vi "Main.vi"() -> ()   [LabVIEW 2018]
uses:
  Status.ctl
  Command.ctl
  SECM tip/Control 1.ctl
  SR865/SR865.ctl
  RBD9103/RBD9103.ctl
  GenericDataEvent/GenericEvent.ctl
  Zaber library/Zaber.ctl
  Zaber library/ZaberVariables.ctl
  Exec Action.ctl
  Actions.ctl
  Program Info.ctl
  Zaber library/Stage joystick buttons.ctl
  <vilib>/Analysis/baseanly.llb/Matrix Type of Inverse Matrix.ctl
  SR865/DataChannel.ctl
  <vilib>/Platform/TimedLoop/XDataNode/timing_clust.ctl
  <vilib>/Platform/TimedLoop/XDataNode/nitl_modes.ctl
  <vilib>/Platform/TimedLoop/XDataNode/wakeup.ctl
  <vilib>/DAQmx/write.llb/DAQmx Write (Digital Bool 1Line 1Point).vi
  <vilib>/Analysis/7linalg.llb/Solve Linear Equations (single right hand).vi
  <vilib>/Analysis/baseanly.llb/Solve Linear Equations By Cholesky.vi
  <vilib>/Analysis/baseanly.llb/Real Matrix to Compact Array.vi
  <vilib>/Analysis/baseanly.llb/Real Compact Tri-Matrix Linear Eqs.vi
  <vilib>/DAQmx/create/channels.llb/DAQmx Create Channel (DO-Digital Output).vi
  <vilib>/DAQmx/miscellaneous.llb/DAQmx Fill In Error Info.vi
  <vilib>/Analysis/7linalg.llb/Solve Linear Eqs (General).vi
  <vilib>/Analysis/7linalg.llb/Solve Linear Eqs (Gen, single right hand).vi
  <vilib>/Utility/file.llb/Write Delimited Spreadsheet (DBL).vi
  <vilib>/measure/maresamp.llb/Resample N Pairs of Arrays (single shot).vi
  <vilib>/Platform/TimedLoop/XDataNode/XDataNode.xnode
  <vilib>/Analysis/NI_AALBase.lvlib
  <vilib>/Analysis/NI_AALPro.lvlib
  <vilib>/Platform/TimedLoop/XDataNode/XDNodeRunTimeDep.lvlib
  <vilib>/measure/NI_MAPro.lvlib
panel:
  in  "Pre-scan time, s":dbl
  in  "Landing dwell, s":dbl
  out "MS dwell":bool
  in  "BtnSaveSegLineRecords":bool
  out "relative main end":dbl
  out "relative main start":dbl
  out "segLines":dbl[][](array[numeric])
  out "Current step idx":i32
  out "CC stop":bool
  out "CC start":bool
  out "Strip motion \nposition":dbl
  out "Main motion\nstart position":dbl
  out "Main motion \nend position":dbl
  in  "sample DLADS prediction":string="C:\\Users\\Lab Admin\\Desktop"
  out "Latest step idx":i32
  out "Wait to iterate ?":bool
  out "Iterate ?":bool
  in  "BtnDLADS":bool
  in  "BtnSaveScanConfig":bool
  in  "Com error":bool
  out "Z Zaber":T1={"Serial port handle"="", "Axis"="", "Controller #"=0, "Min position"=0.0, "Max position"=0.0, "Min velocity"=0.0, "Max velocity"=0.0, "Firmware"="", "Device ID"=0, "Variable event"=refnum, "Variable ref"=refnum, "Resolution, usteps/step"=0, "Serial port semaphore"=refnum, "Joystick buttons"={"MinDir"=1, "MaxDir"=2, "MedSpeed"=5, "HighSpeed"=6}} {"Joystick buttons"."HighSpeed" min=1 max=25 step=1; "Joystick buttons"."MedSpeed" min=1 max=25 step=1; "Joystick buttons"."MaxDir" min=1 max=25 step=1; "Joystick buttons"."MinDir" min=1 max=25 step=1}
  out "Loop time":u32
  out "BtnLoopWasLate":bool caption="Loop was late"
  out "MS ever Trig?":bool=TRUE
  out "MS start":u32=518275974
  out "LineMotion":bool=TRUE caption="Line motion"
  out "LineNumber":u32=2
  out "dt":dbl
  out "t0":dbl
  out "MotionStartTime":u32 caption="Line start time"
  out "Keyence":T4={"Serial port sem"=refnum, "Serial port handle"="", "Baud rate"=9600}
  in  "Keyence COM port":refnum<visa-resource-name>="COM4"
  out "SICM tip":refnum<vi>
  out "Stop tune SICM":refnum<user-event>
  out "RBD9103":T5
  in  "RBD9103 COM":refnum<visa-resource-name>="COM4"
  in  "SR865":refnum<visa-resource-name>="USB0::0xB506::0x2000::003539::INSTR"
  out "SR865":T6
  in  "TabMethods":T7(tab)=enum."Shear force sensor"
  in  "TabPlanes":enum32{"Simple plane", "3 point plane"}(tab)
  in  "SPZEndPosition":dbl=5.0 caption="Z end" min=0.0 max=25.0 format="%#.4f"
  out "PlaneZ3":dbl caption="Z3" min=0.0 max=25.0 format="%#.4f"
  out "PlaneY3":dbl caption="Y3" min=0.0 max=25.0 format="%#.4f"
  out "PlaneX3":dbl=20.0000235 caption="X3" min=0.0 max=25.0 format="%#.4f"
  out "PlaneZ2":dbl caption="Z2" min=0.0 max=25.0 format="%#.4f"
  out "PlaneY2":dbl=10.00001175 caption="Y2" min=0.0 max=25.0 format="%#.4f"
  out "PlaneX2":dbl caption="X2" min=0.0 max=25.0 format="%#.4f"
  out "PlaneZ1":dbl caption="Z1" min=0.0 max=25.0 format="%#.4f"
  out "PlaneY1":dbl caption="Y1" min=0.0 max=25.0 format="%#.4f"
  out "PlaneX1":dbl caption="X1" min=0.0 max=25.0 format="%#.4f"
  in  "BtnPlaneSetPoint3":bool caption="Set Z out position"
  in  "BtnPlaneSetPoint1":bool
  in  "BtnPlaneSetPoint2":bool caption="Set Z out position"
  out "PlaneZx":dbl caption="Zx" min=0.0 max=25.0 format="%#.4f"
  out "PlaneZy":dbl caption="Zy" min=0.0 max=25.0 format="%#.4f"
  in  "BtnPZStepType":bool caption="Z step type"
  out "PZJumps":u32=600 caption="Z jumps" min=1
  out "PZJump":u32 caption="Z jump"
  out "PZRealStep":dbl=0.0049999802083333334 caption="Z real step" format="%#.4f"
  out "PZStepTimeRb":dbl=0.03399378902730266 caption="Z step time, s" format="%#.1f"
  out "Distance":dbl=2257.881405072176 caption="Distance, um" format="%#.1f"
  out "StartDistance":dbl caption="Start distance, um" format="%#.1f"
  out "MoveDistance":dbl caption="Move distance, um" format="%#.1f"
  out "RealMoveDistance":dbl caption="Real move distance, um" format="%#.1f"
  in  "ZFactor":dbl=20.0 caption="Sensor/Z motion factor" min=0.0 max=25.0 format="%#.4f"
  in  "ZMinToMoveDistanceancy":dbl=5.0 caption="Min to move distance, um" min=0.0 format="%#.4f"
  in  "ZMaxToMoveDistance":dbl=50.0 caption="Max to move distance, um" min=0.0 format="%#.4f"
  in  "BtnShearForceTune":bool
  out "SFMWorkingLevel":dbl=7.0 caption="Working level, V" min=0.0 max=25.0 step=0.01 format="%#.4f"
  in  "SFMShiftFromAirLevel":dbl=-0.5 caption="Shift from Air level, V" min=0.0 max=25.0 step=0.01 format="%#.4f"
  in  "SFMSlope":dbl=-0.007 caption="Slope, mm/V" min=0.0 max=25.0 step=0.01 format="%#.4f"
  in  "SFMAirErrorLevel":dbl=0.05 caption="Air error level, V" min=0.0 max=25.0 step=0.01 format="%#.4f"
  out "SFMAirError":bool caption="Air level changed"
  in  "SFMLoopTime":i32=10 caption="Loop time, ms"
  out "CurrentAirLevel":dbl=7.198980893447915 caption="Current air level, V" format="%0.2f"
  in  "SFMStayRange":dbl=0.01 caption="Stay range, V"
  out "ShF loop time":u32
  out "Amp dead time":u32
  out "Read position":u32
  in  "SIMStayRange":dbl=0.01 caption="Stay range, V"
  out "BtnSIMLoopWasLate":bool caption="Loop was late"
  out "SIMCurrentLevel":dbl=7.198980893447915 caption="Current air level, V" format="%0.4g"
  in  "SIMLoopTime":i32=10 caption="Loop time, ms" format="%.4g"
  out "SIMAirError":bool caption="Air error"
  in  "SIMAirErrorLevel":dbl=0.05 caption="Air error level, V" min=0.0 max=25.0 step=0.01 format="%#.4g"
  in  "SIMAirLevelSp":dbl=7.22 caption="Air level, V" min=0.0 max=25.0 step=0.01 format="%#.4g"
  in  "SIMWorkingLevel":dbl=7.0 caption="Working level,V" min=0.0 max=25.0 step=0.01 format="%#.4g"
  out "Position, mm":dbl
  out "PositionRb":dbl caption="Position, mm"
  out "Calculated position":dbl
  out "Value, nA":dbl
  out "LineTimeInSec":dbl=20.396273416381593 caption="Line time, s" format="%#.4f"
  out "LineError":dbl=396.27341638159305 caption="Line error, um" format="%#.1f"
  out "LineTimeError":dbl=0.3962734163815931 caption="Line time error, s"
  out "LineStraightTime":dbl=20.0 caption="Line straight time, s"
  in  "ZStep":dbl=0.005 caption="Z step, mm" min=1e-07 max=25.0 step=0.01 format="%#.4f"
  out "RunRef":refnum<vi>
  out "Dialog3StagesRef":refnum<vi>
  in  "Call type":enum16{"Dynamic", "Static"}(ring)=enum."Static"
  out "Stop tune ShFrc":refnum<user-event>
  out "Tune ShFrc":refnum<vi>
  in  "Baud rate (9600 or 115200)":u32=9600
  in  "Z stage":refnum<visa-resource-name>="COM7"
  in  "X&Y stages":T8="COM6"
  in  "BtnSaveZToFile":bool=TRUE
  in  "BtnZ+":bool
  in  "BtnZ-":bool
  out "ProfilePlot":dbl[][](graph) caption="Profile"
  out "ZPositionPlot":cluster{cluster{dbl, dbl}[]}[](graph) caption="Z position"
  in  "LineZData":cluster{cluster{dbl, dbl}[]}[](array[cluster])=[{[]}, {[]}, {[]}]
  out "Profile array":cluster{dbl[], dbl[]}[](array[cluster])
  in  "Method":T9(ring)=enum."3 point plane"
  in  "BtnMeasurementPause":bool
  in  "BtnSave":bool
  in  "Command":T10=enum."None"
  in  "Status":T11
  out "StripStepRb":dbl caption="Strip step" format="%#.4f"
  out "StripLineRb":u32 caption="Strip line"
  in  "StripLines":u32=2 caption="Strip lines" min=1
  out "YStageType":enum16{"Main motion", "Strip motion"}(ring)=enum."Strip motion" caption="Type motion"
  in  "XStageType":enum16{"Main motion", "Strip motion"}(ring) caption="Type"
  out "ZOutPosition":dbl=9.67997175 caption="Z out" format="%#.4f"
  in  "BtnSetZOutPosition":bool caption="Set Z out position"
  out "ZStartPosition":dbl=9.67997175 caption="Z start" min=0.0 max=25.0 format="%#.4f"
  in  "BtnMeasurement":bool
  in  "BtnSetZStartPosition":bool
  in  "BtnExit":bool
  out "LineTimeInMin":dbl=0.33993789027302657 caption="Line time, min" format="%#.3f"
  in  "MSDwellTimeInSec":dbl=15.0 caption="QTOF ready, s" format="%#.1f"
  in  "YEndPosition":dbl=7.0 caption="End  position, mm" min=0.0 max=25.40003175 format="%#.4f"
  in  "YStartPosition":dbl=5.0 caption="Start position, mm" min=0.0 max=25.40003175 format="%#.4f"
  in  "Velocity":dbl=0.020091796874999998 caption="Velocity, mm/s" min=0.000446484375 max=3.5 format="%#.4g"
  in  "XEndPosition":dbl=20.0 caption="End position, mm" min=0.0 max=50.800015875 format="%#.4f"
  in  "XStartPosition":dbl=15.0 caption="Start position, mm" min=0.0 max=50.800015875 format="%#.4f"
  out "Current Time":timestamp format="%<%I:%M:%S %p>T"
  # "X stage"
  # "Z stage"
  # "Y stage"
  # "Main motion"
  # "Strip motion"
  # "Timing"
  # "Keyence reading time 50 ms ; 115200 bod"
  # "doesn't work in Line"
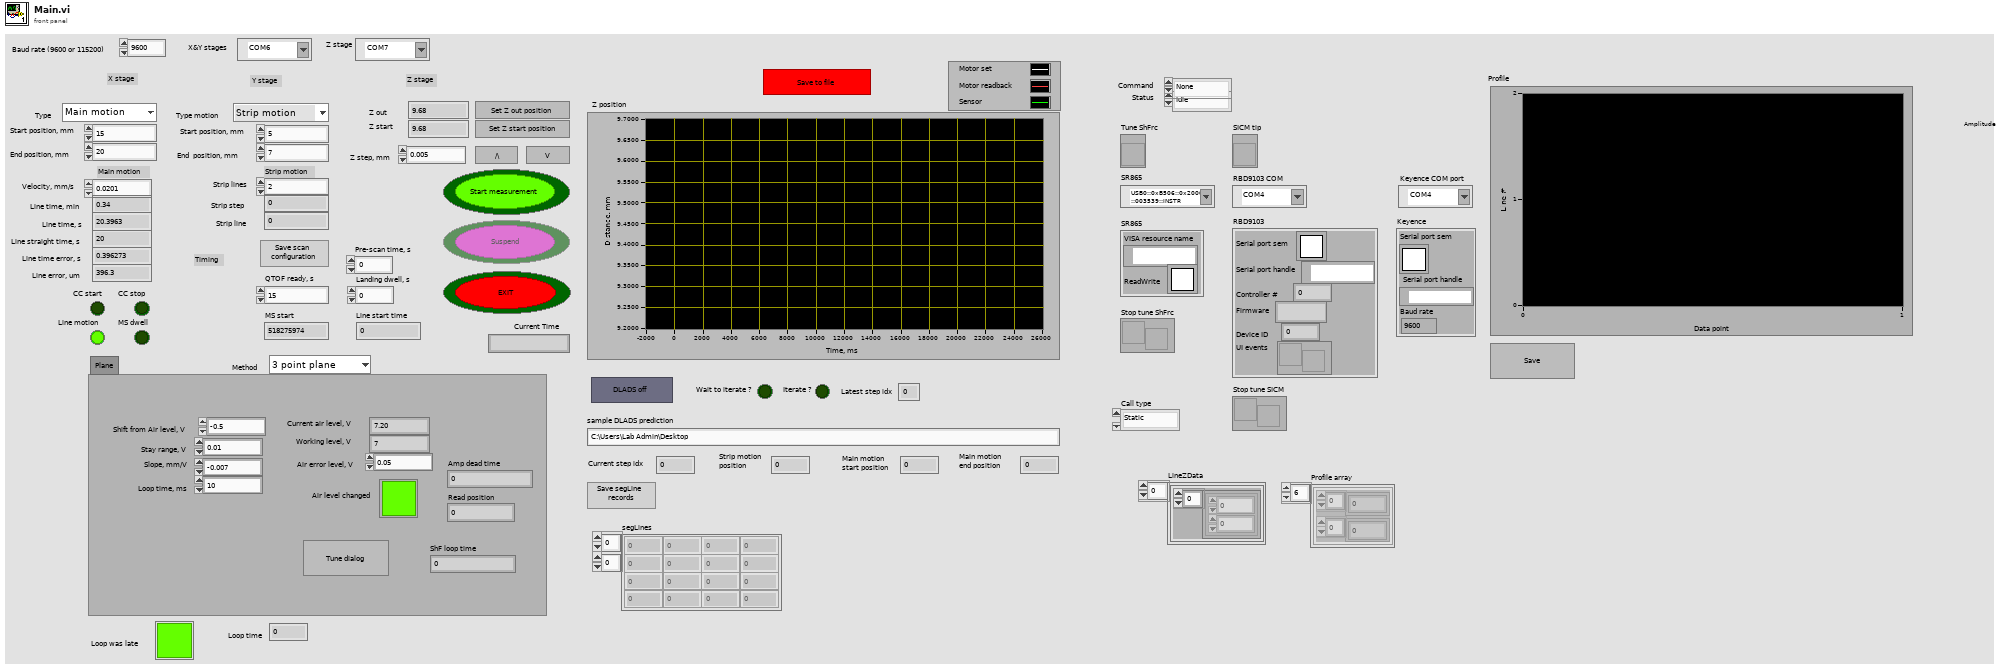
[diagram p1: front panel]
types:
  T1 = typedef "Zaber.ctl" = cluster{"Serial port handle":refnum<visa-resource-name>, "Axis":string, "Controller #":u8, "Min position":dbl, "Max position":dbl, "Min velocity":dbl, "Max velocity":dbl, "Firmware":string, "Device ID":i32, "Variable event":T2, "Variable ref":refnum<data-value>, "Resolution, usteps/step":i32, "Serial port semaphore":T3, "Joystick buttons":cluster{"MinDir":i32, "MaxDir":i32, "MedSpeed":i32, "HighSpeed":i32}}
  T2 = typedef "GenericEvent.ctl" = refnum<user-event>
  T3 = typedef "Semaphore RefNum" = refnum<k1>
  T4 = cluster{"Serial port sem":T3, "Serial port handle":refnum<visa-resource-name>, "Baud rate":u32}
  T5 = typedef "RBD9103.ctl" = cluster{"Serial port sem":T3, "Serial port handle":refnum<visa-resource-name>, "Controller #":u8, "Firmware":string, "Device ID":i32, "UI events":T2}
  T6 = typedef "SR865.ctl" = cluster{"VISA resource name":refnum<visa-resource-name>, "ReadWrite":T3}
  T7 = enum32{"Plane", "Keyence sensor", "Shear force sensor", "SICM sensor"}
  T8 = typedef "Control 1.ctl" = refnum<visa-resource-name>
  T9 = enum16{"Simple plane", "3 point plane", "Keyence sensor", "Shear force sensor", "SICM sensor", "Surface image by Keyence"}
  T10 = typedef "Command.ctl" = enum16{"Start", "Suspend", "Resume", "Stop", "Finish", "None"}
  T11 = typedef "Status.ctl" = enum16{"Idle", "Working", "Pause", "Stopping"}
  T12 = typedef "Program Info.ctl" = cluster{"Placeholder":bool}
  T13 = typedef "Exec Action.ctl" = cluster{"Action":T14, "1":bool, "2":bool, "3":bool}
  T14 = typedef "Actions.ctl" = enum16{"SW Init", "HW Init - Zaber", "HW Init - DO", "Init Asynch Vis", "Set Motion Params", "Set Zout Pos", "Set Zstart Pos", "Step Z", "Method close - Shear force", "Method close - SICM", "Method close - Keyence", "Method UI and HW init", "Tune Shear Force", "Plane Set Point 1", "Plane Set Point 2", "Plane Set Point 3", "Calculate Plane", "Scan UI", "Scan Ctrl", "Handle DLADS", "XY and Sensor Init", "Z Init", "MS Trig", "Line Motion", "Z Exit Ctrl", "MS Complete", "Pause Check Ctrl", "Shift Data", "Plot Profile", "Save Scan Config", "Save Profile Text File", "Wait (ms)", "Get Time", "HW Close - Zaber", "HW Close - DO", "Error", "Exit", "Shutdown Ctrl"}
  T15 = enum8{"Enabled", "Disabled", "Disabled and Grayed Out"}
  T16 = enum32{"Invalid", "Standard", "Closed", "Hidden", "Minimized", "Maximized"}
  T17 = typedef "NI_AALBase.lvlib/Matrix Type of Inverse Matrix.ctl" = enum32{"General", "Positive Definite", "Lower Triangular", "Upper Triangular"}
  T18 = typedef "XDNodeRunTimeDep.lvlib/timing_clust.ctl" = cluster{"Expected End [f-1]":u64, "Actual End [f-1]":u64, "Finished Late? [f-1]":bool, "Expected End [i-1]":u64, "Actual End [i-1]":u64, "Finished Late? [i-1]":bool, "Expected Start [i]":u64, "Actual Start [i]":u64, "Expected Start [f]":u64, "Actual Start [f]":u64, "Source Name":string, "Structure Name":string, "Period":i64, "Deadline":i64, "Offset":i64, "Start":i64, "Priority":i32, "Timeout":i32, "Mode":T19, "Wakeup Reason":T20, "Error":errorcluster, "Source Type":string, "Secondary Source Type":string, "Global End Time":u64, "Global Start Time":u64, "Frame Duration":u64, "Iteration Duration":u64, "Assigned CPU":i32, "I/O Scan Engine Mode":u32}
  T19 = typedef "XDNodeRunTimeDep.lvlib/nitl_modes.ctl" = enum32{"No Change", "Process missed periods, maintain original phase", "Discard missed periods, maintain original phase", "Process missed periods, ignore original phase", "Discard missed periods, ignore original phase"}
  T20 = typedef "XDNodeRunTimeDep.lvlib/wakeup.ctl" = enum32{"Normal", "Aborted", "Asynchronous wakeup", "Timing source error", "Timed loop error", "Timeout"}
  T21 = enum16{"open", "replace", "create", "open or create", "replace or create", "replace or create with confirmation"}
  T22 = typedef "Stage joystick buttons.ctl" = cluster{"MinDir":i32, "MaxDir":i32, "MedSpeed":i32, "HighSpeed":i32}
  T23 = typedef "Joystick event.ctl" = refnum<user-event>
  T24 = typedef "DataChannel.ctl" = u16
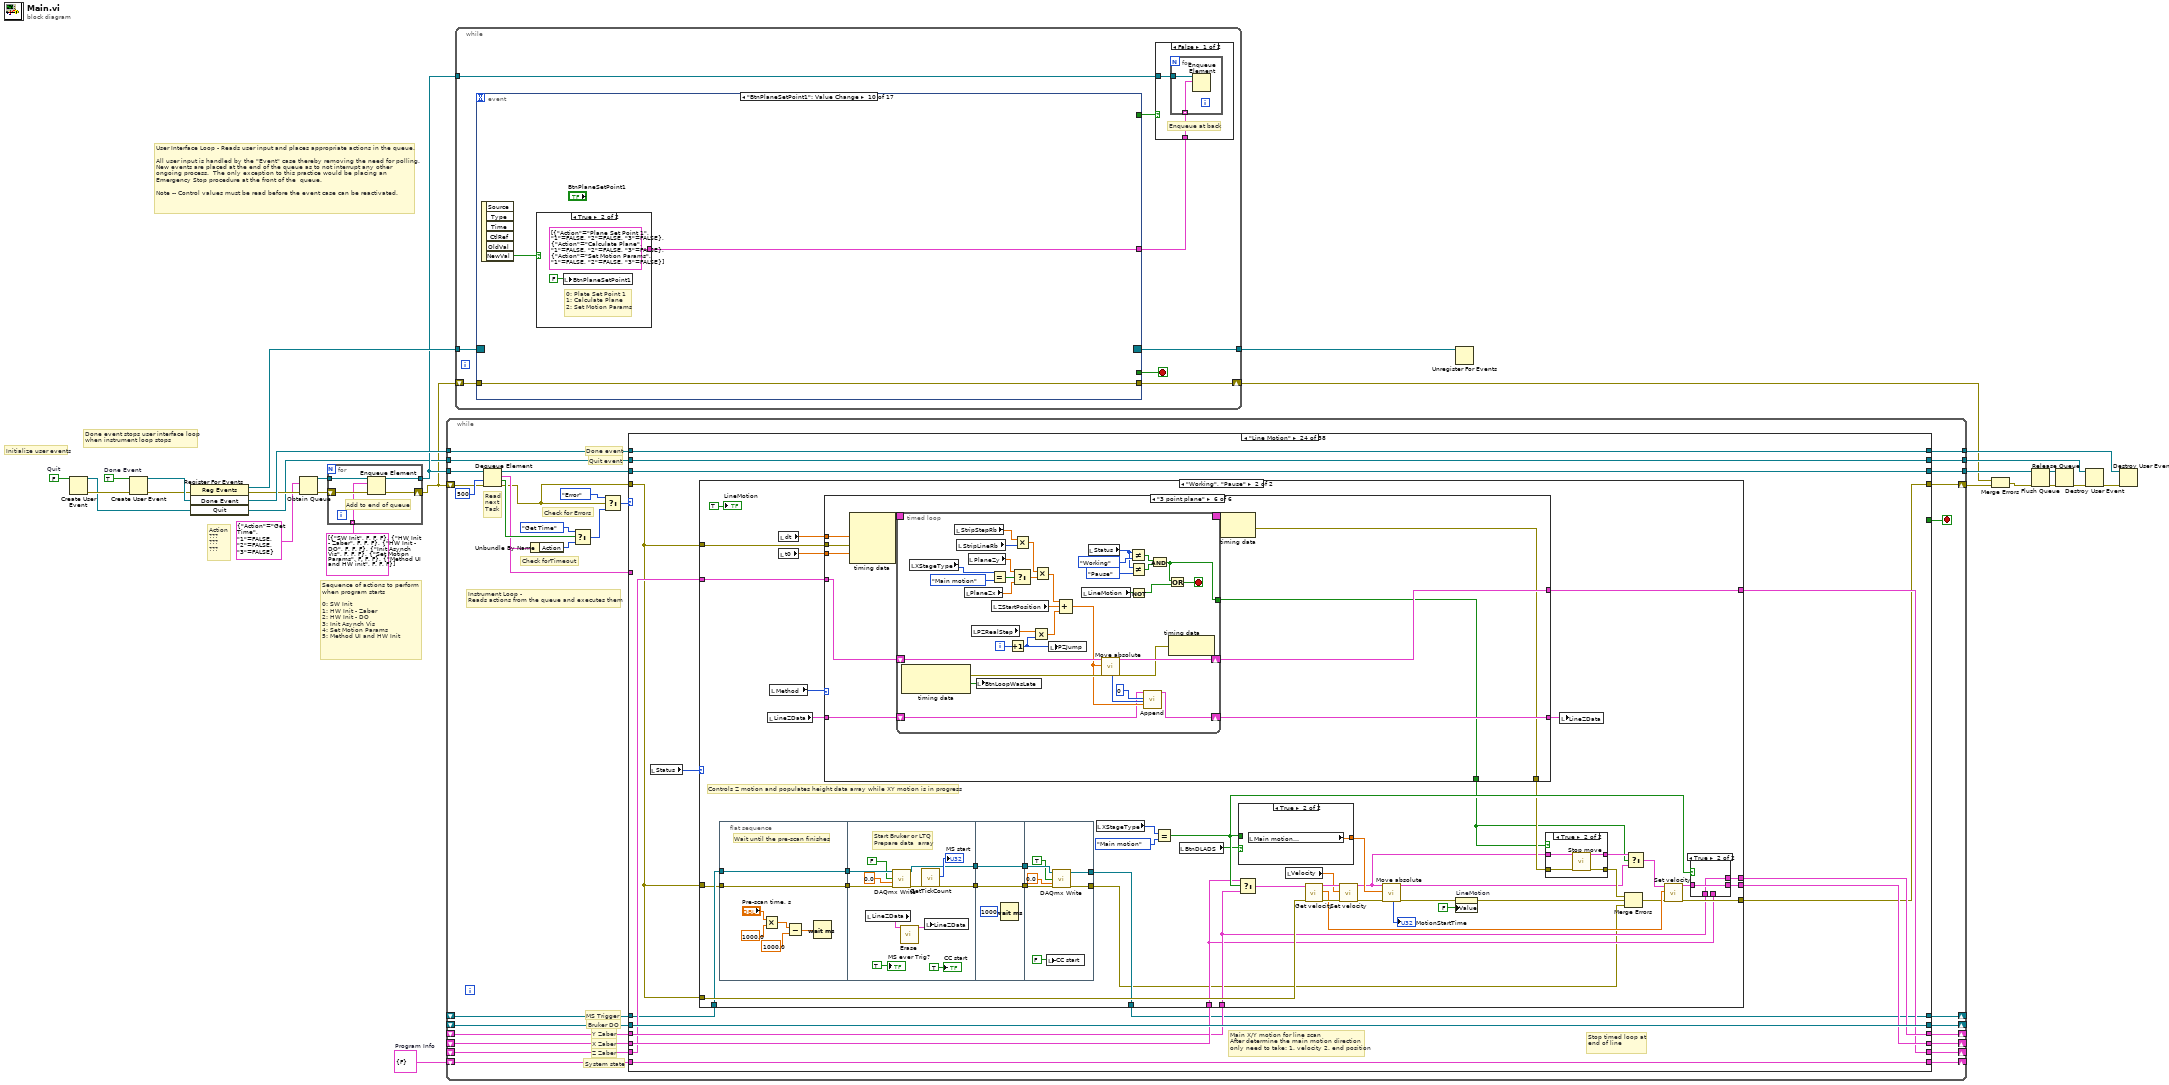
[diagram p0: block diagram]
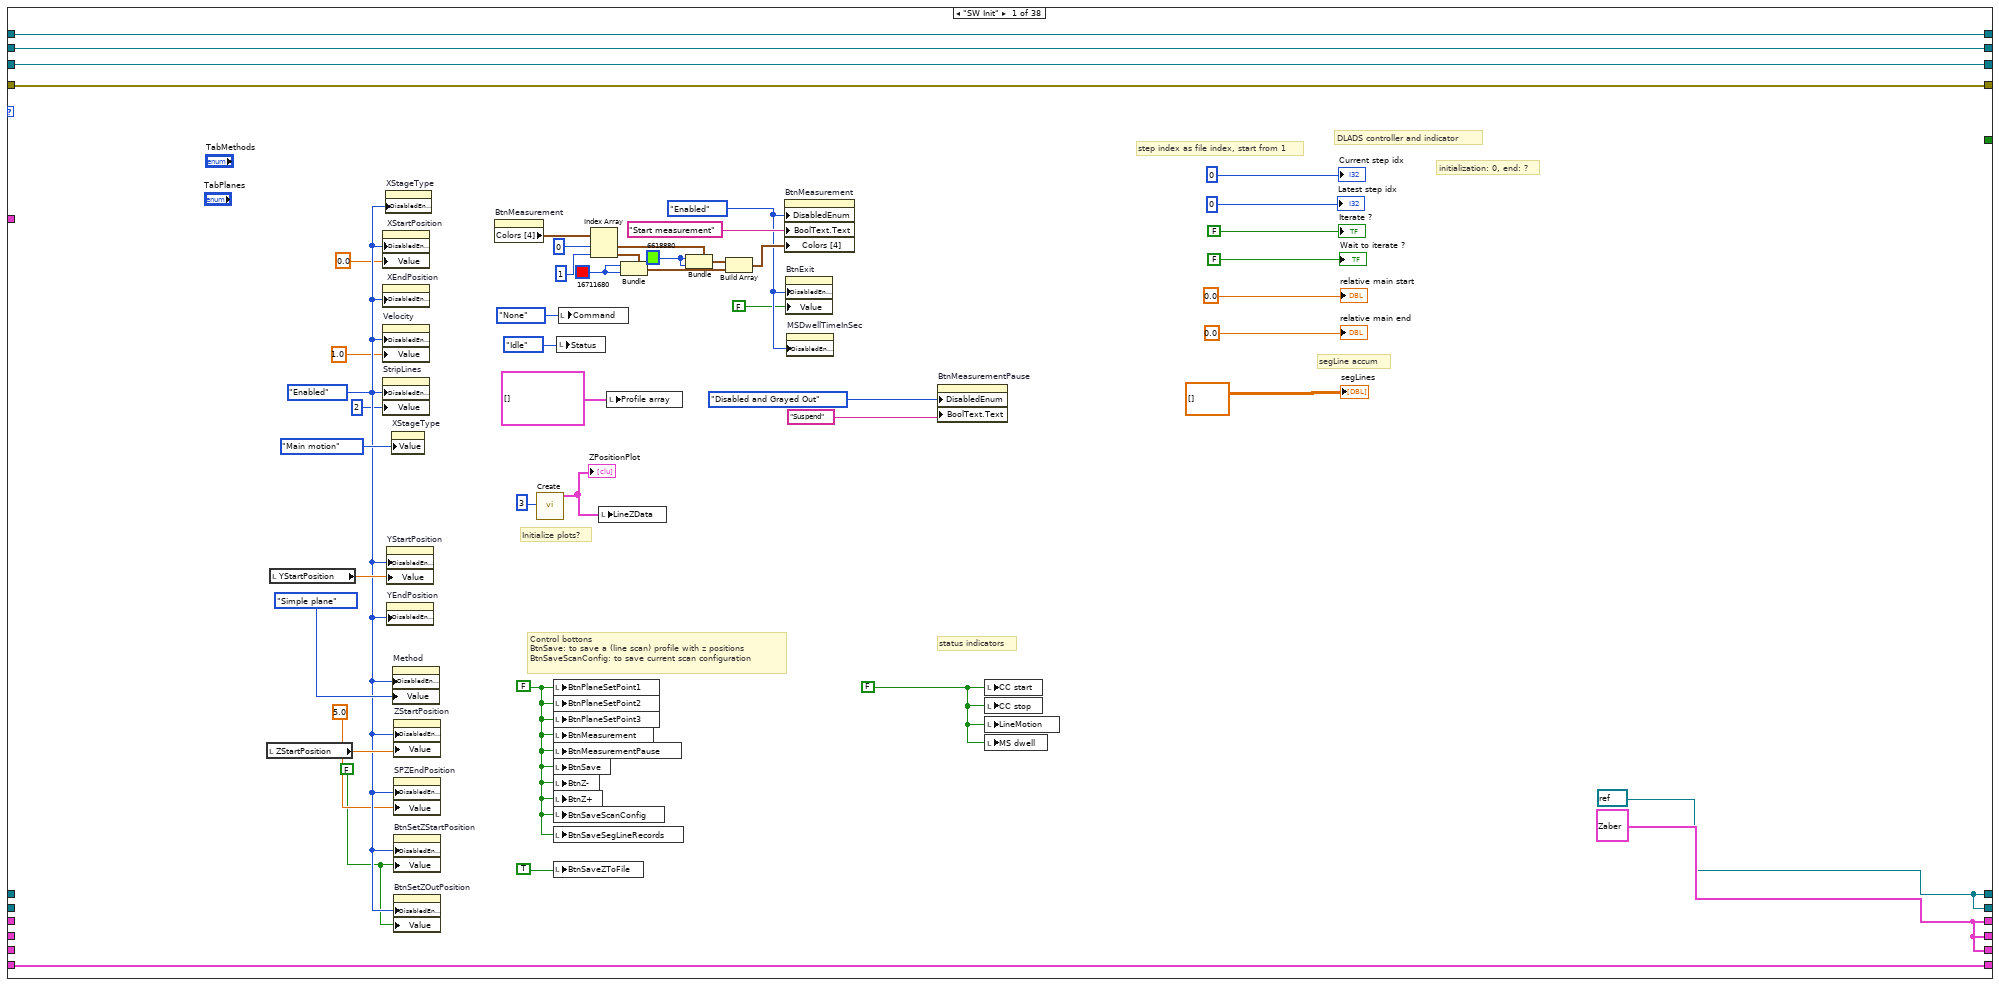
[diagram p2: hidden frame]
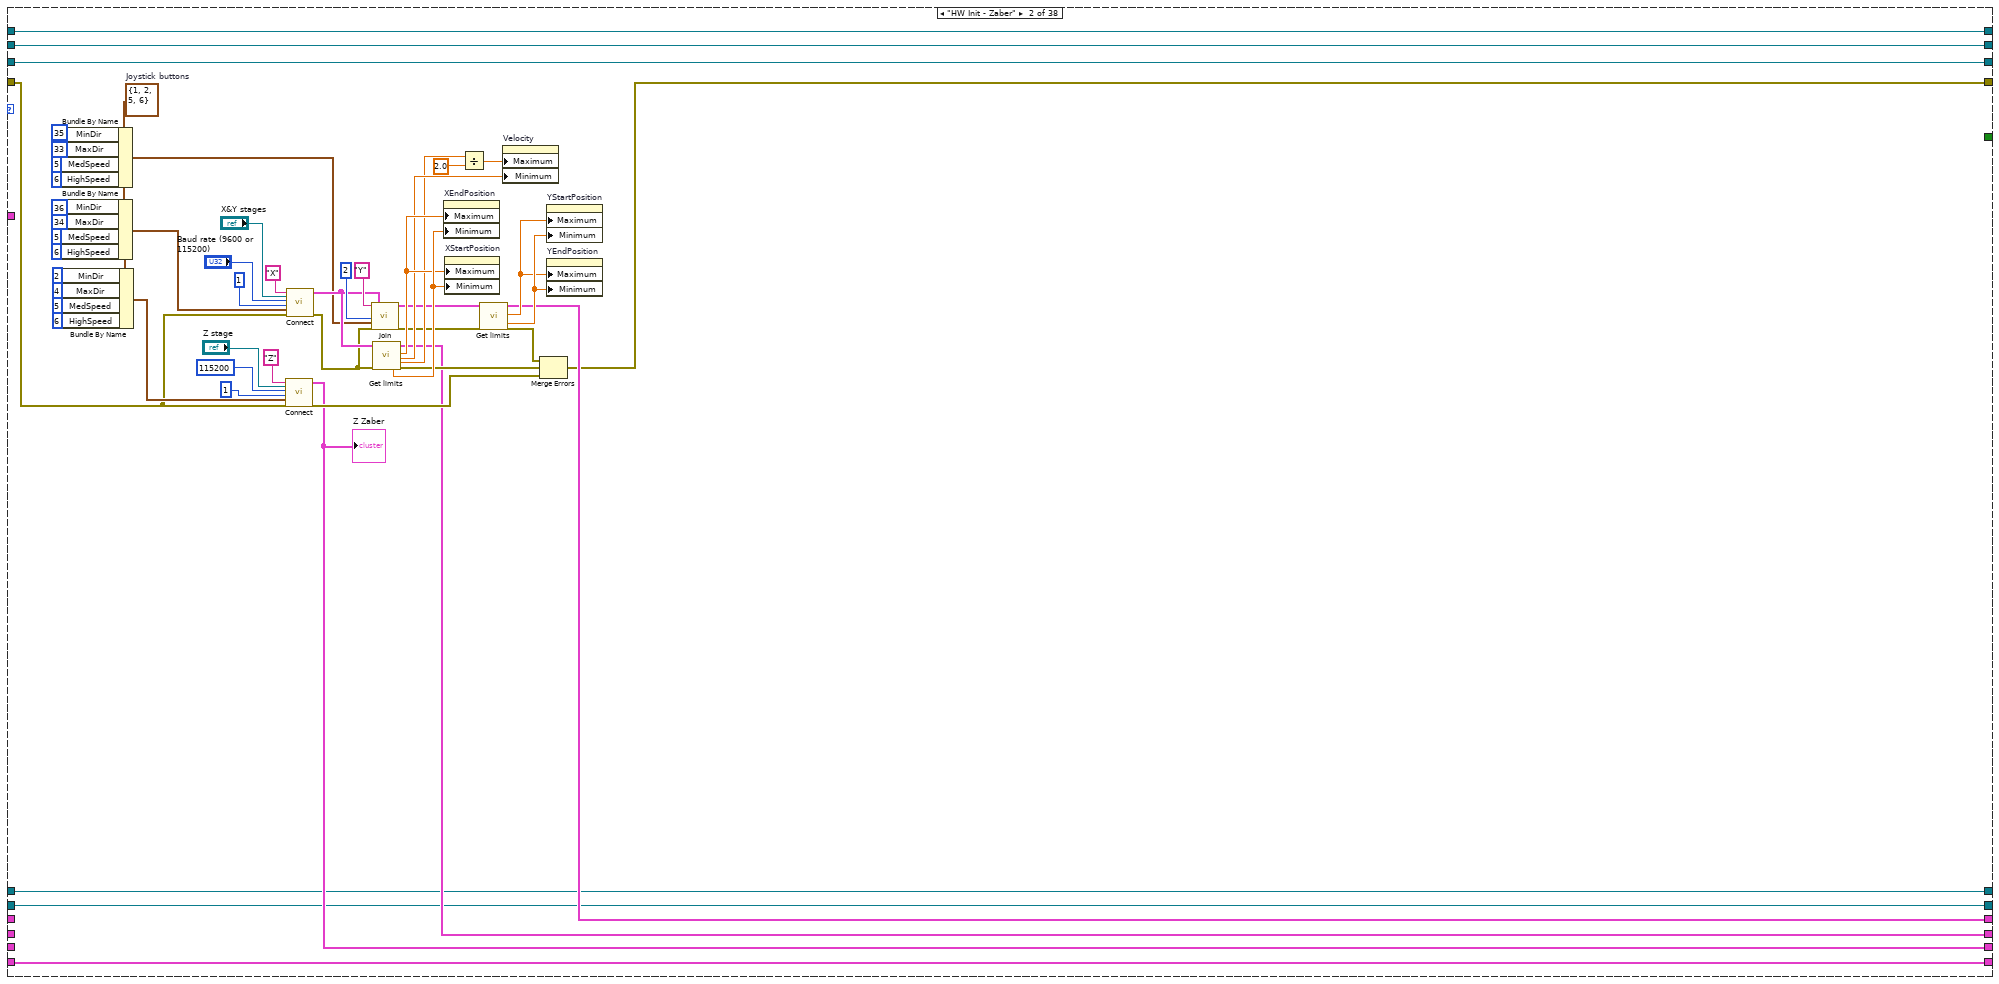
[diagram p3: hidden frame]
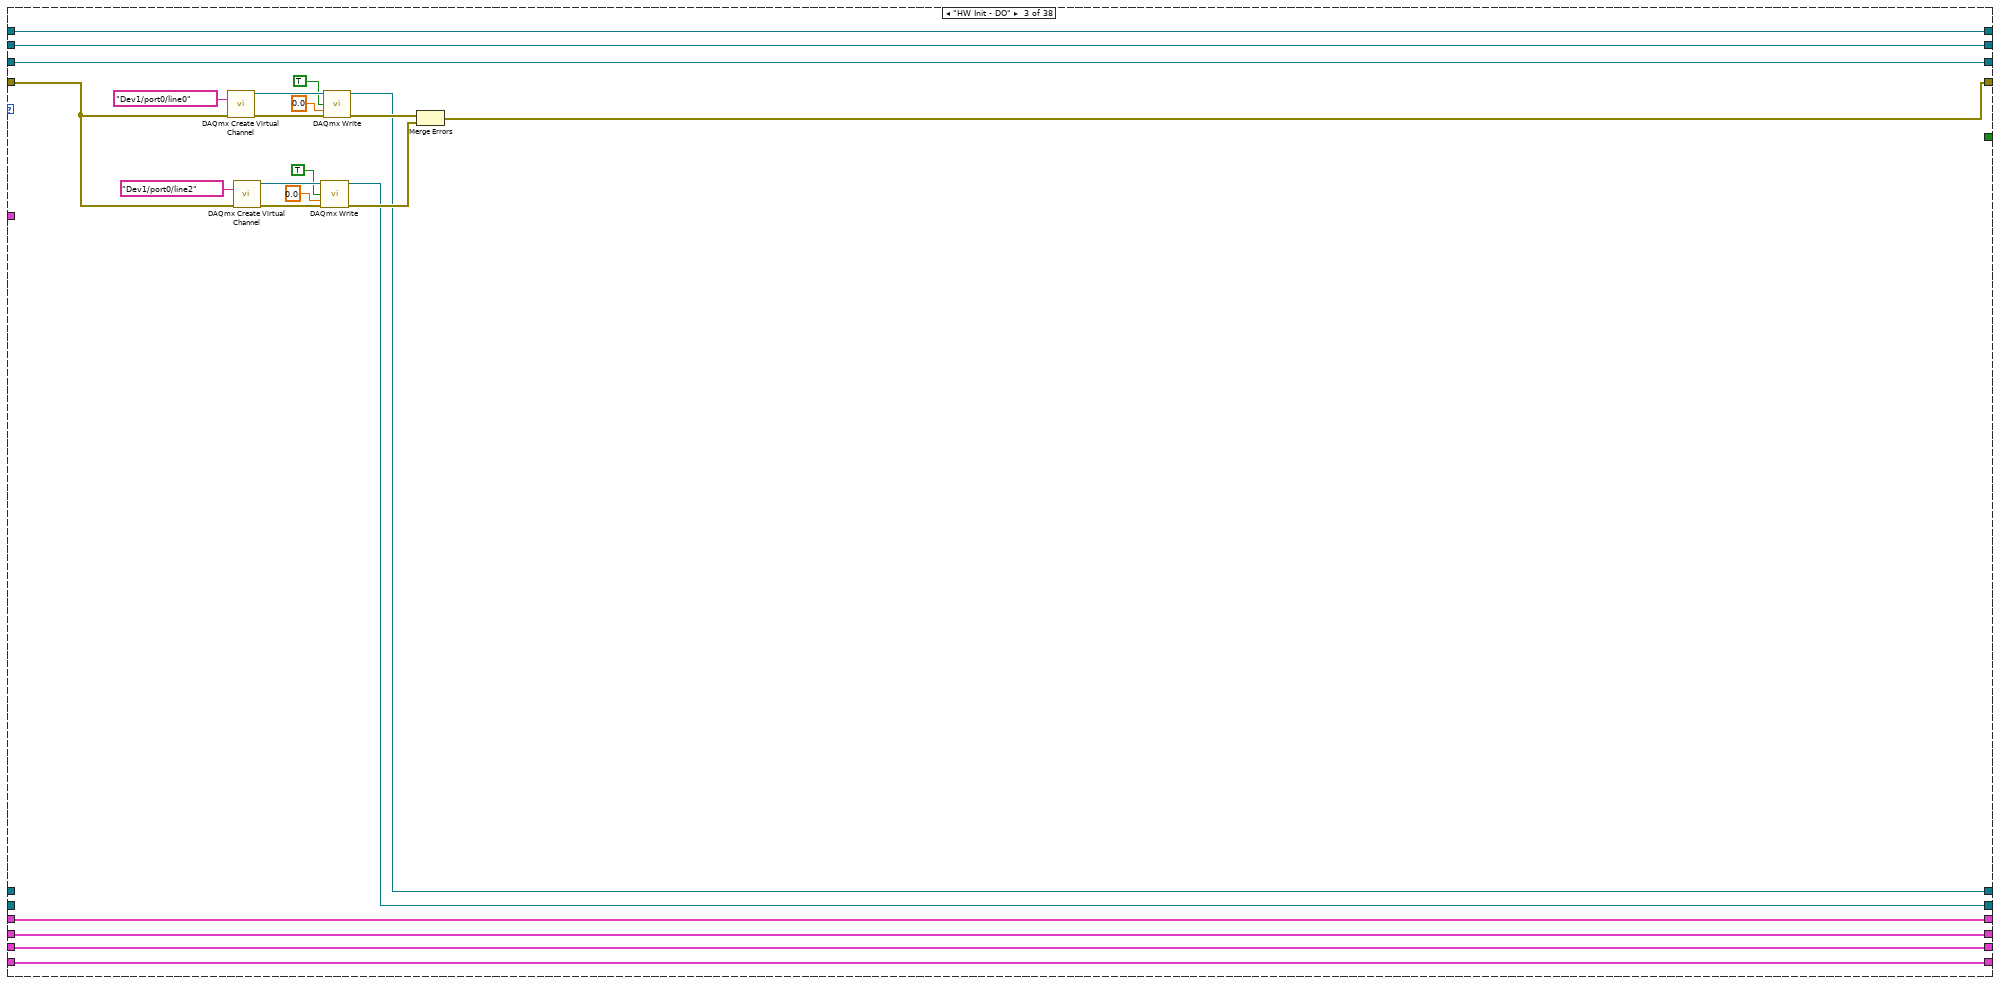
[diagram p4: hidden frame]
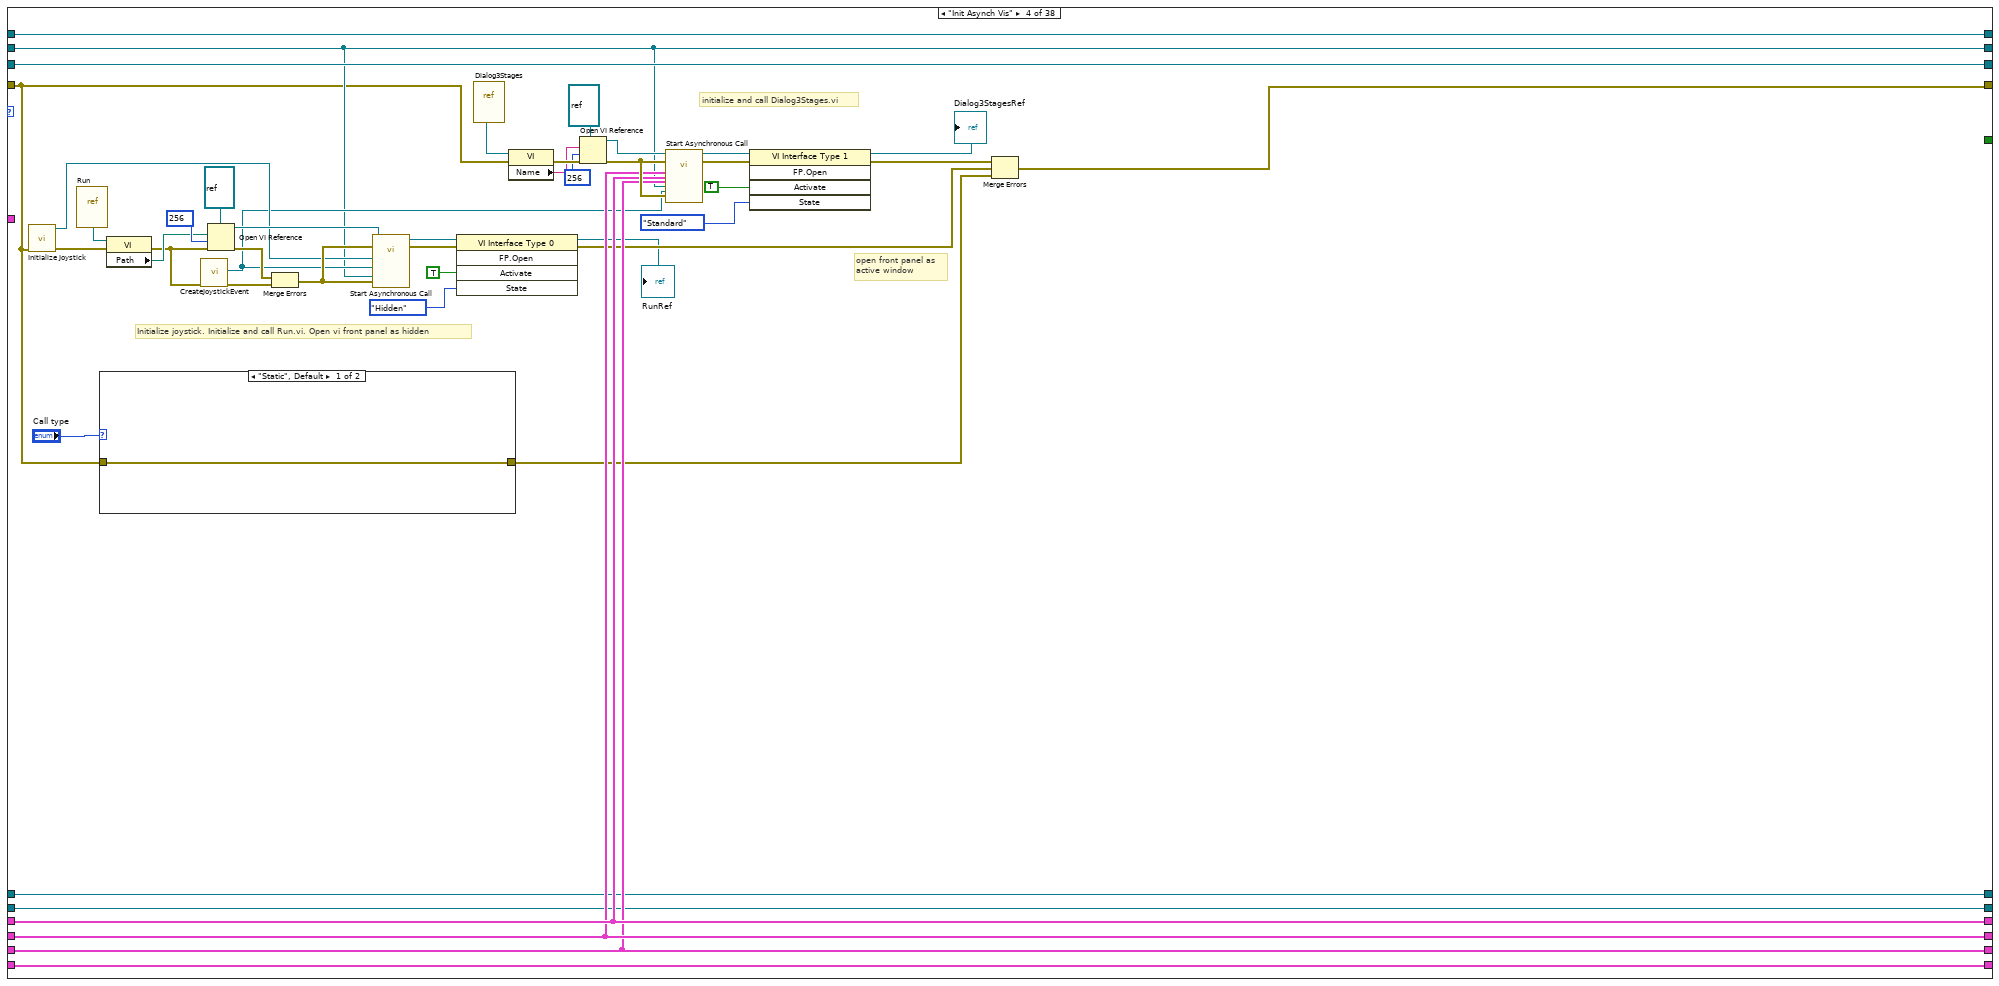
[diagram p5: hidden frame]
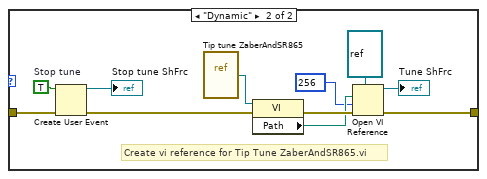
[diagram p6: hidden frame]
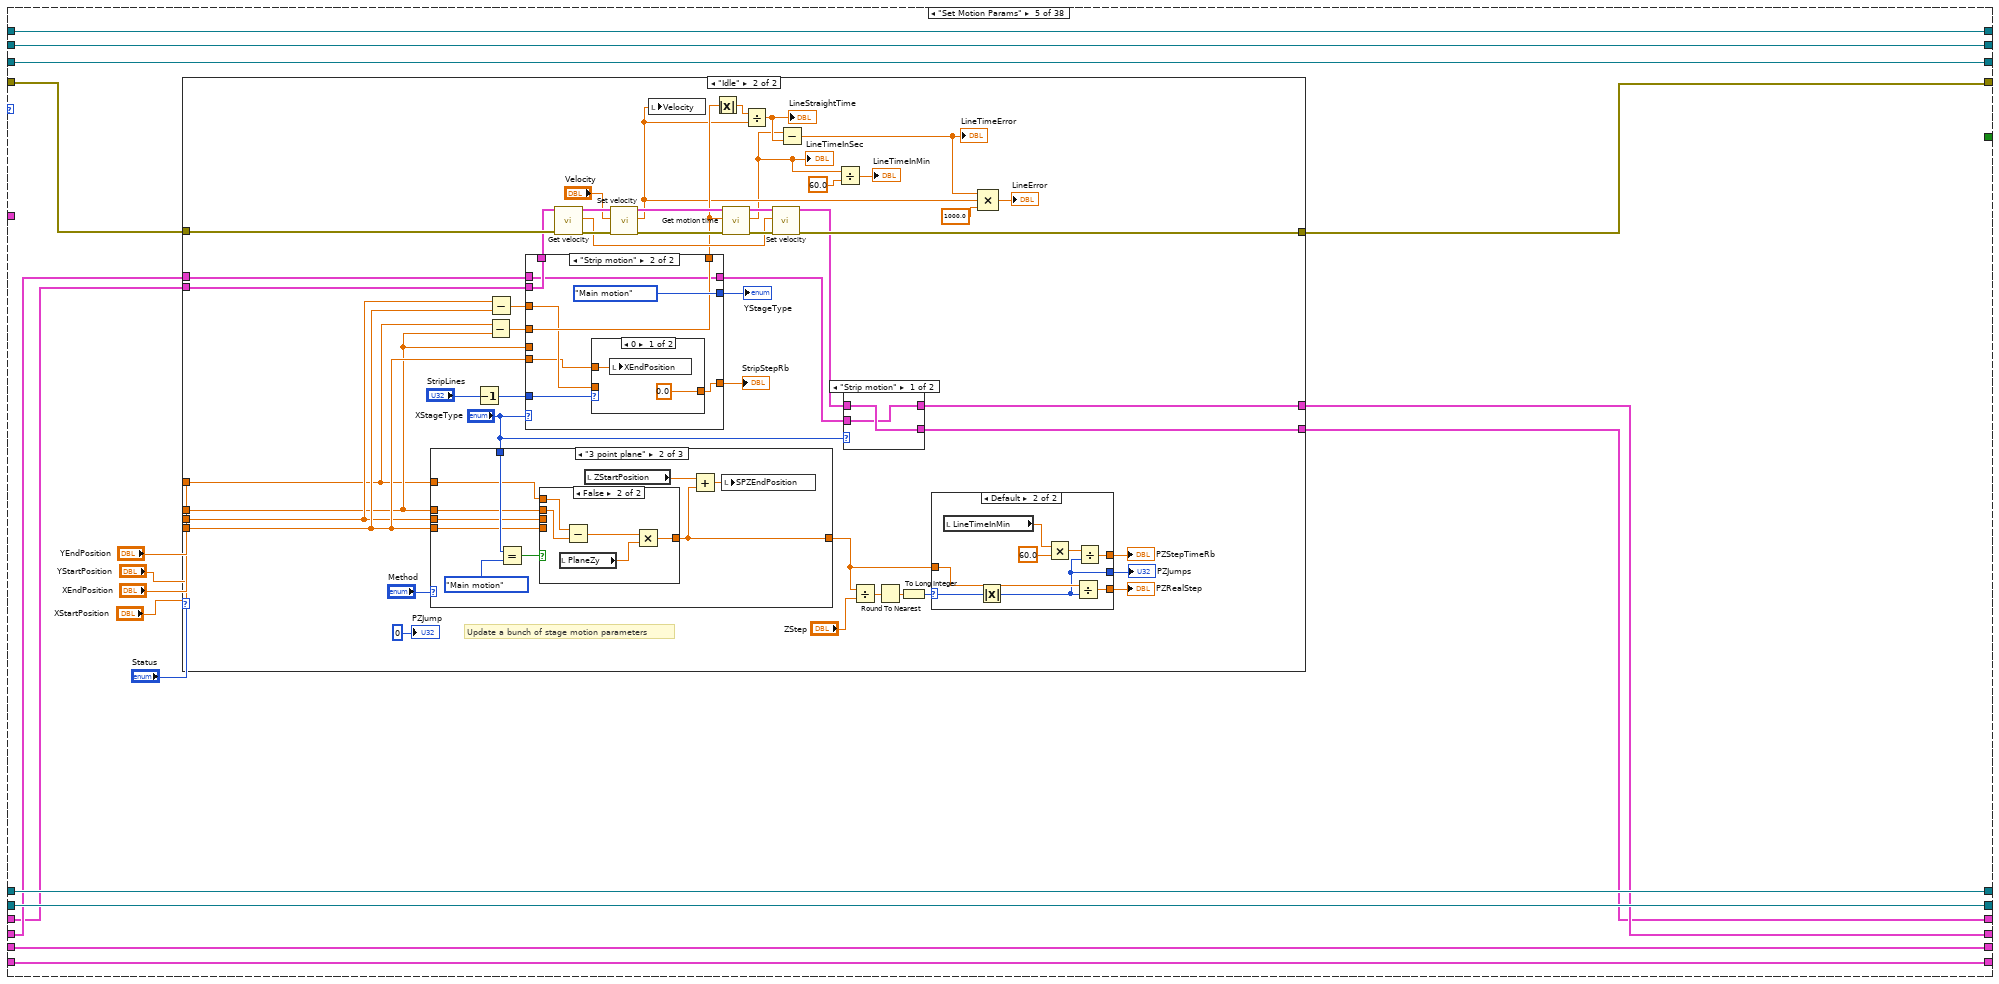
[diagram p7: hidden frame]
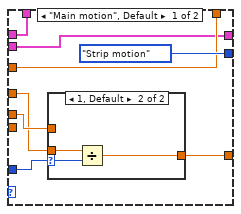
[diagram p10: hidden frame]
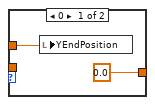
[diagram p11: hidden frame]
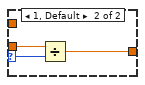
[diagram p12: hidden frame]
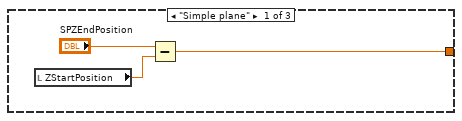
[diagram p13: hidden frame]
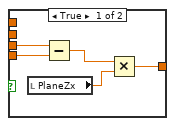
[diagram p14: hidden frame]
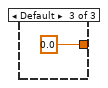
[diagram p15: hidden frame]
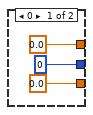
[diagram p16: hidden frame]
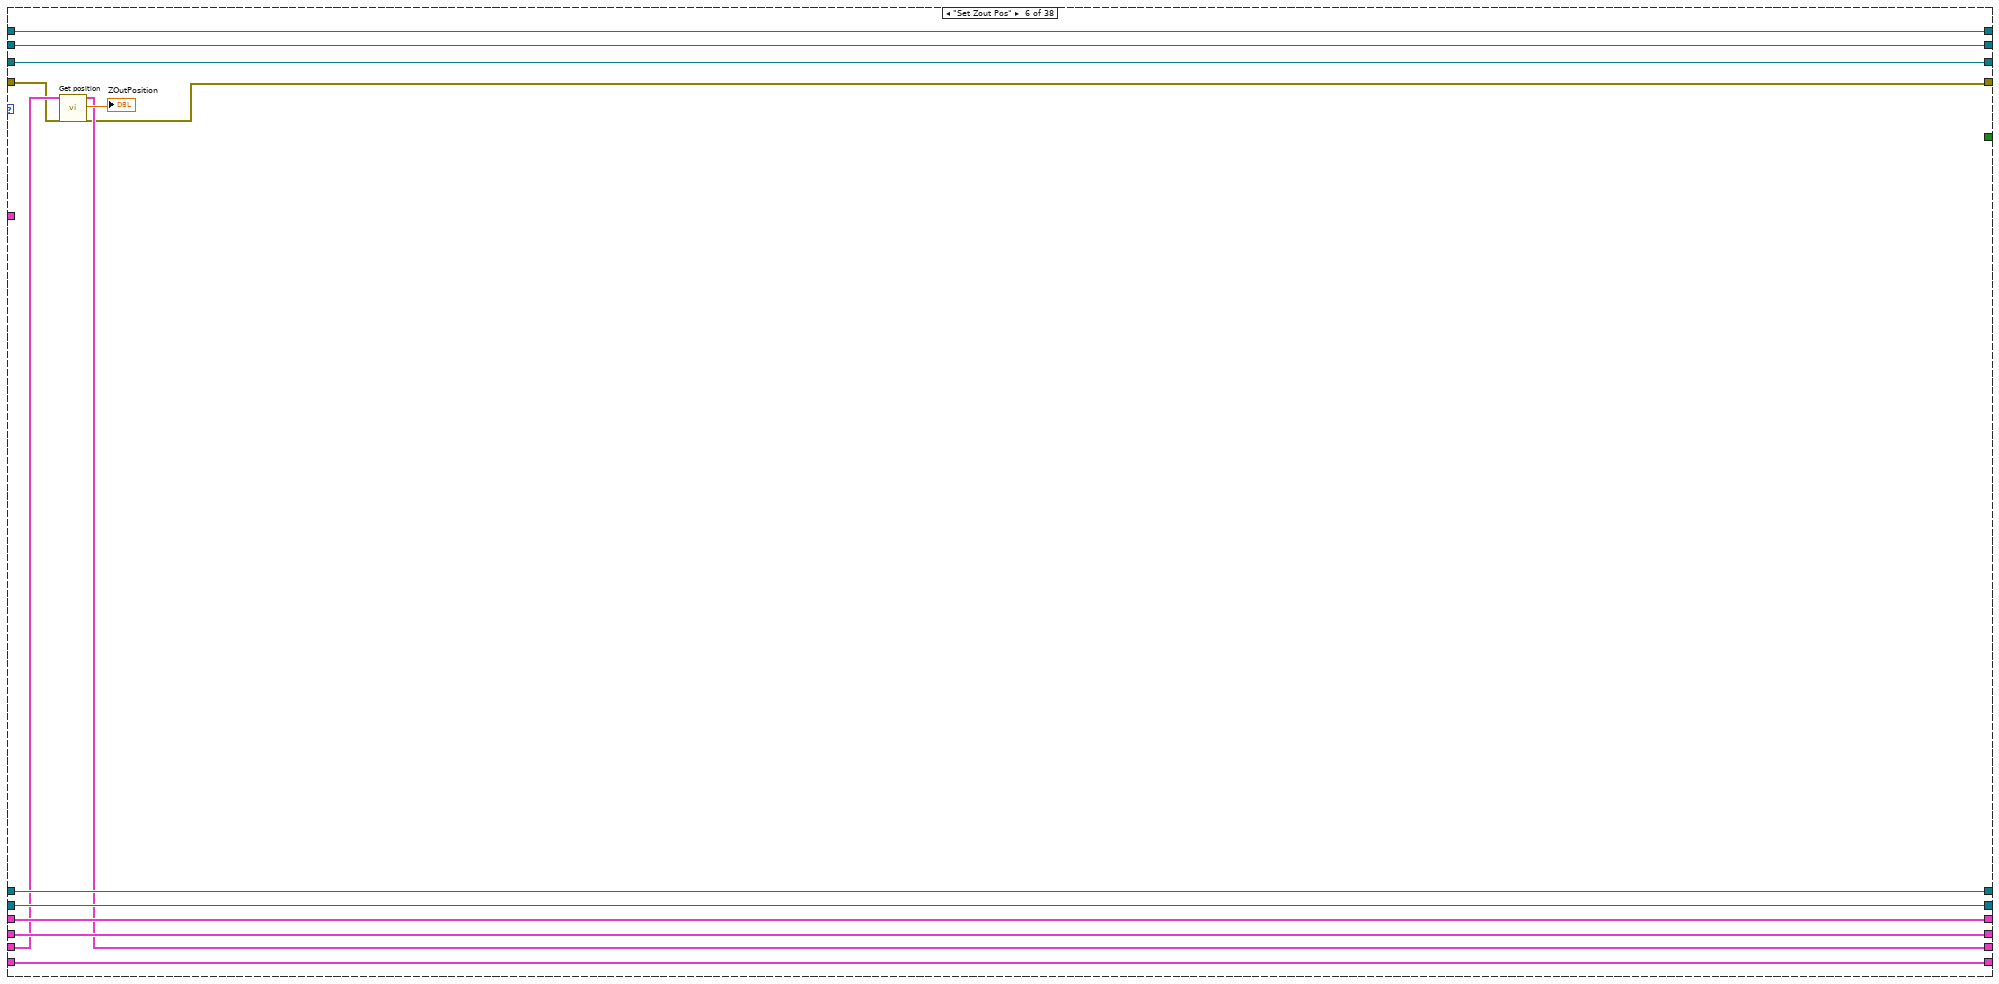
[diagram p17: hidden frame]
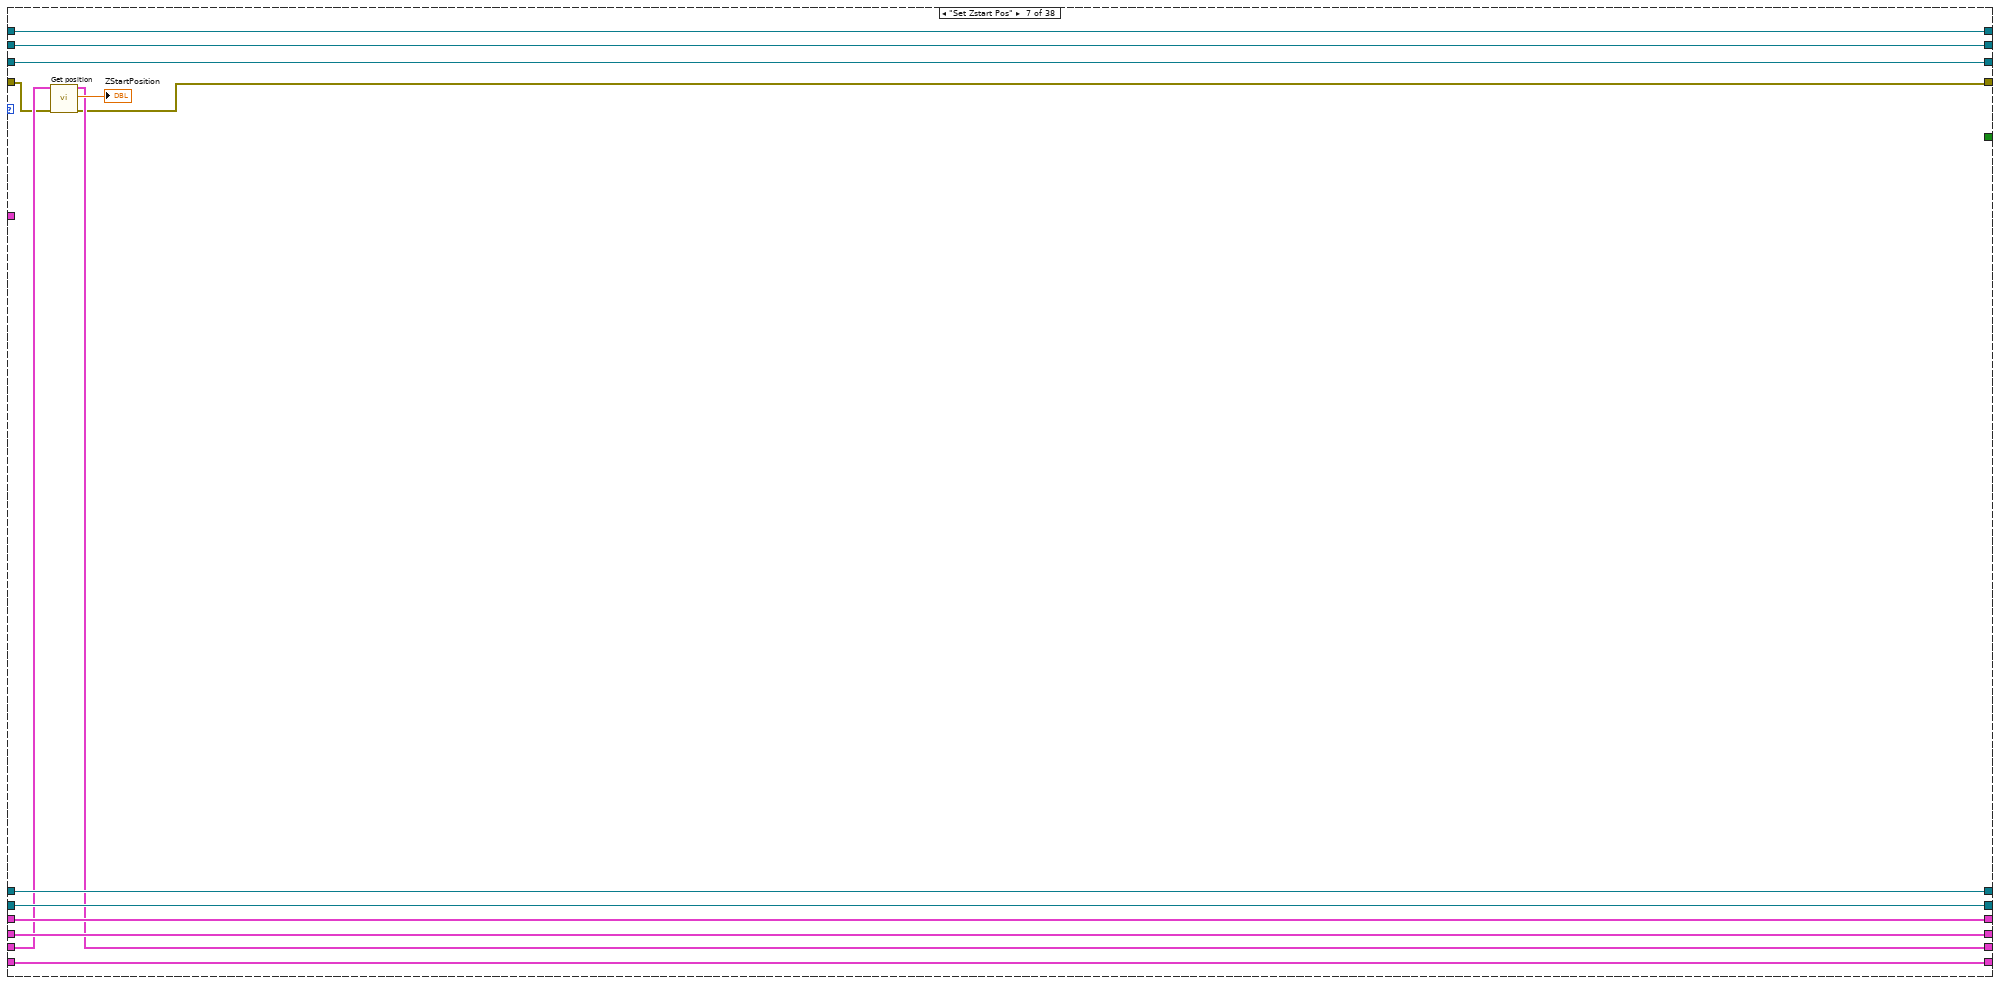
[diagram p18: hidden frame]
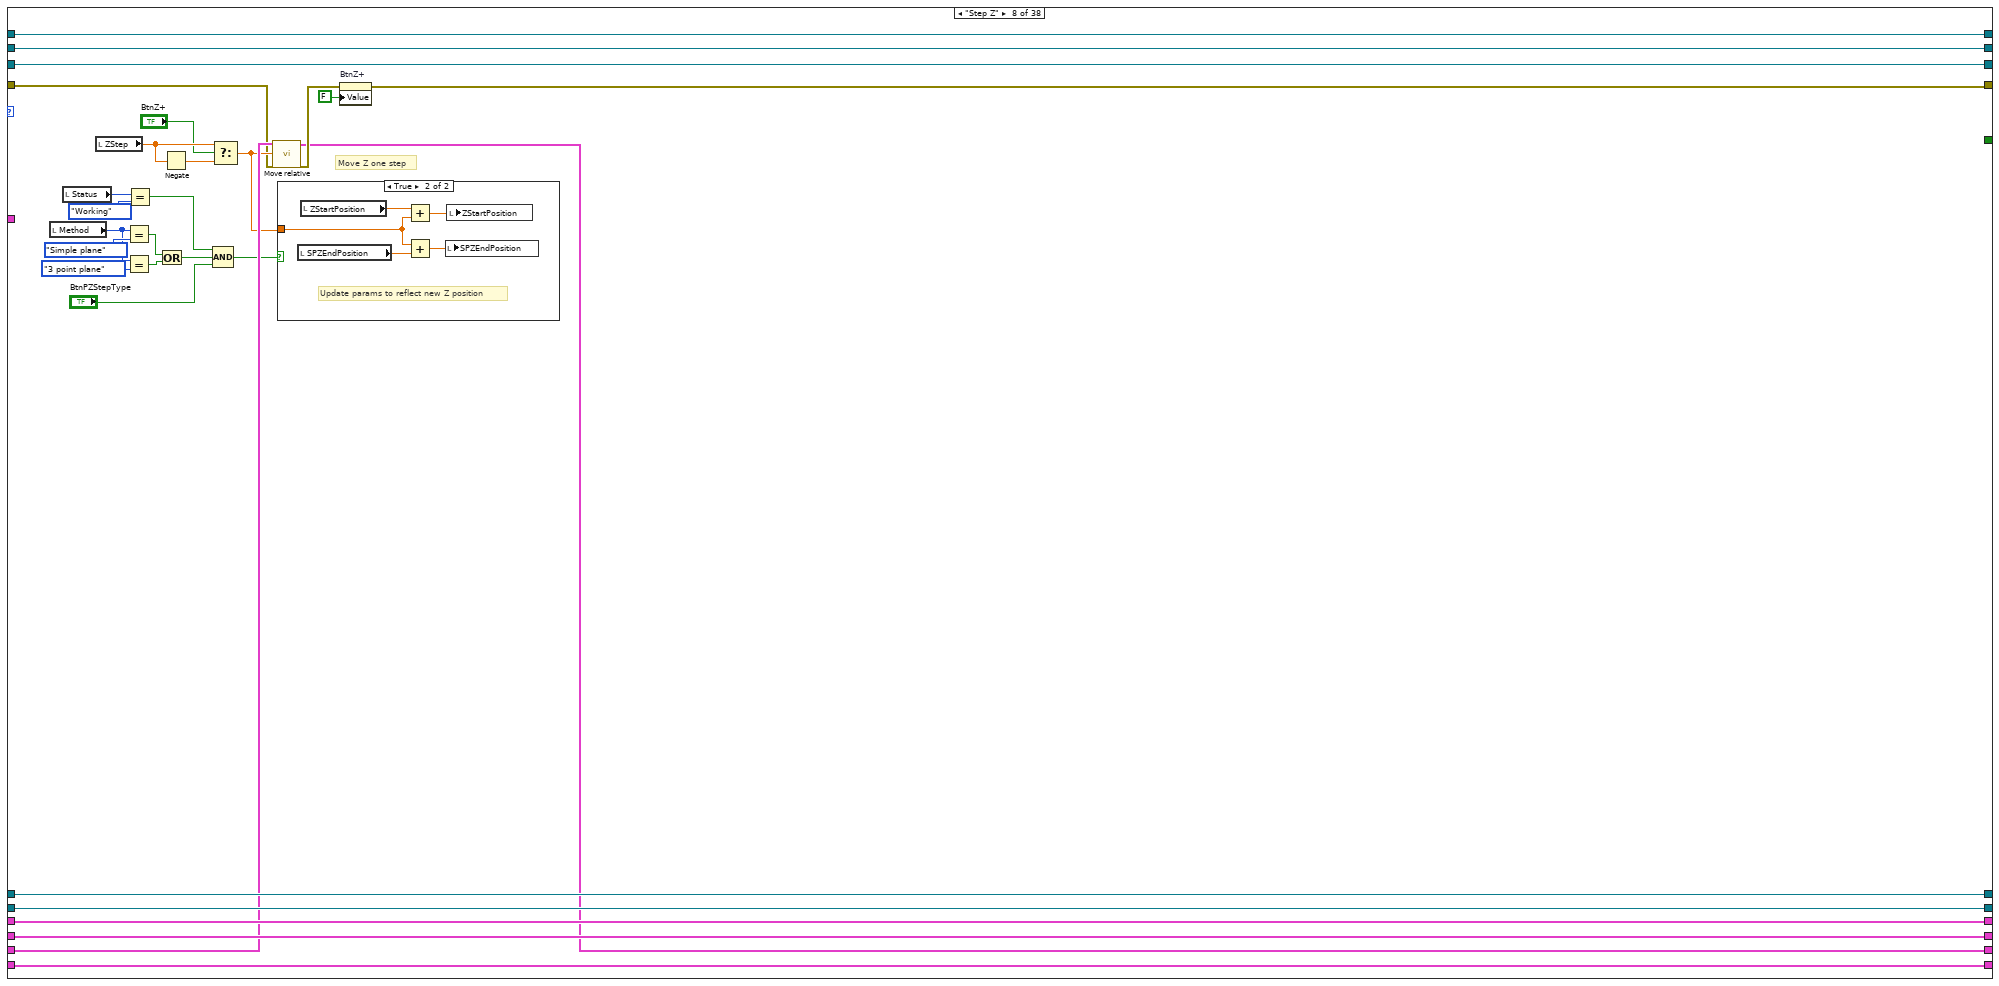
[diagram p19: hidden frame]
diagram:
  w13 = FALSE  # Quit
  w17 = T12 {"Placeholder"=FALSE}  # Program Info
  w23 = TRUE  # Done Event
  # "Initialize user events"
  # "User Interface Loop - Reads user input and places appropriate actions in the queue.\n\nAll user input is handled by the \"Event\" case thereby removing the need for polling.  \nNew events are placed at the end of the queue as to not interrupt any other \nongoing process.  The only exception to this practice would be placing an \nEmergency Stop procedure at the front of the  queue.\n\nNote -- Control values must be read before the event case can be reactivated."
  # "Done event stops user interface loop\nwhen instrument loop stops"
  # "Action\n???\n???\n???"
  # "Sequence of actions to perform \nwhen program starts\n\n0: SW Init\n1: HW Init - Zaber\n2: HW Init - DO\n3: Init Asynch Vis\n4: Set Motion Params\n5: Method UI and HW Init"
  n1 = Create User Event(user event datatype=w13) -> (user event=w7:refnum<user-event>, error out=w9:errorcluster)  [unwired: 1 in]
  n2 = Create User Event(user event datatype=w23, error in=w9) -> (user event=w22:refnum<user-event>, error out=w6:errorcluster)
  n3 = register-events(error in=w6, w22, w7) -> (reference out=w21:refnum<event-registration>, error out=w12:errorcluster)  [unwired: 1 in]
  n4 = Obtain Queue(element data type=T13 {"Action"=enum."Get Time", "1"=FALSE, "2"=FALSE, "3"=FALSE} ("Exec State"), error in (no error)=w12) -> (queue out=w26:refnum<queue>, error out=w25:errorcluster)  [unwired: 3 in, 1 out]
  n5 = for {
    tunnel: w26 -> [w31]
    tunnel: [w28] -> w18
    tunnel: T13[] [{"Action"=enum."SW Init", "1"=FALSE, "2"=FALSE, "3"=FALSE}, {"Action"=enum."HW Init - Zaber", "1"=FALSE, "2"=FALSE, "3"=FALSE}, {"Action"=enum."HW Init - DO", "1"=FALSE, "2"=FALSE, "3"=FALSE}, {"Action"=enum."Init Asynch Vis", "1"=FALSE, "2"=FALSE, "3"=FALSE}, {"Action"=enum."Set Motion Params", "1"=FALSE, "2"=FALSE, "3"=FALSE}, {"Action"=enum."Method UI and HW init", "1"=FALSE, "2"=FALSE, "3"=FALSE}] -> [w27] mode=indexing
    shift-right: [w29] -> w4
    shift-left: w25 -> [w30]
    # "Add to end of queue"
    n6 = Enqueue Element(queue=w31, element=w27, error in (no error)=w30) -> (queue out=w28:refnum<queue>, error out=w29:errorcluster)  [unwired: 1 in, 1 out]
  }
  n7 = while {
    tunnel: w22 -> [w56]
    tunnel: [w55] -> w20
    tunnel: w18 -> [w54]
    shift-right: [w49] -> _
    shift-left: w17 -> [w50]
    tunnel: w7 -> [w47]
    tunnel: [w46] -> w10
    shift-right: [w45] -> _
    shift-left: _ -> [w40]
    shift-right: [w44] -> _
    shift-left: _ -> [w41]
    shift-right: [w43] -> _
    shift-left: _ -> [w42]
    shift-right: [w39] -> _
    shift-left: _ -> [w37]
    shift-right: [w38] -> _
    shift-left: _ -> [w36]
    shift-right: [w33] -> w3
    shift-left: w4 -> [w34]
    tunnel: [w32] -> w14
    stop <- w48 stop-if-true
    # "Bruker DO"
    # "MS Trigger"
    # "Quit event"
    # "Done event"
    # "Y Zaber"
    # "X Zaber"
    # "Z Zaber"
    # "System state"
    # "Instrument Loop -\nReads actions from the queue and executes them"
    # "Check forTimeout"
    # "Check for Errors"
    # "Read\nnext\nTask"
    n8 = Dequeue Element(queue=w54, timeout in ms (-1)=500, error in (no error)=w34) -> (queue out=w53:refnum<queue>, element=w51:T13, timed out?=w59:bool, error out=w35:errorcluster)
    n9 = Unbundle By Name(w51) -> ("Action"=w57:T14)
    n10 = Select(t=Actions."Get Time", s=w59, f=w57) -> (s? t:f=w60:T14)
    n11 = Select(t=Actions."Error", s=w35, f=w60) -> (s? t:f=w52:T14)
    n12 = case shown="\"Line Motion\"" w52 {
      tunnel: w56 -> [w109 w113 w165 w187 w258 w387 w391 w403 w448 w483 w495 w526 w599 w618 w637 w640 w694 w735 w836 w886 w996 w1089 w1242 w1258 w1715 w1759 w1805 w1850 w1854 w1968 w2056 w2136 w2149 w2173 w2209 w2233 w2245 w2271]
      tunnel: [w109 w113 w165 w187 w258 w387 w391 w403 w448 w483 w495 w526 w599 w618 w637 w640 w694 w735 w836 w886 w996 w1089 w1242 w1258 w1715 w1759 w1805 w1850 w1854 w1968 w2056 w2136 w2149 w2173 w2209 w2223 w2245 w2271] -> w55
      tunnel: w53 -> [w108 w160 w183 w227 w256 w385 w399 w428 w446 w481 w493 w524 w597 w616 w635 w655 w692 w697 w822 w872 w1006 w1097 w1240 w1256 w1707 w1757 w1795 w1848 w1865 w1966 w2069 w2144 w2159 w2171 w2178 w2232 w2238 w2278]
      tunnel: w51 -> [_ _ _ _ _ _ _ _ _ _ _ _ _ _ _ _ _ _ _ _ _ _ _ _ _ _ _ _ _ _ _ _ _ _ _ _ _ _]
      tunnel: w50 -> [w107 w161 w184 w228 w257 w386 w400 w429 w447 w482 w494 w525 w598 w617 w636 w656 w693 w734 w835 w885 w993 w1098 w1241 w1257 w1714 w1758 w1804 w1849 w1866 w1967 w2070 w2143 w2160 w2172 w2210 w2230 w2246 w2279]
      tunnel: [w107 w161 w184 w228 w257 w386 w400 w429 w447 w482 w494 w525 w598 w617 w636 w656 w693 w734 w835 w885 w993 w1098 w1241 w1257 w1714 w1758 w1804 w1849 w1866 w1967 w2070 w2143 w2160 w2172 w2210 w2230 w2246 w2279] -> w49
      tunnel: [w108 w160 w183 w227 w256 w385 w399 w428 w446 w481 w493 w524 w597 w616 w635 w655 w692 w697 w819 w876 w1006 w1097 w1240 w1256 w1705 w1757 w1794 w1848 w1865 w1966 w2069 w2144 w2159 w2171 w2176 w2232 w2244 w2278] -> w32
      tunnel: [_ _ _ _ _ _ _ _ _ _ _ _ _ _ _ _ _ _ _ _ _ _ _ _ _ _ _ _ _ _ _ _ _ _ _ w2231 _ _] -> w48
      tunnel: w47 -> [w75 w112 w164 w196 w255 w377 w390 w427 w437 w480 w492 w498 w591 w615 w621 w654 w691 w733 w834 w884 w1005 w1088 w1235 w1247 w1713 w1749 w1803 w1847 w1864 w1965 w2068 w2142 w2148 w2163 w2184 w2224 w2237 w2270]
      tunnel: [w75 w112 w164 w196 w255 w377 w390 w427 w437 w480 w492 w498 w591 w615 w621 w654 w691 w733 w834 w884 w1005 w1088 w1235 w1247 w1713 w1749 w1803 w1847 w1864 w1965 w2068 w2142 w2148 w2163 w2183 w2224 w2237 w2270] -> w46
      tunnel: [w78 w118 w182 w213 w254 w378 w392 w404 w445 w479 w491 w499 w592 w602 w622 w641 w690 w699 w818 w883 w1004 w1090 w1239 w1248 w1700 w1756 w1802 w1846 w1863 w1964 w2067 w2139 w2150 w2170 w2206 w2227 w2241 w2274] -> w43
      tunnel: [w78 w117 w181 w214 w244 w384 w398 w426 w444 w478 w490 w523 w596 w603 w623 w642 w689 w700 w833 w882 w997 w1096 w1238 w1250 w1712 w1755 w1801 w1845 w1862 w1963 w2066 w2140 w2150 w2169 w2207 w2228 w2242 w2275] -> w44
      tunnel: [w78 w116 w180 w215 w243 w383 w397 w425 w443 w477 w489 w522 w595 w604 w624 w643 w688 w701 w832 w881 w998 w1095 w1237 w1251 w1711 w1754 w1800 w1844 w1861 w1962 w2065 w2141 w2150 w2168 w2208 w2229 w2243 w2276] -> w45
      tunnel: w42 -> [_ _ w182 w213 w254 w380 w394 w419 w445 w479 w491 w499 w592 w610 w628 w647 w690 w702 w823 w883 w1004 w1092 w1239 w1249 w1701 w1756 w1802 w1846 w1863 w1964 w2067 w2139 w2154 w2170 w2206 w2227 w2241 w2274]
      tunnel: w41 -> [_ _ w181 w214 w246 w384 w398 w426 w444 w478 w490 w523 w596 w611 w629 w648 w689 w703 w833 w882 w999 w1096 w1238 w1253 w1712 w1755 w1801 w1845 w1862 w1963 w2066 w2140 w2156 w2169 w2207 w2228 w2242 w2275]
      tunnel: w40 -> [_ _ w180 w215 w245 w383 w397 w425 w443 w477 w489 w522 w595 w612 w630 w649 w688 w704 w832 w881 w1000 w1095 w1237 w1252 w1711 w1754 w1800 w1844 w1861 w1962 w2065 w2141 w2155 w2168 w2208 w2229 w2243 w2276]
      tunnel: [w77 w114 w167 w188 w253 w382 w396 w424 w442 w476 w488 w521 w594 w614 w634 w653 w687 w732 w831 w880 w1003 w1094 w1236 w1255 w1710 w1750 w1799 w1843 w1860 w1961 w2064 w2137 w2158 w2164 w2204 w2225 w2239 w2272] -> w39
      tunnel: [w77 w115 w166 w189 w252 w381 w395 w423 w441 w475 w487 w520 w593 w613 w633 w652 w686 w731 w830 w879 w1002 w1093 w1233 w1244 w1709 w1753 w1798 w1842 w1859 w1960 w2063 w2138 w2157 w2164 w2205 w2226 w2240 w2273] -> w38
      tunnel: w37 -> [_ w114 _ w188 w253 w382 w396 w424 w442 w476 w488 w521 w594 w614 w634 w653 w687 w732 w831 w880 w1003 w1094 w1236 w1255 w1710 w1751 w1799 w1843 w1860 w1961 w2064 w2137 w2158 w2165 w2204 w2225 w2239 w2272]
      tunnel: w36 -> [_ w115 _ w189 w252 w381 w395 w423 w441 w475 w487 w520 w593 w613 w633 w652 w686 w731 w830 w879 w1002 w1093 w1233 w1245 w1709 w1753 w1798 w1842 w1859 w1960 w2063 w2138 w2157 w2166 w2205 w2226 w2240 w2273]
      tunnel: w35 -> [w74 w110 w162 w186 w242 w376 w389 w402 w436 w461 w485 w497 w590 w601 w620 w639 w657 w696 w816 w878 w995 w1087 w1234 w1243 w1699 w1748 w1788 w1838 w1853 w1958 w2055 w2135 w2147 w2162 w2177 w2222 w2235 w2269]
      tunnel: [w74 w111 w163 w185 w241 w375 w388 w401 w435 w460 w484 w496 w590 w600 w619 w638 w657 w695 w815 w875 w994 w1086 w1234 w1246 w1703 w1747 w1787 w1838 w1852 w1955 w2054 w2135 w2146 w2161 w2174 w2221 w2236 w2269] -> w33
      frame "SW Init" {
        w63 = FALSE ("CC start")
        w77 = refnum<k21> refnum ("task out")
        w78 = T1 {"Serial port handle"="", "Axis"="", "Controller #"=0, "Min position"=0.0, "Max position"=0.0, "Min velocity"=0.0, "Max velocity"=0.0, "Firmware"="", "Device ID"=0, "Variable event"=refnum, "Variable ref"=refnum, "Resolution, usteps/step"=0, "Serial port semaphore"=refnum, "Joystick buttons"={"MinDir"=1, "MaxDir"=2, "MedSpeed"=5, "HighSpeed"=6}} ("Zaber out")
        w82 = FALSE ("BtnSetZStartPosition")
        w64 = FALSE ("BtnPlaneSetPoint1")
        w81 = T15."Enabled" ("Disabled")
        w97 = u32 6618880
        w96 = u32 16711680
        w102 = T15."Enabled" ("Disabled")
        # "segLine accum"
        # "step index as file index, start from 1"
        # "status indicators"
        # "initialization: 0, end: ?"
        # "DLADS controller and indicator"
        # "Control bottons \nBtnSave: to save a (line scan) profile with z positions\nBtnSaveScanConfig: to save current scan configuration"
        # "Initialize plots?"
        n13 = local read "ZStartPosition"() -> (w103:dbl)
        n14 = local read "YStartPosition"() -> (w105:dbl)
        n15 = property on="XStartPosition" class="DigNum (strict)"("DisabledEnum"=w102, "Value"=0.0 ("Value (Signaling)")) -> ()  [unwired: 2 in, 2 out]
        n16 = property on="XEndPosition" class="DigNum (strict)"("DisabledEnum"=w102) -> ()  [unwired: 2 in, 2 out]
        n17 = property on="Velocity" class="DigNum (strict)"("DisabledEnum"=w102, "Value"=1.0 ("Velocity")) -> ()  [unwired: 2 in, 2 out]
        n18 = property on="StripLines" class="DigNum (strict)"("DisabledEnum"=w102, "Value"=u32 2 ("StripLines")) -> ()  [unwired: 2 in, 2 out]
        n19 = property on="XStageType" class="Enum (strict)"("DisabledEnum"=w102) -> ()  [unwired: 2 in, 2 out]
        n20 = property on="YStartPosition" class="DigNum (strict)"("DisabledEnum"=w102, "Value"=w105) -> ()  [unwired: 2 in, 2 out]
        n21 = property on="YEndPosition" class="DigNum (strict)"("DisabledEnum"=w102) -> ()  [unwired: 2 in, 2 out]
        n22 = property on="XStageType" class="Enum (strict)"("Value"=enum16{"Main motion", "Strip motion"}."Main motion" ("XMotionType")) -> ()  [unwired: 2 in, 2 out]
        n23 = property on="Method" class="Enum (strict)"("DisabledEnum"=w102, "Value"=T9."Simple plane" ("Value (Signaling)")) -> ()  [unwired: 2 in, 2 out]
        n24 = property on="ZStartPosition" class="DigNum (strict)"("DisabledEnum"=w102, "Value"=w103) -> ()  [unwired: 2 in, 2 out]
        n25 = property on="SPZEndPosition" class="DigNum (strict)"("DisabledEnum"=w102, "Value"=5.0 ("SPZEndPosition")) -> ()  [unwired: 2 in, 2 out]
        n26 = property on="BtnSetZStartPosition" class="Bool (strict)"("DisabledEnum"=w102, "Value"=w82) -> ()  [unwired: 2 in, 2 out]
        n27 = property on="BtnSetZOutPosition" class="Bool (strict)"("DisabledEnum"=w102, "Value"=w82) -> ()  [unwired: 2 in, 2 out]
        n28 = property on="BtnMeasurement" class="Bool (strict)"() -> ("Colors [4]"=w92:cluster{u32, u32}[])  [unwired: 2 in, 2 out]
        n29 = call "Create.vi"("Plots"=3) -> ("Data"=w83:cluster{cluster{dbl, dbl}[]}[])  [unwired: 18 in]
        "ZPositionPlot" <- w83
        n30 = local write "BtnPlaneSetPoint1"(w64) -> ()
        n31 = local write "BtnPlaneSetPoint2"(w64) -> ()
        n32 = local write "BtnPlaneSetPoint3"(w64) -> ()
        n33 = local write "BtnMeasurement"(w64) -> ()
        n34 = local write "BtnMeasurementPause"(w64) -> ()
        n35 = local write "BtnSave"(w64) -> ()
        n36 = local write "BtnZ-"(w64) -> ()
        n37 = local write "BtnZ+"(w64) -> ()
        n38 = local write "BtnSaveScanConfig"(w64) -> ()
        n39 = local write "BtnSaveSegLineRecords"(w64) -> ()
        n40 = local write "BtnSaveZToFile"(TRUE ("BtnSaveZToFile")) -> ()
        n41 = local write "Status"(Status."Idle" ("Status")) -> ()
        n42 = local write "Command"(Command."None" ("Command")) -> ()
        n43 = Index Array(array=w92, index #1=0 ("index"), index #2=1 ("index")) -> (element #1=w100:cluster{u32, u32}, element #2=w93:cluster{u32, u32})
        n44 = local write "LineZData"(w83) -> ()
        n45 = local write "Profile array"(cluster{dbl[], dbl[]}[] [] ("Profile array")) -> ()
        n46 = Bundle(cluster=w93, w96, w96) -> (w95:cluster{u32, u32})
        n47 = Bundle(cluster=w100, w97, w97) -> (w99:cluster{u32, u32})
        n48 = Build Array(w99, w95) -> (w91:cluster{u32, u32}[])
        n49 = property on="BtnMeasurement" class="Bool (strict)"("DisabledEnum"=w81, "BoolText.Text"="Start measurement" ("Boolean Text.Text"), "Colors [4]"=w91) -> ()  [unwired: 2 in, 2 out]
        n50 = property on="BtnExit" class="Bool (strict)"("DisabledEnum"=w81, "Value"=FALSE ("BtnExit")) -> ()  [unwired: 2 in, 2 out]
        n51 = property on="MSDwellTimeInSec" class="DigNum (strict)"("DisabledEnum"=w81) -> ()  [unwired: 2 in, 2 out]
        n52 = property on="BtnMeasurementPause" class="Bool (strict)"("DisabledEnum"=T15."Disabled and Grayed Out" ("Disabled"), "BoolText.Text"="Suspend" ("Boolean Text.Text")) -> ()  [unwired: 2 in, 2 out]
        n53 = local write "CC start"(w63) -> ()
        n54 = local write "CC stop"(w63) -> ()
        n55 = local write "LineMotion"(w63) -> ()
        n56 = local write "MS dwell"(w63) -> ()
        "Latest step idx" <- 0
        "Iterate ?" <- FALSE ("Iterate ?")
        "Wait to iterate ?" <- FALSE ("Wait to iterate ?")
        "Current step idx" <- 0
        "segLines" <- dbl[][] [] ("array")
        "relative main start" <- 0.0 ("relative main start")
        "relative main end" <- 0.0 ("relative main end")
      }
      frame "HW Init - Zaber" {
        w127 = T22 {"MinDir"=1, "MaxDir"=2, "MedSpeed"=5, "HighSpeed"=6}  # Joystick buttons
        n57 = Bundle By Name(cluster=w127, "MinDir"=35 ("MinDire"), "MaxDir"=33, "MedSpeed"=5, "HighSpeed"=6) -> (w128:T22)
        n58 = Bundle By Name(cluster=w127, "MinDir"=36 ("MinDire"), "MaxDir"=34, "MedSpeed"=5, "HighSpeed"=6) -> (w129:T22)
        n59 = Bundle By Name(cluster=w127, "MinDir"=2 ("MinDire"), "MaxDir"=4, "MedSpeed"=5, "HighSpeed"=6) -> (w122:T22)
        n60 = call "Connect.vi"("Axis"="Z", "VISA resource name"="Z stage", "baud rate (9600)"=u32 115200, "Controller #"=u8 1, "Joystick buttons"=w122, "error in"=w110) -> ("Zaber"=w118:T1, "error out"=w119:errorcluster)  [unwired: 12 in]
        "Z Zaber" <- w118
        n61 = call "Connect.vi"("Axis"="X", "VISA resource name"="X&Y stages", "baud rate (9600)"="Baud rate (9600 or 115200)", "Controller #"=u8 1, "Joystick buttons"=w129, "error in"=w110) -> ("Zaber"=w143:T1, "error out"=w126:errorcluster)  [unwired: 12 in]
        n62 = call "Join.vi"("Axis"="Y", "Controller #"=u8 2, "Joystick buttons"=w128, "error in"=w126, "Primary Zaber"=w143) -> ("Zaber"=w142:T1, "error out"=w125:errorcluster)  [unwired: 13 in]
        n63 = call "Get limits.vi"("Zaber"=w143, "error in"=w126) -> ("MIN position, mm"=w155:dbl, "Zaber out"=w117:T1, "MAX position, mm"=w154:dbl, "MIN velociry, mm/s"=w153:dbl, "MAX velocity, mm/s"=w145:dbl, "error out"=w120:errorcluster)  [unwired: 11 in, 1 out]
        n64 = property on="XEndPosition" class="DigNum (strict)"("Maximum"=w154, "Minimum"=w155) -> ()  [unwired: 2 in, 2 out]
        n65 = property on="XStartPosition" class="DigNum (strict)"("Maximum"=w154, "Minimum"=w155) -> ()  [unwired: 2 in, 2 out]
        n66 = Divide(x=w145, y=2.0) -> (x/y=w144:dbl)
        n67 = call "Get limits.vi"("Zaber"=w142, "error in"=w125) -> ("MIN position, mm"=w157:dbl, "Zaber out"=w116:T1, "MAX position, mm"=w156:dbl, "error out"=w121:errorcluster)  [unwired: 11 in, 3 out]
        n68 = property on="Velocity" class="DigNum (strict)"("Maximum"=w144, "Minimum"=w153) -> ()  [unwired: 2 in, 2 out]
        n69 = Merge Errors(w121, w120, w119) -> (w111:errorcluster)
        n70 = property on="YStartPosition" class="DigNum (strict)"("Maximum"=w156, "Minimum"=w157) -> ()  [unwired: 2 in, 2 out]
        n71 = property on="YEndPosition" class="DigNum (strict)"("Maximum"=w156, "Minimum"=w157) -> ()  [unwired: 2 in, 2 out]
      }
      frame "HW Init - DO" {
        n72 = call-poly <vilib>:"DAQmx Create Virtual Channel.vi"("lines"=tag "Dev1/port0/line0", "error in"=w162) -> ("task out"=w179:refnum<k21>, "error out"=w176:errorcluster)  [unwired: 3 in, 9 out]
        n73 = call-poly <vilib>:"DAQmx Create Virtual Channel.vi"("lines"=tag "Dev1/port0/line2", "error in"=w162) -> ("task out"=w174:refnum<k21>, "error out"=w171:errorcluster)  [unwired: 3 in, 9 out]
        n74 = call-poly <vilib>:"DAQmx Write.vi"("task/channels in"=w174, "data"=TRUE, "timeout"=0.0, "error in"=w171) -> ("task out"=w167:refnum<k21>, "error out"=w168:errorcluster)  [unwired: 1 in, 9 out]
        n75 = call-poly <vilib>:"DAQmx Write.vi"("task/channels in"=w179, "data"=TRUE, "timeout"=0.0, "error in"=w176) -> ("task out"=w166:refnum<k21>, "error out"=w169:errorcluster)  [unwired: 1 in, 9 out]
        n76 = Merge Errors(w169, w168) -> (w163:errorcluster)
      }
      frame "Init Asynch Vis" {
        # "Initialize joystick. Initialize and call Run.vi. Open vi front panel as hidden"
        # "open front panel as\nactive window"
        # "initialize and call Dialog3Stages.vi"
        n77 = call <vilib>:"Initialize Joystick.vi"("error in (no error)"=w186) -> ("error out"=w200:errorcluster, "device ID"=w198:refnum<k1>)  [unwired: 9 in]
        n78 = vi-ref "Run.vi"() -> (w202:refnum<vi>)
        n79 = case shown="\"Static\", Default" "Call type" {
          tunnel: [w229 w231] -> w192
          tunnel: w186 -> [w229 w230]
          frame "Static", Default {
          }
          frame "Dynamic" {
            w233 = TRUE  # Stop tune
            # "Create vi reference for Tip Tune ZaberAndSR865.vi"
            n80 = Create User Event(user event datatype=w233, error in=w230) -> (user event=→"Stop tune ShFrc":refnum<user-event>, error out=w240:errorcluster)
            n81 = vi-ref "Tip tune ZaberAndSR865.vi"() -> (w238:refnum<vi>)
            n82 = property class="VI"(reference=w238, error in=w240) -> (error out=w239:errorcluster, "Path"=w237:path)  [unwired: 1 out]
            n83 = Open VI Reference(type specifier VI Refnum (for type only)=refnum<vi> refnum, vi path=w237, options=256, error in (no error)=w239) -> (vi reference=→"Tune ShFrc":refnum<vi>, error out=w231:errorcluster)  [unwired: 2 in]
          }
        }
        n84 = property class="VI"(reference=w202, error in=w200) -> (error out=w199:errorcluster, "Path"=w201:path)  [unwired: 1 out]
        n85 = call "CreateJoystickEvent.vi"("error in"=w199) -> ("Joystick event"=w197:T23, "error out"=w206:errorcluster)  [unwired: 17 in]
        n86 = Open VI Reference(type specifier VI Refnum (for type only)=refnum<vi> refnum, vi path=w201, options=256, error in (no error)=w199) -> (vi reference=w210:refnum<vi>, error out=w205:errorcluster)  [unwired: 2 in]
        n87 = Merge Errors(w205, w206) -> (w204:errorcluster)
        n88 = call-by-ref "Start Asynchronous Call"(reference=w210, error in=w204, "Joystick ID"=w198, "Joystick event"=w197, "Stop event"=w196, "error in"=w204) -> (reference out=w208:refnum<vi>, error out=w207:errorcluster)  [unwired: 14 in, 2 out]
        n89 = invoke class="VI Interface Type 0" method="FP.Open"(reference=w208, error in=w207, "Activate"=TRUE ("Activate?"), "State"=T16."Hidden") -> (reference out=→"RunRef":refnum<vi>, error out=w193:errorcluster)  [unwired: 1 in, 3 out]
        n90 = vi-ref "Dialog3Stages.vi"() -> (w216:refnum<vi>)
        n91 = property class="VI"(reference=w216, error in=w186) -> (error out=w226:errorcluster, "Name"=w218:string)  [unwired: 1 out]
        n92 = Open VI Reference(type specifier VI Refnum (for type only)=refnum<vi> refnum, vi path=w218, options=256, error in (no error)=w226) -> (vi reference=w219:refnum<vi>, error out=w221:errorcluster)  [unwired: 2 in]
        n93 = call-by-ref "Start Asynchronous Call"(reference=w219, error in=w221, "X axis"=w214, "Y axis"=w215, "Z axis"=w213, "Stop event"=w196, "Joystick event"=w197, "error in"=w221) -> (reference out=w222:refnum<vi>, error out=w223:errorcluster)  [unwired: 13 in, 1 out]
        n94 = invoke class="VI Interface Type 1" method="FP.Open"(reference=w222, error in=w223, "Activate"=TRUE ("Activate?"), "State"=T16."Standard") -> (reference out=→"Dialog3StagesRef":refnum<vi>, error out=w194:errorcluster)  [unwired: 1 in, 3 out]
        n95 = Merge Errors(w194, w193, w192) -> (w185:errorcluster)
      }
      frame "Set Motion Params" {
        n96 = case shown="\"Idle\"" "Status" {
          tunnel: "XEndPosition" -> [_ w264]
          tunnel: "XStartPosition" -> [_ w265]
          tunnel: "YEndPosition" -> [_ w262]
          tunnel: "YStartPosition" -> [_ w263]
          tunnel: w246 -> [w259 w293]
          tunnel: w245 -> [w260 w292]
          tunnel: w242 -> [w261 w283]
          tunnel: [w261 w271] -> w241
          tunnel: [w259 w268] -> w244
          tunnel: [w260 w267] -> w243
          frame "Working", Default {
          }
          frame "Idle" {
            # "Update a bunch of stage motion parameters"
            n97 = case shown="\"3 point plane\"" "Method" {
              tunnel: [w341 w349 0.0] -> w309
              tunnel: "XStageType" -> [_ w347 _]
              tunnel: w264 -> [_ w346 _]
              tunnel: w265 -> [_ w345 _]
              tunnel: w262 -> [_ w344 _]
              tunnel: w263 -> [_ w343 _]
              frame "Simple plane" {
                n98 = local read "ZStartPosition"() -> (w342:dbl)
                n99 = Subtract(x="SPZEndPosition", y=w342) -> (x-y=w341:dbl)
              }
              frame "3 point plane" {
                n100 = Equal?(x=w347, y=enum16{"Main motion", "Strip motion"}."Main motion") -> (x = y?=w351:bool)
                n101 = case shown="False" w351 {
                  tunnel: [w355 w360] -> w349
                  tunnel: w346 -> [w354 _]
                  tunnel: w345 -> [w353 _]
                  tunnel: w344 -> [_ w358]
                  tunnel: w343 -> [_ w359]
                  frame True {
                    n102 = local read "PlaneZx"() -> (w356:dbl)
                    n103 = Subtract(x=w354, y=w353) -> (x-y=w357:dbl)
                    n104 = Multiply(x=w357, y=w356) -> (x*y=w355:dbl)
                  }
                  frame False {
                    n105 = local read "PlaneZy"() -> (w361:dbl)
                    n106 = Subtract(x=w358, y=w359) -> (x-y=w362:dbl)
                    n107 = Multiply(x=w362, y=w361) -> (x*y=w360:dbl)
                  }
                }
                n108 = local read "ZStartPosition"() -> (w350:dbl)
                n109 = Add(x=w350, y=w349) -> (x+y=w348:dbl)
                n110 = local write "SPZEndPosition"(w348) -> ()
              }
              frame Default {
              }
            }
            n111 = Decrement(x="StripLines") -> (x-1=w296:u32)
            n112 = Subtract(x=w262, y=w263) -> (x-y=w298:dbl)
            n113 = Subtract(x=w264, y=w265) -> (x-y=w297:dbl)
            n114 = case shown="\"Strip motion\"" "XStageType" {
              tunnel: [enum16{"Main motion", "Strip motion"}."Strip motion" ("Value (Signaling)") enum16{"Main motion", "Strip motion"}."Main motion" ("Value (Signaling)")] -> w294
              tunnel: w297 -> [w320 w331]
              tunnel: w298 -> [w317 w332]
              tunnel: [w320 w332] -> w281
              tunnel: w296 -> [w319 w333]
              tunnel: w263 -> [w318 _]
              tunnel: w265 -> [_ w330]
              tunnel: [w316 w329] -> w299
              tunnel: w293 -> [w315 w327]
              tunnel: w292 -> [w314 w328]
              tunnel: [w315 w328] -> w282
              tunnel: [w314 w327] -> w266
              frame "Main motion", Default {
                n115 = case shown="1, Default" w319 {
                  selector: w319 -> [_ w325]
                  tunnel: w318 -> [w322 _]
                  tunnel: w317 -> [_ w326]
                  tunnel: [0.0 w324] -> w316
                  frame 0 {
                    n116 = local write "YEndPosition"(w322) -> ()
                  }
                  frame 1, Default {
                    n117 = Divide(x=w326, y=w325) -> (x/y=w324:dbl)
                  }
                }
              }
              frame "Strip motion" {
                n118 = case shown="0" w333 {
                  selector: w333 -> [_ w338]
                  tunnel: w331 -> [_ w339]
                  tunnel: [0.0 w337] -> w329
                  tunnel: w330 -> [w335 _]
                  frame 0 {
                    n119 = local write "XEndPosition"(w335) -> ()
                  }
                  frame 1, Default {
                    n120 = Divide(x=w339, y=w338) -> (x/y=w337:dbl)
                  }
                }
              }
            }
            "YStageType" <- w294
            "StripStepRb" <- w299
            n121 = call "Get velocity.vi"("Zaber"=w282, "error in"=w283) -> ("Zaber out"=w291:T1, "Velocity, mm/s"=w284:dbl, "error out"=w290:errorcluster)  [unwired: 14 in, 1 out]
            n122 = call "Set velocity.vi"("Zaber in"=w291, "Velocity, mm/s"="Velocity", "error in"=w290) -> ("Zaber out"=w288:T1, "Velocity, mm/s"=w277:dbl, "error out"=w287:errorcluster)  [unwired: 14 in]
            n123 = local write "Velocity"(w277) -> ()
            n124 = Absolute Value(x=w281) -> (abs(x)=w280:dbl)
            n125 = call "Get motion time.vi"("Zaber"=w288, "Distance, mm"=w281, "error in"=w287) -> ("Zaber out"=w286:T1, "Motion time, s"=w274:dbl, "error out"=w285:errorcluster)  [unwired: 14 in]
            "LineTimeInSec" <- w274
            n126 = Divide(x=w280, y=w277) -> (x/y=w279:dbl)
            "LineStraightTime" <- w279
            n127 = call "Set velocity.vi"("Zaber in"=w286, "Velocity, mm/s"=w284, "error in"=w285) -> ("Zaber out"=w270:T1, "error out"=w271:errorcluster)  [unwired: 14 in, 1 out]
            n128 = Subtract(x=w274, y=w279) -> (x-y=w278:dbl)
            "LineTimeError" <- w278
            n129 = Divide(x=w274, y=60.0) -> (x/y=→"LineTimeInMin":dbl)
            n130 = case shown="\"Strip motion\"" "XStageType" {
              tunnel: w270 -> [w311 w313]
              tunnel: [w310 w313] -> w268
              tunnel: [w311 w312] -> w267
              tunnel: w266 -> [w310 w312]
              frame "Strip motion" {
              }
              frame "Main motion", Default {
              }
            }
            n131 = Divide(x=w309, y="ZStep") -> (x/y=w308:dbl)
            n132 = Round To Nearest(number=w308) -> (nearest integer value=w307:dbl)
            n133 = To Long Integer(number=w307) -> (32bit integer=w306:i32)
            n134 = case shown="Default" w306 {
              selector: w306 -> [_ w368]
              tunnel: [0.0 w374] -> w300
              tunnel: [0.0 w373] -> w302
              tunnel: [u32 0 w367] -> w301
              tunnel: w309 -> [_ w370]
              frame 0 {
              }
              frame Default {
                n135 = local read "LineTimeInMin"() -> (w369:dbl)
                n136 = Absolute Value(x=w368) -> (abs(x)=w367:i32)
                n137 = Multiply(x=w369, y=60.0) -> (x*y=w371:dbl)
                n138 = Divide(x=w370, y=w367) -> (x/y=w374:dbl)
                n139 = Divide(x=w371, y=w367) -> (x/y=w373:dbl)
              }
            }
            "PZStepTimeRb" <- w302
            "PZJumps" <- w301
            "PZRealStep" <- w300
            n140 = Compound Arithmetic op=MULTIPLY(w278, w277, 1000.0 ("value")) -> (→"LineError":dbl)
            "PZJump" <- u32 0 ("ZUpRb")
          }
        }
      }
      frame "Set Zout Pos" {
        n141 = call "Get position.vi"("Zaber"=w380, "error in"=w376) -> ("Zaber out"=w378:T1, "PositionRb"=→"ZOutPosition":dbl, "error out"=w375:errorcluster)  [unwired: 13 in, 2 out]
      }
      frame "Set Zstart Pos" {
        n142 = call "Get position.vi"("Zaber"=w394, "error in"=w389) -> ("Zaber out"=w392:T1, "PositionRb"=→"ZStartPosition":dbl, "error out"=w388:errorcluster)  [unwired: 13 in, 2 out]
      }
      frame "Step Z" {
        # "Move Z one step"
        n143 = local read "Method"() -> (w415:T9)
        n144 = local read "Status"() -> (w418:T11)
        n145 = local read "ZStep"() -> (w421:dbl)
        n146 = Equal?(x=w415, y=T9."Simple plane") -> (x = y?=w413:bool)
        n147 = Equal?(x=w415, y=T9."3 point plane") -> (x = y?=w412:bool)
        n148 = Equal?(x=w418, y=Status."Working") -> (x = y?=w411:bool)
        n149 = Or(x=w413, y=w412) -> (x .or. y?=w410:bool)
        n150 = Negate(x=w421) -> (-x=w422:dbl)
        n151 = Select(t=w421, s="BtnZ+", f=w422) -> (s? t:f=w407:dbl)
        n152 = Compound Arithmetic op=AND(w411, w410, "BtnPZStepType") -> (w408:bool)
        n153 = call "Move relative.vi"("Zaber"=w419, "Distance, mm"=w407, "error in"=w402) -> ("Zaber out"=w404:T1, "error out"=w406:errorcluster)  [unwired: 13 in, 2 out]
        n154 = case shown="True" w408 {
          tunnel: w407 -> [_ w433]
          frame False {
          }
          frame True {
            # "Update params to reflect new Z position"
            n155 = local read "SPZEndPosition"() -> (w432:dbl)
            n156 = local read "ZStartPosition"() -> (w434:dbl)
            n157 = Add(x=w434, y=w433) -> (x+y=w431:dbl)
            n158 = Add(x=w433, y=w432) -> (x+y=w430:dbl)
            n159 = local write "SPZEndPosition"(w430) -> ()
            n160 = local write "ZStartPosition"(w431) -> ()
          }
        }
        n161 = property on="BtnZ+" class="Bool (strict)"(error in=w406, "Value"=FALSE ("BtnZ+")) -> (error out=w401:errorcluster)  [unwired: 1 in, 1 out]
      }
      frame "Method close - Shear force" {
        # "Close SW and HW associated wth shear force method"
        n162 = local read "Call type"() -> (w440:enum16{"Dynamic", "Static"})
        n163 = case shown="\"Dynamic\"" w440 {
          tunnel: w436 -> [w449 w457]
          tunnel: [w449 w450] -> w438
          frame "Static", Default {
          }
          frame "Dynamic" {
            n164 = local read "Stop tune ShFrc"() -> (w459:refnum<user-event>)
            n165 = Generate User Event(user event=w459, event data cluster=TRUE ("event data"), error in=w457) -> (error out=w456:errorcluster)  [unwired: 1 in, 1 out]
            n166 = local read "Tune ShFrc"() -> (w455:refnum<vi>)
            n167 = call-by-ref "Wait On Asynchronous Call"(reference=w455, error in=w456) -> (reference out=w453:refnum<vi>, error out=w452:errorcluster, 19:"error out"=w451:errorcluster)  [unwired: 19 in]
            n168 = Merge Errors(w452, w451) -> (w454:errorcluster)
            n169 = invoke class="VI Interface Type 2" method="FP.Close"(reference=w453, error in=w454) -> (error out=w450:errorcluster)  [unwired: 1 in, 2 out]
          }
        }
        n170 = local read "SR865"() -> (w439:T6)
        n171 = call "Uninit.vi"("SR865 in"=w439, "error in"=w438) -> ("error out"=w435:errorcluster)  [unwired: 17 in]
      }
      frame "Method close - SICM" {
        # "Close SW and HW associated with SICM method"
        n172 = local read "Stop tune SICM"() -> (w465:refnum<user-event>)
        n173 = Generate User Event(user event=w465, event data cluster=TRUE ("event data"), error in=w461) -> (error out=w471:errorcluster)  [unwired: 1 in, 1 out]
        n174 = local read "SICM tip"() -> (w464:refnum<vi>)
        n175 = call-by-ref "Wait On Asynchronous Call"(reference=w464, error in=w471) -> (reference out=w469:refnum<vi>, error out=w473:errorcluster, 19:"error out"=w472:errorcluster)  [unwired: 19 in]
        n176 = Merge Errors(w473, w472) -> (w466:errorcluster)
        n177 = invoke class="VI Interface Type 3" method="FP.Close"(reference=w469, error in=w466) -> (reference out=w467:refnum<vi>, error out=w468:errorcluster)  [unwired: 1 in, 1 out]
        n178 = Close Reference(reference=w467, error in (no error)=w468) -> (error out=w470:errorcluster)
        n179 = Destroy User Event(user event=w465, error in=w470) -> (error out=w463:errorcluster)
        n180 = local read "RBD9103"() -> (w462:T5)
        n181 = call "DisconnectR.vi"("RBD9103"=w462, "error in"=w463) -> ("error out"=w460:errorcluster)  [unwired: 17 in]
      }
      frame "Method close - Keyence" {
        # "Close Keyence HW"
        n182 = local read "Keyence"() -> (w486:T4)
        n183 = call "DisconnectK.vi"("Keyence"=w486, "error in"=w485) -> ("error out"=w484:errorcluster)  [unwired: 17 in]
      }
      frame "Method UI and HW init" {
        # "Init hardware and software associated with new method type"
        # "Update UI tab visibility"
        n184 = property on="TabPlanes" class="TabCtl (strict)"(error in=w497) -> (error out=w517:errorcluster, "Pages"=w516:refnum<vi>[])  [unwired: 1 in, 1 out]
        n185 = local read "Method"() -> (w501:T9)
        n186 = property on="TabMethods" class="TabCtl (strict)"(error in=w497) -> (error out=w519:errorcluster, "Pages"=w518:refnum<vi>[])  [unwired: 1 in, 1 out]
        n187 = To Long Integer(number=w501) -> (32bit integer=w513:i32)
        n188 = Index Array(array=w516, index #1=0 ("index"), index #2=1 ("index")) -> (element #1=w509:refnum<vi>, element #2=w508:refnum<vi>)
        n189 = Decrement(x=w513) -> (x-1=w514:i32)
        n190 = Greater Or Equal To 0?(x=w514) -> (x >= 0?=w515:bool)
        n191 = case shown="Default" w501 {
          tunnel: w509 -> [_ w571 w583]
          tunnel: w508 -> [_ w570 w581]
          tunnel: w517 -> [w569 w574 w579]
          tunnel: [w569 w572 w578] -> w507
          frame Default {
          }
          frame "Simple plane" {
            n192 = property class="Page"(reference=w571, error in=w574, "PageVis"=TRUE ("Page Visible")) -> (error out=w576:errorcluster)  [unwired: 1 out]
            n193 = property class="Page"(reference=w570, error in=w576, "PageVis"=FALSE ("Page Visible")) -> (error out=w572:errorcluster)  [unwired: 1 out]
          }
          frame "3 point plane" {
            n194 = property class="Page"(reference=w581, error in=w579, "PageVis"=TRUE ("Page Visible")) -> (error out=w582:errorcluster)  [unwired: 1 out]
            n195 = property class="Page"(reference=w583, error in=w582, "PageVis"=FALSE ("Page Visible")) -> (error out=w578:errorcluster)  [unwired: 1 out]
          }
        }
        n196 = Select(t=w514, s=w515, f=0) -> (s? t:f=w512:i32)
        n197 = Index Array(array=w518, index=w512) -> (element=w511:refnum<vi>)
        n198 = property class="Page"(reference=w511, error in=w519, "PageVis"=TRUE ("Page Visible")) -> (error out=w510:errorcluster)  [unwired: 1 out]
        n199 = for {
          tunnel: w518 -> [w589] mode=indexing
          shift-right: [w587] -> w506
          shift-left: w510 -> [w588]
          tunnel: w512 -> [w586]
          i -> [w585]
          n200 = Equal?(x=w586, y=w585) -> (x = y?=w584:bool)
          n201 = property class="Page"(reference=w589, error in=w588, "PageVis"=w584) -> (error out=w587:errorcluster)  [unwired: 1 out]
        }
        n202 = Merge Errors(w506, w507) -> (w500:errorcluster)
        n203 = case shown="\"Shear force sensor\"" w501 {
          tunnel: w500 -> [w543 w545 w546 w555]
          tunnel: w499 -> [w534 _ _ w552]
          tunnel: [w529 w545 w547 w551] -> w496
          frame "SICM sensor" {
            w542 = TRUE  # Stop tune
            n204 = call "ConnectR.vi"("VISA resource name"="RBD9103 COM", "error in"=w543) -> ("RBD9103"=w533:T5, "error out"=w541:errorcluster)  [unwired: 16 in]
            "RBD9103" <- w533
            n205 = Create User Event(user event datatype=w542, error in=w541) -> (user event=w532:refnum<user-event>, error out=w540:errorcluster)
            "Stop tune SICM" <- w532
            n206 = Open VI Reference(type specifier VI Refnum (for type only)=refnum<vi> refnum, vi path=".\\SICM tip\\Tune SICM method_2.vi", options=256, error in (no error)=w540) -> (vi reference=w535:refnum<vi>, error out=w536:errorcluster)  [unwired: 2 in]
            "SICM tip" <- w535
            n207 = call-by-ref "Start Asynchronous Call"(reference=w535, error in=w536, "Z axis"=w534, "RBD9103"=w533, "Stop event"=w532, "error in"=w536) -> (reference out=w531:refnum<vi>, error out=w530:errorcluster)  [unwired: 15 in, 1 out]
            n208 = invoke class="VI Interface Type 3" method="FP.Open"(reference=w531, error in=w530, "Activate"=TRUE ("Activate?"), "State"=T16."Standard") -> (error out=w529:errorcluster)  [unwired: 1 in, 4 out]
          }
          frame Default {
          }
          frame "Keyence sensor" {
            n209 = call "ConnectK.vi"("VISA resource name"="Keyence COM port", "Baud rate"=u32 115200, "error in"=w546) -> ("Keyence"=→"Keyence":T4, "error out"=w547:errorcluster)  [unwired: 15 in]
          }
          frame "Shear force sensor" {
            n210 = local read "Call type"() -> (w557:enum16{"Dynamic", "Static"})
            n211 = call "Init.vi"("VISA resource name"="SR865", "error in"=w555) -> ("SR865"=w553:T6, "error out"=w554:errorcluster)  [unwired: 16 in]
            "SR865" <- w553
            n212 = case shown="\"Static\", Default" w557 {
              tunnel: w554 -> [w558 w568]
              tunnel: w553 -> [_ w566]
              tunnel: w552 -> [_ w565]
              tunnel: [w558 w560] -> w551
              frame "Static", Default {
              }
              frame "Dynamic" {
                n213 = local read "Tune ShFrc"() -> (w567:refnum<vi>)
                n214 = local read "Stop tune ShFrc"() -> (w564:refnum<user-event>)
                n215 = call-by-ref "Start Asynchronous Call"(reference=w567, error in=w568, "Z axis"=w565, "SR865"=w566, "Stop event"=w564, "error in"=w568) -> (reference out=w563:refnum<vi>, error out=w562:errorcluster)  [unwired: 15 in, 1 out]
                n216 = invoke class="VI Interface Type 2" method="FP.Open"(reference=w563, error in=w562, "Activate"=TRUE ("Activate?"), "State"=T16."Standard") -> (error out=w560:errorcluster)  [unwired: 1 in, 4 out]
              }
            }
          }
        }
      }
      frame "Tune Shear Force" {
      }
      frame "Plane Set Point 1" {
        n217 = call "Get position.vi"("Zaber"=w612, "error in"=w601) -> ("Zaber out"=w604:T1, "PositionRb"=→"PlaneY1":dbl, "error out"=w609:errorcluster)  [unwired: 13 in, 2 out]
        n218 = call "Get position.vi"("Zaber"=w611, "error in"=w609) -> ("Zaber out"=w603:T1, "PositionRb"=→"PlaneX1":dbl, "error out"=w608:errorcluster)  [unwired: 13 in, 2 out]
        n219 = call "Get position.vi"("Zaber"=w610, "error in"=w608) -> ("Zaber out"=w602:T1, "PositionRb"=→"PlaneZ1":dbl, "error out"=w600:errorcluster)  [unwired: 13 in, 2 out]
      }
      frame "Plane Set Point 2" {
        n220 = call "Get position.vi"("Zaber"=w630, "error in"=w620) -> ("Zaber out"=w624:T1, "PositionRb"=→"PlaneY2":dbl, "error out"=w632:errorcluster)  [unwired: 13 in, 2 out]
        n221 = call "Get position.vi"("Zaber"=w629, "error in"=w632) -> ("Zaber out"=w623:T1, "PositionRb"=→"PlaneX2":dbl, "error out"=w631:errorcluster)  [unwired: 13 in, 2 out]
        n222 = call "Get position.vi"("Zaber"=w628, "error in"=w631) -> ("Zaber out"=w622:T1, "PositionRb"=→"PlaneZ2":dbl, "error out"=w619:errorcluster)  [unwired: 13 in, 2 out]
      }
      frame "Plane Set Point 3" {
        n223 = call "Get position.vi"("Zaber"=w649, "error in"=w639) -> ("Zaber out"=w643:T1, "PositionRb"=→"PlaneY3":dbl, "error out"=w651:errorcluster)  [unwired: 13 in, 2 out]
        n224 = call "Get position.vi"("Zaber"=w648, "error in"=w651) -> ("Zaber out"=w642:T1, "PositionRb"=→"PlaneX3":dbl, "error out"=w650:errorcluster)  [unwired: 13 in, 2 out]
        n225 = call "Get position.vi"("Zaber"=w647, "error in"=w650) -> ("Zaber out"=w641:T1, "PositionRb"=→"PlaneZ3":dbl, "error out"=w638:errorcluster)  [unwired: 13 in, 2 out]
      }
      frame "Calculate Plane" {
        # "Calculate imaging plane"
        n226 = local read "PlaneX2"() -> (w671:dbl)
        n227 = local read "PlaneX1"() -> (w670:dbl)
        n228 = local read "PlaneX3"() -> (w669:dbl)
        n229 = local read "PlaneX1"() -> (w668:dbl)
        n230 = local read "PlaneY2"() -> (w667:dbl)
        n231 = local read "PlaneY1"() -> (w666:dbl)
        n232 = local read "PlaneY3"() -> (w665:dbl)
        n233 = local read "PlaneY1"() -> (w664:dbl)
        n234 = local read "PlaneZ2"() -> (w663:dbl)
        n235 = local read "PlaneZ1"() -> (w662:dbl)
        n236 = local read "PlaneZ3"() -> (w661:dbl)
        n237 = local read "PlaneZ1"() -> (w660:dbl)
        n238 = Subtract(x=w661, y=w660) -> (x-y=w684:dbl)
        n239 = Subtract(x=w671, y=w670) -> (x-y=w681:dbl)
        n240 = Subtract(x=w663, y=w662) -> (x-y=w685:dbl)
        n241 = Subtract(x=w669, y=w668) -> (x-y=w672:dbl)
        n242 = Subtract(x=w667, y=w666) -> (x-y=w673:dbl)
        n243 = Subtract(x=w665, y=w664) -> (x-y=w680:dbl)
        n244 = Build Array(w685, w684) -> (w683:dbl[])
        n245 = Build Array(w681, w673) -> (w679:dbl[])
        n246 = Build Array(w672, w680) -> (w678:dbl[])
        n247 = Build Array(w679, w678) -> (w677:dbl[][])
        n248 = call-poly <vilib>:"Solve Linear Equations.vi"("matrix type"=Matrix_Type_of_Inverse_Matrix."General", "Known Vector"=w683, "Input Matrix"=w677) -> ("Solution Vector"=w676:dbl[])  [unwired: 1 out]
        n249 = Index Array(array=w676, index #1=0 ("index"), index #2=1 ("index")) -> (element #1=→"PlaneZx":dbl, element #2=→"PlaneZy":dbl)
      }
      frame "Scan UI" {
        # "Update UI based on scan status"
        n250 = property on="BtnMeasurement" class="Bool (strict)"() -> ("Colors [4]"=w706:cluster{u32, u32}[])  [unwired: 2 in, 2 out]
        n251 = case shown="\"Start\"" "Command" {
          tunnel: [T15."Disabled and Grayed Out" ("Disabled") w772 w796 w800 w809] -> w721
          tunnel: w696 -> [w745 w759 w782 w805 w814]
          tunnel: [w745 w756 w779 w805 w814] -> w720
          tunnel: [w744 w772 w796 w800 w808] -> w711
          tunnel: [w744 w772 T15."Disabled and Grayed Out" ("Disabled") w800 w808] -> w710
          tunnel: ["Stop measurement" ("Caption.Text") "Stopping measurement" ("Boolean Text.Text") "Start measurement" ("Caption.Text") "Stop measurement" ("Caption.Text") "Stop measurement" ("Caption.Text")] -> w709
          tunnel: ["Suspend" ("Caption.Text") "Suspend" ("Caption.Text") "Suspend" ("Caption.Text") "Suspending" ("Caption.Text") "Suspend" ("Caption.Text")] -> w708
          tunnel: [T15."Disabled and Grayed Out" ("Disabled") T15."Enabled" ("Disabled") w796 w800 w809] -> w707
          tunnel: w706 -> [w740 w763 w785 w804 w813]
          tunnel: [w740 w760 w783 w804 w813] -> w705
          tunnel: w704 -> [w739 w755 w778 w803 w812]
          tunnel: w703 -> [w738 w754 w776 w802 w811]
          tunnel: w702 -> [w737 w753 w774 w801 w810]
          tunnel: [w739 w752 w777 w803 w812] -> w701
          tunnel: [w738 w751 w775 w802 w811] -> w700
          tunnel: [w737 w750 w773 w801 w810] -> w699
          frame "Start" {
            w744 = T15."Enabled" ("Disabled")
            w748 = u32 0 ("StripLineRb")
            # "Start imaging"
            n252 = local write "PZJump"(w748) -> ()
            "Profile array" <- cluster{dbl[], dbl[]}[] []
            "StripLineRb" <- w748
            "LineNumber" <- u32 0 ("StripLines")
          }
          frame "Stop" {
            w770 = u32 16711916
            w766 = u32 16711916
            w772 = T15."Disabled and Grayed Out" ("Disabled")
            # "Stop imaging"
            n253 = call "Stop move.vi"("Zaber"=w755, "error in"=w759) -> ("Zaber out"=w752:T1, "error out"=w758:errorcluster)  [unwired: 16 in]
            n254 = call "Stop move.vi"("Zaber"=w754, "error in"=w758) -> ("Zaber out"=w751:T1, "error out"=w757:errorcluster)  [unwired: 16 in]
            n255 = call "Stop move.vi"("Zaber"=w753, "error in"=w757) -> ("Zaber out"=w750:T1, "error out"=w756:errorcluster)  [unwired: 16 in]
            n256 = Index Array(array=w763, index #1=0 ("index"), index #2=1 ("index")) -> (element #1=w767:cluster{u32, u32}, element #2=w764:cluster{u32, u32})
            n257 = Bundle(cluster=w764, w766, w766) -> (w771:cluster{u32, u32})
            n258 = Bundle(cluster=w767, w770, w770) -> (w768:cluster{u32, u32})
            n259 = Build Array(w768, w771) -> (w760:cluster{u32, u32}[])
          }
          frame "Finish", Default {
            w789 = u32 6618880
            w784 = u32 16711680
            w796 = T15."Enabled" ("Disabled")
            # "Imaging finished"
            n260 = call "Stop move.vi"("Zaber"=w778, "error in"=w782) -> ("Zaber out"=w777:T1, "error out"=w781:errorcluster)  [unwired: 16 in]
            n261 = call "Stop move.vi"("Zaber"=w776, "error in"=w781) -> ("Zaber out"=w775:T1, "error out"=w780:errorcluster)  [unwired: 16 in]
            n262 = call "Stop move.vi"("Zaber"=w774, "error in"=w780) -> ("Zaber out"=w773:T1, "error out"=w779:errorcluster)  [unwired: 16 in]
            n263 = Index Array(array=w785, index #1=0 ("index"), index #2=1 ("index")) -> (element #1=w792:cluster{u32, u32}, element #2=w786:cluster{u32, u32})
            n264 = Bundle(cluster=w786, w784, w784) -> (w788:cluster{u32, u32})
            n265 = local write "BtnMeasurement"(FALSE ("BtnMeasurement")) -> ()
            n266 = Bundle(cluster=w792, w789, w789) -> (w791:cluster{u32, u32})
            n267 = Build Array(w791, w788) -> (w783:cluster{u32, u32}[])
          }
          frame "Suspend" {
            w800 = T15."Disabled and Grayed Out" ("Disabled")
            # "Suspend imaging"
          }
          frame "Resume" {
            w808 = T15."Enabled" ("Disabled")
            w809 = T15."Disabled and Grayed Out" ("Disabled")
            # "Resume imaging"
          }
        }
        n268 = property on="XStageType" class="Enum (strict)"(error in=w720, "DisabledEnum"=w721) -> (error out=w730:errorcluster)  [unwired: 1 in, 1 out]
        n269 = property on="Velocity" class="DigNum (strict)"(error in=w720, "DisabledEnum"=w721) -> (error out=w726:errorcluster)  [unwired: 1 in, 1 out]
        n270 = property on="BtnMeasurement" class="Bool (strict)"(error in=w720, "Colors [4]"=w705, "DisabledEnum"=w711, "BoolText.Text"=w709) -> (error out=w719:errorcluster)  [unwired: 1 in, 1 out]
        n271 = property on="Method" class="Enum (strict)"(error in=w720, "DisabledEnum"=w721) -> (error out=w723:errorcluster)  [unwired: 1 in, 1 out]
        n272 = property on="XStartPosition" class="DigNum (strict)"(error in=w730, "DisabledEnum"=w721) -> (error out=w729:errorcluster)  [unwired: 1 in, 1 out]
        n273 = property on="StripLines" class="DigNum (strict)"(error in=w726, "DisabledEnum"=w721) -> (error out=w725:errorcluster)  [unwired: 1 in, 1 out]
        n274 = property on="SPZEndPosition" class="DigNum (strict)"(error in=w723, "DisabledEnum"=w721) -> (error out=w722:errorcluster)  [unwired: 1 in, 1 out]
        n275 = property on="BtnMeasurementPause" class="Bool (strict)"(error in=w719, "DisabledEnum"=w710, "BoolText.Text"=w708) -> (error out=w718:errorcluster)  [unwired: 1 in, 1 out]
        n276 = property on="BtnSetZOutPosition" class="Bool (strict)"(error in=w725, "DisabledEnum"=w721) -> (error out=w724:errorcluster)  [unwired: 1 in, 1 out]
        n277 = property on="XEndPosition" class="DigNum (strict)"(error in=w729, "DisabledEnum"=w721) -> (error out=w728:errorcluster)  [unwired: 1 in, 1 out]
        n278 = property on="MSDwellTimeInSec" class="DigNum (strict)"(error in=w722, "DisabledEnum"=w721) -> (error out=w715:errorcluster)  [unwired: 1 in, 1 out]
        n279 = property on="YStartPosition" class="DigNum (strict)"(error in=w728, "DisabledEnum"=w721) -> (error out=w727:errorcluster)  [unwired: 1 in, 1 out]
        n280 = property on="BtnExit" class="Bool (strict)"(error in=w718, "DisabledEnum"=w707) -> (error out=w714:errorcluster)  [unwired: 1 in, 1 out]
        n281 = property on="BtnSetZStartPosition" class="Bool (strict)"(error in=w724, "DisabledEnum"=w721) -> (error out=w716:errorcluster)  [unwired: 1 in, 1 out]
        n282 = property on="YEndPosition" class="DigNum (strict)"(error in=w727, "DisabledEnum"=w721) -> (error out=w717:errorcluster)  [unwired: 1 in, 1 out]
        n283 = Merge Errors(w717, w716, w715, w714) -> (w713:errorcluster)
        n284 = property on="Command" class="Enum (strict)"(error in=w713, "Value"=Command."None" ("Command")) -> (error out=w695:errorcluster)  [unwired: 1 in, 1 out]
      }
      frame "Scan Ctrl" {
        # "determine :  ideal\n                     or \n                      working     determine:  normal mode\n                                                              or \n                                                              DLADS mode"
        n285 = local read "Command"() -> (w824:T10)
        n286 = local read "Status"() -> (w817:T11)
        n287 = Not Equal?(x=w824, y=Command."Finish") -> (x != y?=w829:bool)
        n288 = Equal?(x=Status."Working" ("y"), y=w817) -> (x = y?=w828:bool)
        n289 = And(x=w829, y=w828) -> (x .and. y?=w825:bool)
        n290 = case shown="True" w825 {
          tunnel: w823 -> [w837 w847]
          tunnel: w816 -> [w839 w846]
          tunnel: [w839 w840] -> w821
          tunnel: [T13[] [{"Action"=enum."Wait (ms)", "1"=FALSE, "2"=FALSE, "3"=FALSE}] w845] -> w820
          tunnel: [w837 w844] -> w818
          tunnel: w817 -> [_ w843]
          frame False {
            # "0: Wait"
          }
          frame True {
            w850 = 1000.0 ("y")
            # "Calculate dt and t0 for simple\nplane and 3 point plane methods"
            n291 = case shown="\"Working\", \"Pause\"" w843 {
              tunnel: w847 -> [w866 w870]
              tunnel: [w866 w869] -> w851
              tunnel: w846 -> [w865 w868]
              tunnel: [w865 w867] -> w852
              frame "Idle", Default {
              }
              frame "Working", "Pause" {
                n292 = local read "ZOutPosition"() -> (w871:dbl)
                n293 = call "Move absolute.vi"("Zaber"=w870, "Position, mm"=w871, "error in"=w868) -> ("Zaber out"=w869:T1, "error out"=w867:errorcluster)  [unwired: 13 in, 2 out]
              }
            }
            n294 = local read "PZRealStep"() -> (w853:dbl)
            n295 = call "Get motion time.vi"("Zaber"=w851, "Distance, mm"=w853, "error in"=w852) -> ("Zaber out"=w844:T1, "Motion time, s"=w859:dbl, "error out"=w841:errorcluster)  [unwired: 14 in]
            n296 = local read "PZStepTimeRb"() -> (w858:dbl)
            n297 = Multiply(x=w858, y=w850) -> (x*y=w857:dbl)
            "dt" <- w857
            n298 = Multiply(x=w850, y=w859) -> (x*y=w856:dbl)
            n299 = Subtract(x=w857, y=w856) -> (x-y=w855:dbl)
            n300 = Divide(x=w855, y=2.0) -> (x/y=w854:dbl)
            n301 = Absolute Value(x=w854) -> (abs(x)=→"t0":dbl)
            n302 = case shown="True" "BtnDLADS" {
              tunnel: [T13[] [{"Action"=enum."XY and Sensor Init", "1"=FALSE, "2"=FALSE, "3"=FALSE}, {"Action"=enum."Z Init", "1"=FALSE, "2"=FALSE, "3"=FALSE}, {"Action"=enum."MS Trig", "1"=FALSE, "2"=FALSE, "3"=FALSE}, {"Action"=enum."Line Motion", "1"=FALSE, "2"=FALSE, "3"=FALSE}, {"Action"=enum."MS Complete", "1"=FALSE, "2"=FALSE, "3"=FALSE}, {"Action"=enum."Z Exit Ctrl", "1"=FALSE, "2"=FALSE, "3"=FALSE}, {"Action"=enum."Pause Check Ctrl", "1"=FALSE, "2"=FALSE, "3"=FALSE}] T13[] [{"Action"=enum."Handle DLADS", "1"=FALSE, "2"=FALSE, "3"=FALSE}]] -> w845
              tunnel: [w861 w863] -> w840
              tunnel: w841 -> [w861 w863]
              frame False {
                # "0: XY and Sensor Init\n1: Z Init\n2: MS Trig\n3: Line Motion\n4: MS Complete\n5: Z Exit Ctrl\n6: Pause Check Ctrl"
              }
              frame True {
                # "0: Handle DLADS"
              }
            }
            "SFMAirError" <- FALSE ("SFMAirError")
          }
        }
        n303 = call "Add to Queue.vi"("error in (no error)"=w821, "Actions"=w820, "Queue Ref In"=w822) -> ("error out"=w815:errorcluster, "Queue Ref Out"=w819:refnum<queue>)  [unwired: 7 in]
      }
      frame "Handle DLADS" {
        n304 = flat-sequence {
          tunnel: w878 -> [w888]
          tunnel: [w887] -> w877
          tunnel: w877 -> [w974]
          tunnel: [w973] -> w874
          tunnel: [w972] -> w873
          frame #0 {
            n305 = while {
              tunnel: w888 -> [w898]
              tunnel: [w896] -> w887
              stop <- w891 stop-if-true
              # "If error, all values will be 0.\nLets try to avoid errors and avoid line scan."
              # "When to break the polling loop?\n1, iterate with UNLOOK\n2. stop measurement"
              n306 = String To Path(string="sample DLADS prediction") -> (path=w902:path)
              n307 = Wait (ms)(milliseconds to wait=u32 500) -> ()  [unwired: 1 out]
              n308 = Build Path(base path=w902, name or relative path=path "UNLOCK" ("default name")) -> (appended path=w901:path)
              n309 = Read from Text File(file (use dialog)=w901, error in=w898) -> (text=w897:string, error out=w889:errorcluster)  [unwired: 1 in, 3 out]
              n310 = case shown="No Error" w889 {
                tunnel: w897 -> [w957 _]
                frame No Error {
                  # "move before the location for pre-scan"
                  # "unit for positions: mm"
                  # "for v0.8.6 UNLOCK format"
                  # "update the motion positions"
                  # "read 1st and last item for segline mode"
                  n311 = Spreadsheet String To Array(format string="%f", spreadsheet string=w957, array type (2D Dbl)=string[][] [] ("Array")) -> (array=w924:string[][])  [unwired: 1 in]
                  n312 = Array Size(array=w924) -> (size(s)=w955:i32[])
                  n313 = Index Array(array=w955, index=0) -> (element=w953:i32)
                  n314 = Subtract(x=w953, y=1) -> (x-y=w951:i32)
                  n315 = Index Array(array=w924, index (row) #1=0 ("disabled index (row)"), index (col) #1=0 ("disabled index (col)"), index (row) #2=w951, index (col) #2=0 ("disabled index (col)")) -> (element #1=w925:string, element #2=w947:string)
                  n316 = Search/Split String(string=w947, search string/char (-)=",", offset (0)=1) -> (match + rest of string=w945:string)  [unwired: 2 out]
                  n317 = Search/Split String(string=w925, search string/char (-)=",", offset (0)=1) -> (match + rest of string=w932:string)  [unwired: 2 out]
                  n318 = Search/Split String(string=w945, search string/char (-)=")") -> (substring before match=w942:string)  [unwired: 1 in, 2 out]
                  n319 = Search/Split String(string=w925, search string/char (-)=",") -> (substring before match=w937:string)  [unwired: 1 in, 2 out]
                  n320 = Search/Split String(string=w932, search string/char (-)=")") -> (substring before match=w929:string)  [unwired: 1 in, 2 out]
                  n321 = Replace Substring(2:2 ("length (len. of substring)"), 4:"" ("substring (\"\")"), 5:w942) -> (1:w939:string)  [unwired: 1 in, 1 out]
                  n322 = Replace Substring(2:2 ("length (len. of substring)"), 4:"" ("substring (\"\")"), 5:w929) -> (1:w926:string)  [unwired: 1 in, 1 out]
                  n323 = Replace Substring(2:1 ("length (len. of substring)"), 4:"" ("substring (\"\")"), 5:w937) -> (1:w934:string)  [unwired: 1 in, 1 out]
                  n324 = Decimal String To Number(string=w939) -> (number=w913:i32)  [unwired: 2 in, 1 out]
                  n325 = Decimal String To Number(string=w926) -> (number=w917:i32)  [unwired: 2 in, 1 out]
                  n326 = Decimal String To Number(string=w934) -> (number=w921:i32)  [unwired: 2 in, 1 out]
                  n327 = local read "XStageType"() -> (w911:enum16{"Main motion", "Strip motion"})
                  n328 = local read "StripStepRb"() -> (w923:dbl)
                  n329 = Decrement(x=w921) -> (x-1=w922:i32)
                  n330 = Divide(x=w913, y=1000) -> (x/y=w912:dbl)
                  n331 = Divide(x=w917, y=1000) -> (x/y=w915:dbl)
                  n332 = case shown="\"Main motion\"" w911 {
                    tunnel: [w962 w965] -> w910
                    tunnel: [w963 w964] -> w909
                    frame "Main motion" {
                      n333 = local read "YStartPosition"() -> (w963:dbl)
                      n334 = local read "XStartPosition"() -> (w962:dbl)
                    }
                    frame "Strip motion", Default {
                      n335 = local read "XStartPosition"() -> (w964:dbl)
                      n336 = local read "YStartPosition"() -> (w965:dbl)
                    }
                  }
                  n337 = Multiply(x=w923, y=w922) -> (x*y=w918:dbl)
                  n338 = local read "Latest step idx"() -> (w956:i32)
                  n339 = local write "Current step idx"(w921) -> ()
                  n340 = local read "Pre-scan time, s"() -> (w908:dbl)
                  n341 = local write "relative main end"(w912) -> ()
                  n342 = local write "relative main start"(w915) -> ()
                  n343 = local read "Velocity"() -> (w907:dbl)
                  n344 = Not Equal?(x=w956, y=w921) -> (x != y?=w959:bool)
                  n345 = Add(x=w915, y=w910) -> (x+y=w905:dbl)
                  n346 = Add(x=w910, y=w912) -> (x+y=→"Main motion \nend position":dbl)
                  n347 = Multiply(x=w908, y=w907) -> (x*y=w904:dbl)
                  n348 = Not(x=w959) -> (.not. x?=w958:bool)
                  n349 = Add(x=w918, y=w909) -> (x+y=→"Strip motion \nposition":dbl)
                  n350 = Subtract(x=w905, y=w904) -> (x-y=→"Main motion\nstart position":dbl)
                  n351 = local write "Iterate ?"(w959) -> ()
                  n352 = local write "Wait to iterate ?"(w958) -> ()
                }
                frame Error {
                  n353 = local write "Wait to iterate ?"(TRUE ("Wait to iterate ?")) -> ()
                  n354 = local write "Iterate ?"(FALSE ("Iterate ?")) -> ()
                }
              }
              n355 = call <vilib>:"Clear Errors.vi"("error in (no error)"=w889, "specific error code to clear (0: all)"=0) -> ("error out"=w896:errorcluster)  [unwired: 4 in, 1 out]
              n356 = local read "Status"() -> (w894:T11)
              n357 = local read "Iterate ?"() -> (w890:bool)
              n358 = Equal?(x=w894, y=Status."Stopping") -> (x = y?=w892:bool)
              n359 = Or(x=w892, y=w890) -> (x .or. y?=w891:bool)
            }
          }
          frame #1 {
            # "no finish condition yet..."
            # "update DLADS control, except 'Status' == 'Stopping'"
            n360 = local read "Status"() -> (w970:T11)
            n361 = Not Equal?(x=w970, y=Status."Stopping") -> (x != y?=w968:bool)
            n362 = case shown="True" w968 {
              frame False {
              }
              frame True {
                n363 = local write "Wait to iterate ?"(FALSE ("Wait to iterate ?")) -> ()
                n364 = local read "Current step idx"() -> (w981:i32)
                n365 = local write "Iterate ?"(FALSE ("Iterate ?")) -> ()
                n366 = local read "relative main start"() -> (w975:dbl)
                n367 = To Double Precision Float(number=w981) -> (double precision float=w980:dbl)
                n368 = local write "Latest step idx"(w981) -> ()
                n369 = local read "relative main end"() -> (w976:dbl)
                n370 = Initialize Array(w980, 1 ("dimension size")) -> (w983:dbl[])
                n371 = Insert Into Array(array=w983, new element=w975) -> (w982:dbl[])  [unwired: 1 in]
                n372 = local read "segLines"() -> (w979:dbl[][])
                n373 = Insert Into Array(array=w982, new element=w976) -> (w978:dbl[])  [unwired: 1 in]
                n374 = Insert Into Array(array=w979, new element=w978) -> (w977:dbl[][])  [unwired: 2 in]
                n375 = local write "segLines"(w977) -> ()
              }
            }
            n376 = case shown="True" TRUE {
              tunnel: w974 -> [w989 w992]
              tunnel: [w988 w992] -> w973
              tunnel: [T13[] [] T13[] [{"Action"=enum."XY and Sensor Init", "1"=FALSE, "2"=FALSE, "3"=FALSE}, {"Action"=enum."Z Init", "1"=FALSE, "2"=FALSE, "3"=FALSE}, {"Action"=enum."MS Trig", "1"=FALSE, "2"=FALSE, "3"=FALSE}, {"Action"=enum."Line Motion", "1"=FALSE, "2"=FALSE, "3"=FALSE}, {"Action"=enum."MS Complete", "1"=FALSE, "2"=FALSE, "3"=FALSE}, {"Action"=enum."Z Exit Ctrl", "1"=FALSE, "2"=FALSE, "3"=FALSE}, {"Action"=enum."Pause Check Ctrl", "1"=FALSE, "2"=FALSE, "3"=FALSE}]] -> w972
              frame False {
                n377 = property on="Command" class="Enum (strict)"(error in=w989, "Val(Sgnl)"=Command."Finish" ("Value (Signaling)")) -> (error out=w988:errorcluster)  [unwired: 1 in, 1 out]
              }
              frame True {
                # "0: XY and Sensor Init\n1: Z Init\n2: MS Trig\n3: Line Motion\n4: MS complete\n5: Z Exit Ctrl\n6: Pause Check Ctrl"
              }
            }
          }
        }
        n378 = call "Add to Queue.vi"("error in (no error)"=w874, "Actions"=w873, "Queue Ref In"=w872) -> ("error out"=w875:errorcluster, "Queue Ref Out"=w876:refnum<queue>)  [unwired: 7 in]
      }
      frame "XY and Sensor Init" {
        n379 = local read "Status"() -> (w1001:T11)
        n380 = case shown="\"Working\", \"Pause\"" w1001 {
          tunnel: w1000 -> [w1007 w1030]
          tunnel: w999 -> [w1008 w1039]
          tunnel: w995 -> [w1009 w1016]
          tunnel: [w1009 w1019] -> w994
          tunnel: [w1007 w1018] -> w998
          tunnel: [w1008 w1017] -> w997
          frame "Idle", Default {
          }
          frame "Working", "Pause" {
            # "x stage"
            # "y stage"
            # "provide strip step or strip position, TBD"
            # "Move XY to line start position"
            n381 = local read "XStartPosition"() -> (w1014:dbl)
            n382 = local read "YStartPosition"() -> (w1013:dbl)
            n383 = local read "Main motion\nstart position"() -> (w1011:dbl)
            n384 = local read "Strip motion \nposition"() -> (w1010:dbl)
            n385 = local read "LineNumber"() -> (w1024:u32)
            n386 = local read "StripStepRb"() -> (w1025:dbl)
            n387 = local read "Method"() -> (w1023:T9)
            n388 = Multiply(x=w1025, y=w1024) -> (x*y=w1012:dbl)
            n389 = local write "StripLineRb"(w1024) -> ()
            n390 = local read "BtnDLADS"() -> (w1015:bool)
            n391 = case shown="\"Shear force sensor\"" w1023 {
              tunnel: w1016 -> [w1063 w1073 w1085]
              tunnel: [w1063 w1064 w1077] -> w1022
              frame Default {
              }
              frame "Shear force sensor" {
                w1074 = T24 2 items=["X", "Y", "R", "Theta", "IN1", "IN2", "IN3", "IN4", "OUT1", "OUT2", "XNoise", "YNoise", "Phase", "SineOut", "DCLevel", "IntRefFreq", "ExtRefFreq"] ("DataChannel")
                n392 = local read "CurrentAirLevel"() -> (w1067:dbl)
                n393 = local read "SR865"() -> (w1075:T6)
                n394 = call "DataChannelRead.vi"("SR865 in"=w1075, "DataChannel"=w1074, "error in"=w1073) -> ("Signal"=w1068:dbl, "error out"=w1064:errorcluster)  [unwired: 14 in, 1 out]
                n395 = flat-sequence {
                  tunnel: w1068 -> [w1076]
                  tunnel: w1067 -> [_]
                  frame #0 {
                    "CurrentAirLevel" <- w1076
                  }
                }
                n396 = Subtract(x=w1068, y="SFMShiftFromAirLevel") -> (x-y=→"SFMWorkingLevel":dbl)
                n397 = Subtract(x=w1068, y=w1067) -> (x-y=w1069:dbl)
                n398 = Absolute Value(x=w1069) -> (abs(x)=w1070:dbl)
                n399 = Greater?(x=w1070, y="SFMAirErrorLevel") -> (0:w1065:bool)
                n400 = local write "SFMAirError"(w1065) -> ()
              }
              frame "SICM sensor" {
                n401 = local read "RBD9103"() -> (w1084:T5)
                n402 = call "Read.vi"("RBD9103"=w1084, "error in"=w1085) -> ("Value, nA"=w1078:dbl, "error out"=w1077:errorcluster)  [unwired: 12 in, 4 out]
                "SIMCurrentLevel" <- w1078
                n403 = Subtract(x="SIMAirLevelSp", y=w1078) -> (x-y=w1082:dbl)
                n404 = Absolute Value(x=w1082) -> (abs(x)=w1081:dbl)
                n405 = Greater?(x=w1081, y="SIMAirErrorLevel") -> (0:→"SIMAirError":bool)
              }
            }
            n406 = call "Get limits.vi"("Zaber"=w1030, "error in"=w1016) -> ("Zaber out"=w1036:T1, "MAX velocity, mm/s"=w1029:dbl, "error out"=w1034:errorcluster)  [unwired: 11 in, 4 out]
            n407 = call "Get limits.vi"("Zaber"=w1039, "error in"=w1016) -> ("Zaber out"=w1038:T1, "MAX velocity, mm/s"=w1028:dbl, "error out"=w1032:errorcluster)  [unwired: 11 in, 4 out]
            n408 = case shown="False" w1015 {
              tunnel: [w1044 w1055] -> w1027
              tunnel: [w1043 w1054] -> w1026
              tunnel: w1014 -> [w1042 _]
              tunnel: w1013 -> [w1041 _]
              tunnel: w1012 -> [w1040 _]
              tunnel: w1011 -> [_ w1057]
              tunnel: w1010 -> [_ w1056]
              frame False {
                n409 = local read "XStageType"() -> (w1045:enum16{"Main motion", "Strip motion"})
                n410 = case shown="\"Main motion\"" w1045 {
                  tunnel: [w1048 w1053] -> w1044
                  tunnel: [w1049 w1050] -> w1043
                  tunnel: w1042 -> [w1048 w1052]
                  tunnel: w1041 -> [w1047 w1050]
                  tunnel: w1040 -> [w1046 w1051]
                  frame "Main motion" {
                    n411 = Add(x=w1047, y=w1046) -> (x+y=w1049:dbl)
                  }
                  frame "Strip motion", Default {
                    n412 = Add(x=w1052, y=w1051) -> (x+y=w1053:dbl)
                  }
                }
              }
              frame True {
                n413 = local read "XStageType"() -> (w1058:enum16{"Main motion", "Strip motion"})
                n414 = case shown="\"Strip motion\", Default" w1058 {
                  tunnel: [w1060 w1061] -> w1055
                  tunnel: w1057 -> [w1060 w1062]
                  tunnel: w1056 -> [w1059 w1061]
                  tunnel: [w1059 w1062] -> w1054
                  frame "Main motion" {
                  }
                  frame "Strip motion", Default {
                  }
                }
              }
            }
            n415 = call "Set velocity.vi"("Zaber in"=w1036, "Velocity, mm/s"=w1029, "error in"=w1034) -> ("Zaber out"=w1035:T1, "error out"=w1033:errorcluster)  [unwired: 14 in, 1 out]
            n416 = call "Set velocity.vi"("Zaber in"=w1038, "Velocity, mm/s"=w1028, "error in"=w1032) -> ("Zaber out"=w1037:T1, "error out"=w1031:errorcluster)  [unwired: 14 in, 1 out]
            n417 = call "Move absolute.vi"("Zaber"=w1035, "Position, mm"=w1026, "error in"=w1033) -> ("Zaber out"=w1018:T1, "error out"=w1021:errorcluster)  [unwired: 13 in, 2 out]
            n418 = call "Move absolute.vi"("Zaber"=w1037, "Position, mm"=w1027, "error in"=w1031) -> ("Zaber out"=w1017:T1, "error out"=w1020:errorcluster)  [unwired: 13 in, 2 out]
            n419 = Merge Errors(w1022, w1021, w1020) -> (w1019:errorcluster)
          }
        }
        n420 = Unbundle By Name(w993) -> ()  [unwired: 3 out]
      }
      frame "Z Init" {
        n421 = local read "Status"() -> (w1091:T11)
        n422 = case shown="\"Working\", \"Pause\"" w1091 {
          selector: w1091 -> [_ w1103]
          tunnel: w1092 -> [w1099 w1107]
          tunnel: w1087 -> [w1100 w1106]
          tunnel: [w1100 w1105] -> w1086
          tunnel: [w1099 w1104] -> w1090
          frame "Idle", Default {
          }
          frame "Working", "Pause" {
            n423 = flat-sequence {
              tunnel: w1107 -> [w1117]
              tunnel: w1106 -> [w1116]
              tunnel: w1103 -> [w1108]
              tunnel: [w1111] -> w1102
              tunnel: [w1110] -> w1101
              tunnel: [w1231] -> w1104
              tunnel: [w1232] -> w1105
              tunnel: w1102 -> [w1232]
              tunnel: w1101 -> [w1231]
              frame #0 {
                # "Let's move Z to the 3-point plane to handel tilt, firstly."
                # "A new workflow to make 3-points a prerequisite"
                # "Let's land Z to the surface, secondly."
                # "Move Z to start pos"
                n424 = local read "ZStartPosition"() -> (w1119:dbl)
                n425 = local read "Method"() -> (w1113:T9)
                n426 = case shown="\"Shear force sensor\"" w1113 {
                  tunnel: w1119 -> [w1203 w1204 w1217]
                  tunnel: [w1203 w1205 w1216] -> w1118
                  frame Default {
                  }
                  frame "3 point plane" {
                    n427 = local read "XStageType"() -> (w1208:enum16{"Main motion", "Strip motion"})
                    n428 = local read "PlaneZy"() -> (w1209:dbl)
                    n429 = local read "StripLineRb"() -> (w1210:u32)
                    n430 = local read "PlaneZx"() -> (w1206:dbl)
                    n431 = local read "StripStepRb"() -> (w1211:dbl)
                    n432 = Equal?(x=w1208, y=enum16{"Main motion", "Strip motion"}."Main motion") -> (x = y?=w1215:bool)
                    n433 = Select(t=w1209, s=w1215, f=w1206) -> (s? t:f=w1214:dbl)
                    n434 = Multiply(x=w1211, y=w1210) -> (x*y=w1213:dbl)
                    n435 = Multiply(x=w1213, y=w1214) -> (x*y=w1212:dbl)
                    n436 = Add(x=w1212, y=w1204) -> (x+y=w1205:dbl)
                  }
                  frame "Shear force sensor" {
                    n437 = local read "XStageType"() -> (w1220:enum16{"Main motion", "Strip motion"})
                    n438 = local read "PlaneZy"() -> (w1221:dbl)
                    n439 = local read "StripLineRb"() -> (w1222:u32)
                    n440 = local read "PlaneZx"() -> (w1219:dbl)
                    n441 = local read "StripStepRb"() -> (w1223:dbl)
                    n442 = Equal?(x=w1220, y=enum16{"Main motion", "Strip motion"}."Main motion") -> (x = y?=w1226:bool)
                    n443 = Select(t=w1221, s=w1226, f=w1219) -> (s? t:f=w1225:dbl)
                    n444 = Multiply(x=w1223, y=w1222) -> (x*y=w1224:dbl)
                    n445 = Multiply(x=w1224, y=w1225) -> (x*y=w1227:dbl)
                    n446 = Add(x=w1227, y=w1217) -> (x+y=w1216:dbl)
                  }
                }
                n447 = call "Move absolute.vi"("Zaber"=w1117, "Position, mm"=w1118, "error in"=w1116) -> ("Zaber out"=w1109:T1, "error out"=w1114:errorcluster)  [unwired: 13 in, 2 out]
                n448 = call "Delay.vi"("Delay, ms"=u32 1000, "error in"=w1114) -> ("error out"=w1112:errorcluster)  [unwired: 17 in]
                n449 = case shown="\"Shear force sensor\"" w1113 {
                  tunnel: w1109 -> [w1120 w1122 w1129 w1166]
                  tunnel: w1112 -> [w1121 w1126 w1131 w1168]
                  tunnel: w1108 -> [_ _ w1130 w1167]
                  tunnel: [w1121 w1123 w1127 w1165] -> w1111
                  tunnel: [w1120 w1122 w1128 w1164] -> w1110
                  frame "Simple plane", Default {
                  }
                  frame "Keyence sensor" {
                    n450 = local read "Keyence"() -> (w1125:T4)
                    n451 = call "Get value OUT1.vi"("Keyence"=w1125, "error in"=w1126) -> ("Distance"=→"StartDistance":dbl, "error out"=w1123:errorcluster)  [unwired: 14 in, 2 out]
                  }
                  frame "Shear force sensor" {
                    n452 = while {
                      tunnel: w1131 -> [w1146]
                      tunnel: w1130 -> [w1139]
                      tunnel: w1129 -> [w1134]
                      tunnel: [w1133] -> w1128
                      tunnel: [w1132] -> w1127
                      stop <- w1138 stop-if-true
                      w1148 = T24 2 items=["X", "Y", "R", "Theta", "IN1", "IN2", "IN3", "IN4", "OUT1", "OUT2", "XNoise", "YNoise", "Phase", "SineOut", "DCLevel", "IntRefFreq", "ExtRefFreq"] ("DataChannel")
                      # "tip landing"
                      n453 = local read "SR865"() -> (w1147:T6)
                      n454 = local read "SFMWorkingLevel"() -> (w1143:dbl)
                      n455 = call "DataChannelRead.vi"("SR865 in"=w1147, "DataChannel"=w1148, "error in"=w1146) -> ("Signal"=w1144:dbl, "error out"=w1135:errorcluster)  [unwired: 14 in, 1 out]
                      n456 = Subtract(x=w1144, y=w1143) -> (x-y=w1136:dbl)
                      n457 = Absolute Value(x=w1136) -> (abs(x)=w1145:dbl)
                      n458 = Not Equal?(x=w1139, y=enum16{"Idle", "Working", "Stopping"}."Working") -> (x != y?=w1140:bool)
                      n459 = Less Or Equal?(x=w1145, y="SFMStayRange") -> (x <= y?=w1137:bool)
                      n460 = Or(x=w1140, y=w1137) -> (x .or. y?=w1138:bool)
                      n461 = case shown="False" w1137 {
                        tunnel: w1136 -> [w1155 _]
                        tunnel: w1135 -> [w1152 w1162]
                        tunnel: w1134 -> [w1151 w1163]
                        tunnel: [w1150 w1163] -> w1133
                        tunnel: [w1149 w1162] -> w1132
                        frame False {
                          n462 = Absolute Value(x="SFMSlope") -> (abs(x)=w1157:dbl)
                          n463 = Multiply(x="SFMSlope", y=w1155) -> (x*y=w1160:dbl)
                          n464 = Greater Than 0?(x=w1160) -> (x > 0?=w1161:bool)
                          n465 = Negate(x=w1157) -> (-x=w1158:dbl)
                          n466 = Select(t=w1158, s=w1161, f=w1157) -> (s? t:f=w1159:dbl)
                          n467 = Add(x=w1159, y=0.0) -> (x+y=w1153:dbl)
                          n468 = call "Move relative.vi"("Zaber"=w1151, "Distance, mm"=w1153, "error in"=w1152) -> ("Zaber out"=w1150:T1, "error out"=w1149:errorcluster)  [unwired: 13 in, 2 out]
                        }
                        frame True {
                        }
                      }
                    }
                  }
                  frame "SICM sensor" {
                    n469 = while {
                      tunnel: w1168 -> [w1185]
                      tunnel: w1167 -> [w1175]
                      tunnel: w1166 -> [w1172]
                      tunnel: [w1171] -> w1165
                      tunnel: [w1170] -> w1164
                      stop <- w1176 stop-if-true
                      # "tip landing"
                      n470 = local read "RBD9103"() -> (w1183:T5)
                      n471 = call "Delay.vi"("Delay, ms"=u32 1000, "error in"=w1185) -> ("error out"=w1184:errorcluster)  [unwired: 17 in]
                      n472 = call "Read.vi"("RBD9103"=w1183, "error in"=w1184) -> ("Value, nA"=w1181:dbl, "error out"=w1169:errorcluster)  [unwired: 12 in, 4 out]
                      "Value, nA" <- w1181
                      n473 = Subtract(x=w1181, y="SIMWorkingLevel") -> (x-y=w1173:dbl)
                      n474 = Absolute Value(x=w1173) -> (abs(x)=w1182:dbl)
                      n475 = Less Or Equal?(x=w1182, y="SIMStayRange") -> (x <= y?=w1174:bool)
                      n476 = Not Equal?(x=w1175, y=enum16{"Idle", "Working", "Stopping"}."Working") -> (x != y?=w1177:bool)
                      n477 = Or(x=w1177, y=w1174) -> (x .or. y?=w1176:bool)
                      n478 = case shown="True" w1174 {
                        tunnel: w1173 -> [w1198 _]
                        tunnel: w1172 -> [w1199 w1201]
                        tunnel: w1169 -> [w1200 w1202]
                        tunnel: [w1188 w1202] -> w1171
                        tunnel: [w1187 w1201] -> w1170
                        frame False {
                          n479 = Greater Than 0?(x=w1198) -> (x > 0?=w1194:bool)
                          n480 = call "Get position.vi"("Zaber"=w1199, "error in"=w1200) -> ("Zaber out"=w1192:T1, "PositionRb"=w1193:dbl, "error out"=w1191:errorcluster)  [unwired: 13 in, 2 out]
                          "PositionRb" <- w1193
                          n481 = Select(t=0.0001, s=w1194, f=-0.0005) -> (s? t:f=w1197:dbl)
                          n482 = Add(x=w1193, y=w1197) -> (x+y=w1190:dbl)
                          "Calculated position" <- w1190
                          n483 = call "Move absolute.vi"("Zaber"=w1192, "Position, mm"=w1190, "error in"=w1191) -> ("Zaber out"=w1187:T1, "Position, mm"=→"Position, mm":dbl, "error out"=w1188:errorcluster)  [unwired: 13 in, 1 out]
                        }
                        frame True {
                        }
                      }
                    }
                  }
                }
              }
              frame #1 {
                # "Finally, wait for a period to \ngenerate droplet on tissue."
                n484 = Multiply(x="Landing dwell, s", y=1000.0) -> (x*y=w1228:dbl)
                n485 = Wait (ms)(milliseconds to wait=w1228) -> ()  [unwired: 1 out]
              }
            }
          }
        }
      }
      frame "MS Trig" {
      }
      frame "Line Motion" {
        # "Main X/Y motion for line scan\nAfter determine the main motion direction\nonly need to take: 1. velocity 2. end position"
        # "Stop timed loop at end of line"
        n486 = local read "Status"() -> (w1254:T11)
        n487 = case shown="\"Working\", \"Pause\"" w1254 {
          tunnel: w1253 -> [w1263 w1294]
          tunnel: w1252 -> [w1264 w1295]
          tunnel: w1243 -> [w1262 w1309]
          tunnel: [w1262 w1300] -> w1246
          tunnel: [w1264 w1298] -> w1251
          tunnel: [w1263 w1297] -> w1250
          tunnel: w1243 -> [_ w1292]
          tunnel: w1249 -> [w1261 w1290]
          tunnel: [w1261 w1289] -> w1248
          tunnel: w1245 -> [w1259 w1270]
          tunnel: [w1259 w1269] -> w1244
          tunnel: w1243 -> [_ w1268]
          frame "Idle", Default {
            n488 = local write "MS ever Trig?"(FALSE) -> ()
          }
          frame "Working", "Pause" {
            # "Controls Z motion and populates height data array while XY motion is in progress"
            n489 = flat-sequence {
              tunnel: w1268 -> [w1319]
              tunnel: w1270 -> [w1320]
              tunnel: [w1320] -> w1266
              tunnel: [w1319] -> w1265
              tunnel: [w1327] -> w1274
              tunnel: [w1324] -> w1273
              tunnel: w1266 -> [w1332]
              tunnel: w1265 -> [w1321]
              tunnel: w1274 -> [w1335]
              tunnel: w1273 -> [w1334]
              tunnel: [w1335] -> w1272
              tunnel: [w1334] -> w1271
              tunnel: w1272 -> [w1342]
              tunnel: w1271 -> [w1339]
              tunnel: [w1338] -> w1269
              tunnel: [w1337] -> w1267
              frame #0 {
                # "Wait until the pre-scan finishes"
                n490 = Multiply(x="Pre-scan time, s", y=1000.0) -> (x*y=w1316:dbl)
                n491 = Subtract(x=w1316, y=1000.0) -> (x-y=w1314:dbl)
                n492 = Wait (ms)(milliseconds to wait=w1314) -> ()  [unwired: 1 out]
              }
              frame #1 {
                # "Start Bruker or LTQ\nPrepare data  array"
                n493 = local read "LineZData"() -> (w1326:cluster{cluster{dbl, dbl}[]}[])
                n494 = call-poly <vilib>:"DAQmx Write.vi"("task/channels in"=w1332, "data"=FALSE, "timeout"=0.0, "error in"=w1321) -> ("task out"=w1327:refnum<k21>, "error out"=w1329:errorcluster)  [unwired: 1 in, 9 out]
                n495 = call "Erase.vi"("Data"=w1326) -> ("Data"=w1325:cluster{cluster{dbl, dbl}[]}[])  [unwired: 18 in]
                n496 = call "GetTickCount.vi"("error in (no error)"=w1329) -> ("ms"=→"MS start":u32, "error IO"=w1324:errorcluster)  [unwired: 17 in]
                n497 = local write "LineZData"(w1325) -> ()
                "MS ever Trig?" <- TRUE
                "CC start" <- TRUE ("CC start")
              }
              frame #2 {
                n498 = Wait (ms)(milliseconds to wait=u32 1000) -> ()  [unwired: 1 out]
              }
              frame #3 {
                n499 = local write "CC start"(FALSE ("CC start")) -> ()
                n500 = call-poly <vilib>:"DAQmx Write.vi"("task/channels in"=w1342, "data"=TRUE, "timeout"=0.0, "error in"=w1339) -> ("task out"=w1338:refnum<k21>, "error out"=w1337:errorcluster)  [unwired: 1 in, 9 out]
              }
            }
            n501 = local read "LineZData"() -> (w1286:cluster{cluster{dbl, dbl}[]}[])
            n502 = local read "Method"() -> (w1293:T9)
            n503 = local read "dt"() -> (w1288:dbl)
            n504 = local read "t0"() -> (w1287:dbl)
            n505 = case shown="\"3 point plane\"" w1293 {
              tunnel: w1292 -> [w1355 w1402 w1475 w1557 w1627 w1637]
              tunnel: [w1351 w1400 w1474 w1555 w1627 w1631] -> w1284
              tunnel: w1290 -> [w1353 w1399 w1473 w1556 w1628 w1635]
              tunnel: [w1350 w1396 w1472 w1554 FALSE w1630] -> w1277
              tunnel: [w1352 w1397 w1471 w1553 w1628 w1632] -> w1289
              tunnel: w1288 -> [w1356 _ _ _ _ w1638]
              tunnel: w1287 -> [w1354 _ _ _ _ w1636]
              tunnel: w1286 -> [w1349 w1401 w1470 w1552 w1626 w1634]
              tunnel: [w1348 w1398 w1469 w1551 w1626 w1633] -> w1285
              frame "Simple plane" {
                n506 = node-c288(w1356, w1355, w1354) -> (w1358:T18)  [unwired: 1 in]
                n507 = timed-loop {
                  timing: w1358 -> [_]
                  timing-out: [_] -> w1357
                  shift-right: [w1374] -> w1352
                  shift-left: w1353 -> [w1375]
                  tunnel: [w1359] -> w1350
                  shift-right: [w1368] -> w1348
                  shift-left: w1349 -> [w1369]
                  i -> [w1381]
                  stop <- w1362 stop-if-true
                  n508 = node-c288() -> (w1376:errorcluster, w1382:bool)  [unwired: 1 in]
                  n509 = local read "ZStartPosition"() -> (w1377:dbl)
                  n510 = local read "PZRealStep"() -> (w1379:dbl)
                  n511 = Increment(x=w1381) -> (x+1=w1380:i32)
                  n512 = local write "PZJump"(w1380) -> ()
                  n513 = Multiply(x=w1380, y=w1379) -> (x*y=w1378:dbl)
                  n514 = local write "BtnLoopWasLate"(w1382) -> ()
                  n515 = Add(x=w1378, y=w1377) -> (x+y=w1370:dbl)
                  n516 = call "Move absolute.vi"("Zaber"=w1375, "Position, mm"=w1370, "error in"=w1376) -> ("Start time, ms"=w1371:u32, "Zaber out"=w1374:T1, "error out"=w1373:errorcluster)  [unwired: 13 in, 1 out]
                  n517 = local read "LineMotion"() -> (w1360:bool)
                  n518 = local read "Status"() -> (w1361:T11)
                  n519 = call "Append.vi"("Data"=w1369, "Plot"=0, "X"=w1371, "Y"=w1370) -> ("Data"=w1368:cluster{cluster{dbl, dbl}[]}[])  [unwired: 15 in]
                  n520 = Not Equal?(x=w1361, y=enum16{"Idle", "Working", "Stopping"}."Working") -> (x != y?=w1363:bool)
                  n521 = Not Equal?(x=w1361, y=Status."Pause") -> (x != y?=w1364:bool)
                  n522 = Not(x=w1360) -> (.not. x?=w1366:bool)
                  n523 = And(x=w1363, y=w1364) -> (x .and. y?=w1359:bool)
                  n524 = node-c288(w1373) -> ()  [unwired: 1 out]
                  n525 = Or(x=w1359, y=w1366) -> (x .or. y?=w1362:bool)
                }
                n526 = node-c288(w1357) -> (w1351:errorcluster)
              }
              frame "Keyence sensor" {
                n527 = node-c288(i64 60 ("Period"), w1402) -> (w1405:T18)  [unwired: 1 in]
                n528 = timed-loop {
                  timing: w1405 -> [_]
                  timing-out: [_] -> w1404
                  shift-right: [w1415] -> w1398
                  shift-left: w1401 -> [w1429]
                  shift-right: [w1417] -> w1397
                  shift-left: w1399 -> [w1418]
                  tunnel: [w1406] -> w1396
                  stop <- w1409 stop-if-true
                  n529 = node-c288() -> (w1440:errorcluster, w1422:bool)  [unwired: 1 in]
                  n530 = local write "BtnLoopWasLate"(w1422) -> ()
                  n531 = local read "Keyence"() -> (w1438:T4)
                  n532 = call "GetTickCount.vi"("error in (no error)"=w1440) -> ("ms"=w1436:u32, "error IO"=w1439:errorcluster)  [unwired: 17 in]
                  n533 = local read "StartDistance"() -> (w1433:dbl)
                  n534 = call "Get value OUT2.vi"("Keyence"=w1438, "error in"=w1439) -> ("Start transfer"=w1431:u32, "Distance"=w1432:dbl, "error out"=w1420:errorcluster)  [unwired: 13 in, 2 out]
                  "Distance" <- w1432
                  n535 = Subtract(x=w1433, y=w1432) -> (x-y=w1423:dbl)
                  "MoveDistance" <- w1423
                  n536 = call "Append.vi"("Data"=w1429, "Plot"=2, "X"=w1431, "Y"=w1423) -> ("Data"=w1416:cluster{cluster{dbl, dbl}[]}[])  [unwired: 15 in]
                  n537 = Absolute Value(x=w1423) -> (abs(x)=w1428:dbl)
                  n538 = In Range and Coerce(upper limit="ZMaxToMoveDistance", x=w1428, lower limit="ZMinToMoveDistanceancy") -> (In Range?=w1424:bool)  [unwired: 1 out]
                  n539 = local read "LineMotion"() -> (w1408:bool)
                  n540 = local read "Status"() -> (w1407:T11)
                  n541 = Select(t=w1423, s=w1424, f=0.0) -> (s? t:f=w1421:dbl)
                  "RealMoveDistance" <- w1421
                  n542 = Not Equal?(x=w1407, y=enum16{"Idle", "Working", "Stopping"}."Working") -> (x != y?=w1410:bool)
                  n543 = Not Equal?(x=w1407, y=Status."Pause") -> (x != y?=w1411:bool)
                  n544 = Not(x=w1408) -> (.not. x?=w1413:bool)
                  n545 = case shown="1, Default" w1421 {
                    tunnel: w1421 -> [_ w1456]
                    tunnel: w1420 -> [w1441 w1452]
                    tunnel: [w1441 w1451] -> w1419
                    tunnel: [w1443 w1447] -> w1415
                    tunnel: w1418 -> [w1442 w1446]
                    tunnel: [w1442 w1445] -> w1417
                    tunnel: w1416 -> [w1443 w1444]
                    frame 0 {
                    }
                    frame 1, Default {
                      n546 = Divide(x=w1456, y="ZFactor") -> (x/y=w1454:dbl)
                      n547 = Divide(x=w1454, y=1000.0) -> (x/y=w1448:dbl)
                      n548 = call "Start relative move.vi"("Zaber"=w1446, "Distance, mm"=w1448, "error in"=w1452) -> ("Start time, ms"=w1449:u32, "Zaber out"=w1445:T1, "error out"=w1451:errorcluster)  [unwired: 14 in]
                      n549 = call "Append.vi"("Data"=w1444, "Plot"=0, "X"=w1449, "Y"=w1448) -> ("Data"=w1447:cluster{cluster{dbl, dbl}[]}[])  [unwired: 15 in]
                    }
                  }
                  n550 = And(x=w1410, y=w1411) -> (x .and. y?=w1406:bool)
                  n551 = Or(x=w1406, y=w1413) -> (x .or. y?=w1409:bool)
                  n552 = call "GetTickCount.vi"("error in (no error)"=w1419) -> ("ms"=w1437:u32, "error IO"=w1434:errorcluster)  [unwired: 17 in]
                  n553 = Subtract(x=w1437, y=w1436) -> (x-y=→"Loop time":u32)
                  n554 = node-c288(w1434) -> ()  [unwired: 1 out]
                }
                n555 = node-c288(w1404) -> (w1400:errorcluster)
              }
              frame "Shear force sensor" {
                n556 = node-c288("SFMLoopTime", w1475) -> (w1478:T18)  [unwired: 1 in]
                n557 = timed-loop {
                  timing: w1478 -> [_]
                  timing-out: [_] -> w1477
                  tunnel: [w1479] -> w1472
                  shift-right: [w1486] -> w1471
                  shift-left: w1473 -> [w1513]
                  shift-right: [w1484] -> w1469
                  shift-left: w1470 -> [w1485]
                  stop <- w1488 stop-if-true
                  w1514 = T24 2 items=["X", "Y", "R", "Theta", "IN1", "IN2", "IN3", "IN4", "OUT1", "OUT2", "XNoise", "YNoise", "Phase", "SineOut", "DCLevel", "IntRefFreq", "ExtRefFreq"] ("DataChannel")
                  n558 = node-c288() -> (w1517:errorcluster, →"BtnLoopWasLate":bool)  [unwired: 1 in]
                  n559 = local read "SFMWorkingLevel"() -> (w1510:dbl)
                  n560 = local read "SFMStayRange"() -> (w1509:dbl)
                  n561 = local read "SR865"() -> (w1515:T6)
                  n562 = call "GetTickCount.vi"("error in (no error)"=w1517) -> ("ms"=w1496:u32, "error IO"=w1516:errorcluster)  [unwired: 17 in]
                  n563 = call "DataChannelRead.vi"("SR865 in"=w1515, "DataChannel"=w1514, "error in"=w1516) -> ("Signal"=w1511:dbl, "error out"=w1497:errorcluster)  [unwired: 14 in, 1 out]
                  n564 = Subtract(x=w1511, y=w1510) -> (x-y=w1506:dbl)
                  n565 = call "GetTickCount.vi"("error in (no error)"=w1497) -> ("ms"=w1492:u32)  [unwired: 17 in, 1 out]
                  n566 = call "Get position.vi"("Zaber"=w1513, "error in"=w1497) -> ("Command time, ms"=w1505:u32, "Zaber out"=w1507:T1, "PositionRb"=w1504:dbl, "error out"=w1494:errorcluster)  [unwired: 13 in, 1 out]
                  n567 = Absolute Value(x=w1506) -> (abs(x)=w1512:dbl)
                  n568 = Less Or Equal?(x=w1512, y=w1509) -> (x <= y?=w1508:bool)
                  n569 = Subtract(x=w1492, y=w1496) -> (x-y=→"Amp dead time":u32)
                  n570 = call "GetTickCount.vi"("error in (no error)"=w1494) -> ("ms"=w1493:u32)  [unwired: 17 in, 1 out]
                  n571 = Subtract(x=w1493, y=w1492) -> (x-y=→"Read position":u32)
                  n572 = call "Append.vi"("Data"=w1485, "Plot"=1, "X"=w1505, "Y"=w1504) -> ("Data"=w1502:cluster{cluster{dbl, dbl}[]}[])  [unwired: 15 in]
                  n573 = case shown="False" w1508 {
                    tunnel: w1507 -> [w1527 w1538]
                    tunnel: w1494 -> [w1526 w1537]
                    tunnel: w1506 -> [w1530 _]
                    tunnel: w1504 -> [w1528 _]
                    tunnel: [w1525 w1538] -> w1486
                    tunnel: [w1524 w1537] -> w1501
                    tunnel: w1502 -> [w1520 w1536]
                    tunnel: [w1519 w1536] -> w1484
                    frame False {
                      n574 = local read "SFMSlope"() -> (w1529:dbl)
                      n575 = Absolute Value(x=w1529) -> (abs(x)=w1531:dbl)
                      n576 = Multiply(x=w1529, y=w1530) -> (x*y=w1533:dbl)
                      n577 = Greater Than 0?(x=w1533) -> (x > 0?=w1535:bool)
                      n578 = Negate(x=w1531) -> (-x=w1532:dbl)
                      n579 = Select(t=w1532, s=w1535, f=w1531) -> (s? t:f=w1534:dbl)
                      n580 = Add(x=w1528, y=w1534) -> (x+y=w1522:dbl)
                      n581 = call "Start absolute move.vi"("Zaber"=w1527, "Position, mm"=w1522, "error in"=w1526) -> ("Start time, ms"=w1523:u32, "Zaber out"=w1525:T1, "error out"=w1524:errorcluster)  [unwired: 14 in]
                      n582 = call "Append.vi"("Data"=w1520, "Plot"=0, "X"=w1523, "Y"=w1522) -> ("Data"=w1519:cluster{cluster{dbl, dbl}[]}[])  [unwired: 15 in]
                    }
                    frame True {
                    }
                  }
                  n583 = local read "LineMotion"() -> (w1487:bool)
                  n584 = local read "Status"() -> (w1483:T11)
                  n585 = Not Equal?(x=w1483, y=enum16{"Idle", "Working", "Stopping"}."Working") -> (x != y?=w1480:bool)
                  n586 = Not Equal?(x=w1483, y=Status."Pause") -> (x != y?=w1481:bool)
                  n587 = Not(x=w1487) -> (.not. x?=w1489:bool)
                  n588 = And(x=w1480, y=w1481) -> (x .and. y?=w1479:bool)
                  n589 = Or(x=w1479, y=w1489) -> (x .or. y?=w1488:bool)
                  n590 = call "GetTickCount.vi"("error in (no error)"=w1501) -> ("ms"=w1500:u32, "error IO"=w1498:errorcluster)  [unwired: 17 in]
                  n591 = Subtract(x=w1500, y=w1496) -> (x-y=→"ShF loop time":u32)
                  n592 = node-c288(w1498) -> ()  [unwired: 1 out]
                }
                n593 = node-c288(w1477) -> (w1474:errorcluster)
              }
              frame "SICM sensor" {
                n594 = node-c288("SIMLoopTime", w1557, 60000 ("Priority")) -> (w1561:T18)  [unwired: 1 in]
                n595 = timed-loop {
                  timing: w1561 -> [_]
                  timing-out: [_] -> w1560
                  shift-right: [w1574] -> w1553
                  shift-left: w1556 -> [w1589]
                  tunnel: [w1562] -> w1554
                  shift-right: [w1571] -> w1551
                  shift-left: w1552 -> [w1572]
                  stop <- w1563 stop-if-true
                  n596 = node-c288() -> (w1592:errorcluster, →"BtnSIMLoopWasLate":bool)  [unwired: 1 in]
                  n597 = local read "SIMWorkingLevel"() -> (w1591:dbl)
                  n598 = local read "RBD9103"() -> (w1593:T5)
                  n599 = local read "SIMStayRange"() -> (w1590:dbl)
                  n600 = call "Read.vi"("RBD9103"=w1593, "error in"=w1592) -> ("Command time, ms"=w1581:u32, "Value, nA"=w1580:dbl, "error out"=w1588:errorcluster)  [unwired: 12 in, 3 out]
                  n601 = Subtract(x=w1580, y=w1591) -> (x-y=w1583:dbl)
                  n602 = local write "Value, nA"(w1580) -> ()
                  n603 = call "Get position.vi"("Zaber"=w1589, "error in"=w1588) -> ("Command time, ms"=w1577:u32, "Zaber out"=w1587:T1, "PositionRb"=w1575:dbl, "error out"=w1584:errorcluster)  [unwired: 13 in, 1 out]
                  n604 = Absolute Value(x=w1583) -> (abs(x)=w1585:dbl)
                  n605 = Less Or Equal?(x=w1585, y=w1590) -> (x <= y?=w1586:bool)
                  n606 = call "Append.vi"("Data"=w1572, "Plot"=2, "X"=w1581, "Y"=w1580) -> ("Data"=w1579:cluster{cluster{dbl, dbl}[]}[])  [unwired: 15 in]
                  n607 = local write "PositionRb"(w1575) -> ()
                  n608 = call "Append.vi"("Data"=w1579, "Plot"=1, "X"=w1577, "Y"=w1575) -> ("Data"=w1576:cluster{cluster{dbl, dbl}[]}[])  [unwired: 15 in]
                  n609 = case shown="False" w1586 {
                    tunnel: w1587 -> [w1603 w1611]
                    tunnel: w1584 -> [w1602 w1610]
                    tunnel: w1583 -> [w1605 _]
                    tunnel: w1575 -> [w1604 _]
                    tunnel: [w1601 w1610] -> w1573
                    tunnel: [w1600 w1611] -> w1574
                    tunnel: w1576 -> [w1596 w1612]
                    tunnel: [w1595 w1612] -> w1571
                    frame False {
                      n610 = Greater Than 0?(x=w1605) -> (x > 0?=w1609:bool)
                      n611 = Select(t=0.0001, s=w1609, f=-0.0005) -> (s? t:f=w1606:dbl)
                      n612 = Add(x=w1604, y=w1606) -> (x+y=w1598:dbl)
                      n613 = local write "Calculated position"(w1598) -> ()
                      n614 = call "Start absolute move.vi"("Zaber"=w1603, "Position, mm"=w1598, "error in"=w1602) -> ("Start time, ms"=w1599:u32, "Zaber out"=w1600:T1, "error out"=w1601:errorcluster)  [unwired: 14 in]
                      n615 = call "Append.vi"("Data"=w1596, "Plot"=0, "X"=w1599, "Y"=w1598) -> ("Data"=w1595:cluster{cluster{dbl, dbl}[]}[])  [unwired: 15 in]
                    }
                    frame True {
                    }
                  }
                  n616 = local read "LineMotion"() -> (w1564:bool)
                  n617 = local read "Status"() -> (w1565:T11)
                  n618 = Not Equal?(x=w1565, y=enum16{"Idle", "Working", "Stopping"}."Working") -> (x != y?=w1566:bool)
                  n619 = Not Equal?(x=w1565, y=Status."Pause") -> (x != y?=w1567:bool)
                  n620 = Not(x=w1564) -> (.not. x?=w1569:bool)
                  n621 = And(x=w1566, y=w1567) -> (x .and. y?=w1562:bool)
                  n622 = Or(x=w1562, y=w1569) -> (x .or. y?=w1563:bool)
                  n623 = node-c288(w1573) -> ()  [unwired: 1 out]
                }
                n624 = node-c288(w1560) -> (w1555:errorcluster)
              }
              frame Default {
              }
              frame "3 point plane" {
                n625 = node-c288(w1638, w1637, w1636) -> (w1640:T18)  [unwired: 1 in]
                n626 = timed-loop {
                  timing: w1640 -> [_]
                  timing-out: [_] -> w1639
                  shift-right: [w1657] -> w1632
                  shift-left: w1635 -> [w1658]
                  shift-right: [w1651] -> w1633
                  shift-left: w1634 -> [w1652]
                  tunnel: [w1641] -> w1630
                  i -> [w1660]
                  stop <- w1642 stop-if-true
                  n627 = node-c288() -> (w1674:errorcluster, w1673:bool)  [unwired: 1 in]
                  n628 = local read "XStageType"() -> (w1663:enum16{"Main motion", "Strip motion"})
                  n629 = local read "StripStepRb"() -> (w1666:dbl)
                  n630 = local read "StripLineRb"() -> (w1665:u32)
                  n631 = local read "PlaneZx"() -> (w1650:dbl)
                  n632 = local read "PlaneZy"() -> (w1664:dbl)
                  n633 = local read "PZRealStep"() -> (w1661:dbl)
                  n634 = local write "BtnLoopWasLate"(w1673) -> ()
                  n635 = Equal?(x=w1663, y=enum16{"Main motion", "Strip motion"}."Main motion") -> (x = y?=w1669:bool)
                  n636 = local read "ZStartPosition"() -> (w1662:dbl)
                  n637 = Increment(x=w1660) -> (x+1=w1659:i32)
                  n638 = Select(t=w1664, s=w1669, f=w1650) -> (s? t:f=w1668:dbl)
                  n639 = Multiply(x=w1666, y=w1665) -> (x*y=w1667:dbl)
                  n640 = Multiply(x=w1661, y=w1659) -> (x*y=w1672:dbl)
                  n641 = Multiply(x=w1667, y=w1668) -> (x*y=w1670:dbl)
                  n642 = local write "PZJump"(w1659) -> ()
                  n643 = Compound Arithmetic op=ADD(w1670, w1662, w1672) -> (w1655:dbl)
                  n644 = local read "LineMotion"() -> (w1643:bool)
                  n645 = local read "Status"() -> (w1644:T11)
                  n646 = call "Move absolute.vi"("Zaber"=w1658, "Position, mm"=w1655, "error in"=w1674) -> ("Start time, ms"=w1654:u32, "Zaber out"=w1657:T1, "error out"=w1656:errorcluster)  [unwired: 13 in, 1 out]
                  n647 = Not Equal?(x=w1644, y=enum16{"Idle", "Working", "Stopping"}."Working") -> (x != y?=w1645:bool)
                  n648 = Not Equal?(x=w1644, y=Status."Pause") -> (x != y?=w1646:bool)
                  n649 = Not(x=w1643) -> (.not. x?=w1648:bool)
                  n650 = call "Append.vi"("Data"=w1652, "Plot"=0, "X"=w1654, "Y"=w1655) -> ("Data"=w1651:cluster{cluster{dbl, dbl}[]}[])  [unwired: 15 in]
                  n651 = And(x=w1645, y=w1646) -> (x .and. y?=w1641:bool)
                  n652 = Or(x=w1641, y=w1648) -> (x .or. y?=w1642:bool)
                  n653 = node-c288(w1656) -> ()  [unwired: 1 out]
                }
                n654 = node-c288(w1639) -> (w1631:errorcluster)
              }
            }
            n655 = local read "XStageType"() -> (w1313:enum16{"Main motion", "Strip motion"})
            n656 = Equal?(x=w1313, y=enum16{"Main motion", "Strip motion"}."Main motion") -> (x = y?=w1296:bool)
            n657 = local read "BtnDLADS"() -> (w1276:bool)
            n658 = case shown="True" w1276 {
              tunnel: [w1344 w1347] -> w1305
              tunnel: w1296 -> [w1343 _]
              frame False {
                n659 = local read "XEndPosition"() -> (w1346:dbl)
                n660 = local read "YEndPosition"() -> (w1345:dbl)
                n661 = Select(t=w1346, s=w1343, f=w1345) -> (s? t:f=w1344:dbl)
              }
              frame True {
                n662 = local read "Main motion \nend position"() -> (w1347:dbl)
              }
            }
            n663 = Select(t=w1294, s=w1296, f=w1295) -> (s? t:f=w1311:T1)
            n664 = local read "Velocity"() -> (w1308:dbl)
            n665 = call "Get velocity.vi"("Zaber"=w1311, "error in"=w1309) -> ("Zaber out"=w1310:T1, "Velocity, mm/s"=w1301:dbl, "error out"=w1307:errorcluster)  [unwired: 14 in, 1 out]
            n666 = call "Set velocity.vi"("Zaber in"=w1310, "Velocity, mm/s"=w1308, "error in"=w1307) -> ("Zaber out"=w1283:T1, "error out"=w1306:errorcluster)  [unwired: 14 in, 1 out]
            n667 = call "Move absolute.vi"("Zaber"=w1283, "Position, mm"=w1305, "error in"=w1306) -> ("Start time, ms"=→"MotionStartTime":u32, "Zaber out"=w1279:T1, "error out"=w1303:errorcluster)  [unwired: 13 in, 1 out]
            n668 = property on="LineMotion" class="Bool (strict)"(error in=w1303, "Value"=FALSE ("LineMotion")) -> (error out=w1291:errorcluster)  [unwired: 1 in, 1 out]
            n669 = case shown="True" w1277 {
              tunnel: w1283 -> [w1693 w1697]
              tunnel: w1284 -> [w1692 w1696]
              tunnel: [w1693 w1695] -> w1280
              tunnel: [w1692 w1694] -> w1282
              frame False {
              }
              frame True {
                n670 = call "Stop move.vi"("Zaber"=w1697, "error in"=w1696) -> ("Zaber out"=w1695:T1, "error out"=w1694:errorcluster)  [unwired: 16 in]
              }
            }
            n671 = local write "LineZData"(w1285) -> ()
            n672 = Merge Errors(w1282, w1291, w1267) -> (w1281:errorcluster)
            n673 = Select(t=w1280, s=w1277, f=w1279) -> (s? t:f=w1278:T1)
            n674 = call "Set velocity.vi"("Zaber in"=w1278, "Velocity, mm/s"=w1301, "error in"=w1281) -> ("Zaber out"=w1299:T1, "error out"=w1300:errorcluster)  [unwired: 14 in, 1 out]
            n675 = case shown="True" w1296 {
              tunnel: w1299 -> [w1689 w1691]
              tunnel: [w1689 w1690] -> w1298
              tunnel: [w1688 w1691] -> w1297
              tunnel: w1295 -> [_ w1690]
              tunnel: w1294 -> [w1688 _]
              frame False {
              }
              frame True {
              }
            }
            "LineMotion" <- TRUE ("MainLine Motion")
          }
        }
      }
      frame "Z Exit Ctrl" {
        # "is this a 2d or line profile?\ndouble check and delete 2d plot function."
        n676 = local read "Status"() -> (w1702:T11)
        n677 = local read "MS ever Trig?"() -> (w1708:bool)
        n678 = case shown="\"Working\"" w1702 {
          tunnel: w1701 -> [w1723 w1741 w1744]
          tunnel: [w1722 w1740 w1744] -> w1700
          tunnel: w1699 -> [w1721 w1739 w1743]
          tunnel: [w1720 w1738 w1743] -> w1698
          frame "Working" {
            # "Move tip to Zout position"
            n679 = flat-sequence {
              tunnel: w1723 -> [w1728]
              tunnel: w1721 -> [w1726]
              tunnel: [w1727] -> w1719
              tunnel: [w1725] -> w1718
              tunnel: w1719 -> [w1734]
              tunnel: w1718 -> [w1733]
              tunnel: [w1734] -> w1717
              tunnel: [w1733] -> w1716
              tunnel: [w1736] -> w1720
              tunnel: [w1737] -> w1722
              tunnel: w1717 -> [w1737]
              tunnel: w1716 -> [w1736]
              frame #0 {
                n680 = local read "ZOutPosition"() -> (w1729:dbl)
                n681 = call "Move absolute.vi"("Zaber"=w1728, "Position, mm"=w1729, "error in"=w1726) -> ("Zaber out"=w1727:T1, "error out"=w1725:errorcluster)  [unwired: 13 in, 2 out]
                "MS dwell" <- TRUE ("MS dwell")
              }
              frame #1 {
                # "Wait when 1. QTOF gets ready  (and 2. DLADS computation)"
                n682 = Multiply(x="MSDwellTimeInSec", y=1000) -> (x*y=w1731:dbl)
                n683 = Wait (ms)(milliseconds to wait=w1731) -> ()  [unwired: 1 out]
              }
              frame #2 {
                n684 = local write "MS dwell"(FALSE ("MS dwell")) -> ()
              }
            }
          }
          frame "Pause" {
            # "Move tip to Zout position"
            n685 = local read "ZOutPosition"() -> (w1742:dbl)
            n686 = call "Move absolute.vi"("Zaber"=w1741, "Position, mm"=w1742, "error in"=w1739) -> ("Zaber out"=w1740:T1, "error out"=w1738:errorcluster)  [unwired: 13 in, 2 out]
          }
          frame "Idle", Default {
          }
        }
        n687 = case shown="True" w1708 {
          tunnel: [T13[] [] T13[] [{"Action"=enum."Plot Profile", "1"=FALSE, "2"=FALSE, "3"=FALSE}]] -> w1704
          frame False {
          }
          frame True {
            # "0: Plot profile"
          }
        }
        n688 = call "Add to Queue.vi"("error in (no error)"=w1698, "Front? (F)"=TRUE, "Actions"=w1704, "Queue Ref In"=w1707) -> ("error out"=w1703:errorcluster, "Queue Ref Out"=w1705:refnum<queue>)  [unwired: 6 in]
      }
      frame "MS Complete" {
        # "Agilent mass spectrometer CC could work the same way as Brucker mass spec.\nThough for Brucker, the pulse interval was set to be 1ms."
        n689 = local read "MS ever Trig?"() -> (w1752:bool)
        n690 = case shown="True" w1752 {
          tunnel: w1751 -> [w1761 w1769]
          tunnel: w1748 -> [w1760 w1768]
          tunnel: [w1761 w1765] -> w1750
          tunnel: [w1760 w1764] -> w1747
          frame False {
          }
          frame True {
            n691 = flat-sequence {
              tunnel: w1769 -> [w1773]
              tunnel: w1768 -> [w1772]
              tunnel: [w1774] -> w1767
              tunnel: [w1771] -> w1762
              tunnel: w1767 -> [w1779]
              tunnel: [w1779] -> w1766
              tunnel: [w1778] -> w1763
              tunnel: w1762 -> [w1778]
              tunnel: w1766 -> [w1786]
              tunnel: [w1783] -> w1765
              tunnel: [w1782] -> w1764
              tunnel: w1763 -> [w1781]
              frame #0 {
                n692 = call-poly <vilib>:"DAQmx Write.vi"("task/channels in"=w1773, "data"=FALSE, "timeout"=0.0, "error in"=w1772) -> ("task out"=w1774:refnum<k21>, "error out"=w1771:errorcluster)  [unwired: 1 in, 9 out]
                "CC stop" <- TRUE ("CC stop")
              }
              frame #1 {
                n693 = Wait (ms)(milliseconds to wait=u32 1000) -> ()  [unwired: 1 out]
              }
              frame #2 {
                n694 = call-poly <vilib>:"DAQmx Write.vi"("task/channels in"=w1786, "data"=TRUE, "timeout"=0.0, "error in"=w1781) -> ("task out"=w1783:refnum<k21>, "error out"=w1782:errorcluster)  [unwired: 1 in, 9 out]
                n695 = local write "CC stop"(FALSE ("CC stop")) -> ()
              }
            }
          }
        }
      }
      frame "Pause Check Ctrl" {
        # "still keep this constrain\nIn DLADS, scan # <= defined #"
        # "At the end of each line, this case evaluates progress and status changes (paused, etc.) and decides what to do next"
        n696 = local read "LineNumber"() -> (w1797:u32)
        n697 = local read "StripLines"() -> (w1796:u32)
        n698 = local read "Status"() -> (w1792:T11)
        n699 = Increment(x=w1797) -> (x+1=w1791:u32)
        n700 = Not Equal?(x=w1796, y=w1791) -> (x != y?=w1793:bool)
        n701 = case shown="True" w1793 {
          tunnel: w1792 -> [_ w1814]
          tunnel: [T13[] [] w1813] -> w1790
          tunnel: w1791 -> [_ w1812]
          tunnel: w1788 -> [w1808 w1811]
          tunnel: [w1807 w1810] -> w1789
          frame False {
            # "Scan finished"
            n702 = property on="Command" class="Enum (strict)"(error in=w1808, "Val(Sgnl)"=Command."Finish" ("Command")) -> (error out=w1807:errorcluster)  [unwired: 1 in, 1 out]
          }
          frame True {
            n703 = case shown="\"Working\"" w1814 {
              tunnel: [w1816 T13[] [] T13[] []] -> w1813
              tunnel: w1812 -> [w1818 _ _]
              tunnel: w1811 -> [w1817 w1832 w1836]
              tunnel: [w1817 w1831 w1835] -> w1810
              frame "Working" {
                # "LineNumber variable  only works \nfor non-DLADS mode."
                n704 = local write "LineNumber"(w1818) -> ()
                n705 = local read "BtnDLADS"() -> (w1815:bool)
                n706 = case shown="True" w1815 {
                  tunnel: [T13[] [{"Action"=enum."XY and Sensor Init", "1"=FALSE, "2"=FALSE, "3"=FALSE}, {"Action"=enum."Z Init", "1"=FALSE, "2"=FALSE, "3"=FALSE}, {"Action"=enum."MS Trig", "1"=FALSE, "2"=FALSE, "3"=FALSE}, {"Action"=enum."Line Motion", "1"=FALSE, "2"=FALSE, "3"=FALSE}, {"Action"=enum."MS Complete", "1"=FALSE, "2"=FALSE, "3"=FALSE}, {"Action"=enum."Z Exit Ctrl", "1"=FALSE, "2"=FALSE, "3"=FALSE}, {"Action"=enum."Pause Check Ctrl", "1"=FALSE, "2"=FALSE, "3"=FALSE}] w1820] -> w1816
                  frame False {
                    # "Start next line:\n\n0: XY and Sensor Init\n1: Z Init\n2: MS Trig\n3: Line Motion\n4: MS Complete\n5: Z Exit Ctrl\n6: Pause Check Ctrl"
                  }
                  frame True {
                    n707 = flat-sequence {
                      tunnel: [T13[] [{"Action"=enum."Handle DLADS", "1"=FALSE, "2"=FALSE, "3"=FALSE}]] -> w1820
                      frame #0 {
                        # "Create LOCK to trigger DLADS computation"
                        n708 = local read "sample DLADS prediction"() -> (w1821:string)
                        n709 = String To Path(string=w1821) -> (path=w1827:path)
                        n710 = Build Path(base path=w1827, name or relative path="LOCK") -> (appended path=w1825:path)
                        n711 = Open/Create/Replace File(file path (use dialog)=w1825, operation (0:open)=T21."create") -> (refnum out=w1823:refnum<file>, error out=w1822:errorcluster)  [unwired: 2 in, 3 out]
                        n712 = Close File(refnum=w1823, error in=w1822) -> ()  [unwired: 2 out]
                      }
                      frame #1 {
                        # "0: Handle DLADS"
                      }
                    }
                  }
                }
              }
              frame "Pause", Default {
                w1829 = T15."Enabled" ("Disabled")
                # "Paused: do nothing"
                n713 = property on="BtnMeasurementPause" class="Bool (strict)"(error in=w1832, "DisabledEnum"=w1829, "BoolText.Text"="Resume" ("Caption.Text")) -> (error out=w1831:errorcluster)  [unwired: 1 in, 1 out]
                n714 = property on="BtnExit" class="Bool (strict)"("DisabledEnum"=w1829) -> ()  [unwired: 2 in, 2 out]
              }
              frame "Stopping" {
                # "Finish run if stopped mid-run"
                n715 = property on="Command" class="Enum (strict)"(error in=w1836, "Val(Sgnl)"=Command."Finish" ("Value (Signaling)")) -> (error out=w1835:errorcluster)  [unwired: 1 in, 1 out]
              }
            }
          }
        }
        n716 = call "Add to Queue.vi"("error in (no error)"=w1789, "Actions"=w1790, "Queue Ref In"=w1795) -> ("error out"=w1787:errorcluster, "Queue Ref Out"=w1794:refnum<queue>)  [unwired: 7 in]
      }
      frame "Shift Data" {
        # "Shift data along x"
        n717 = local read "MotionStartTime"() -> (w1840:u32)
        n718 = call "ShiftAlongX.vi"("Data"="LineZData", "X shift"=w1840) -> ("Data"=w1839:cluster{cluster{dbl, dbl}[]}[])  [unwired: 17 in]
        n719 = local write "ZPositionPlot"(w1839) -> ()
      }
      frame "Plot Profile" {
        # "Shift data along x"
        n720 = local read "MotionStartTime"() -> (w1857:u32)
        n721 = local read "LineZData"() -> (w1858:cluster{cluster{dbl, dbl}[]}[])
        n722 = case shown="False" TRUE {
          tunnel: w1858 -> [w1869 _]
          tunnel: w1853 -> [w1868 w1913]
          tunnel: [w1867 w1913] -> w1852
          frame False {
            w1884 = u16 2 items=["coerce", "linear", "spline", "FIR filter"] ("interpolation mode")
            # "According to Hang this has never worked properly so it is commented out."
            # "Not sure what this does.\nWhat are profile array and ProfilePlot?"
            n723 = Index Array(array=w1869, index=2) -> (element=w1896:cluster{cluster{dbl, dbl}[]})
            n724 = Unbundle(w1896) -> (w1895:cluster{dbl, dbl}[])
            n725 = for {
              tunnel: w1895 -> [w1912] mode=indexing
              tunnel: [w1911] -> w1893 mode=indexing
              tunnel: [w1910] -> w1894 mode=indexing
              n726 = Unbundle(w1912) -> (w1910:dbl, w1911:dbl)
            }
            n727 = local read "Profile array"() -> (w1891:cluster{dbl[], dbl[]}[])
            n728 = Bundle(w1894, w1893) -> (w1892:cluster{dbl[], dbl[]})  [unwired: 1 in]
            n729 = Build Array (concatenate)(w1891, w1892) -> (w1874:cluster{dbl[], dbl[]}[])
            n730 = for {
              tunnel: w1874 -> [w1909] mode=indexing
              tunnel: [w1906] -> w1877 mode=indexing
              n731 = Unbundle(w1909) -> (w1908:dbl[])  [unwired: 1 out]
              n732 = Index Array(array=w1908, index=0) -> (element=w1906:dbl)
            }
            n733 = local write "Profile array"(w1874) -> ()
            n734 = Index Array(array=w1874, index=0) -> (element=w1879:cluster{dbl[], dbl[]})
            n735 = Unbundle(w1879) -> (w1889:dbl[])  [unwired: 1 out]
            n736 = Index Array(array=w1889, index #1=1 ("index"), index #2=0 ("index")) -> (element #1=w1886:dbl, element #2=w1885:dbl)
            n737 = Array Max & Min(array=w1877) -> (max index (indices)=w1876:i32)  [unwired: 3 out]
            n738 = Subtract(x=w1886, y=w1885) -> (x-y=w1883:dbl)
            n739 = Index Array(array=w1877, index=w1876) -> (element=w1875:dbl)
            n740 = call-poly <vilib>:"Resample Waveforms (single shot).vi"("Multiple XY-data in"=w1874, "dt"=w1883, "t0"=w1875, "interpolation mode"=w1884, "error in (no error)"=w1868) -> ("Multiple XY-data out"=w1881:cluster{"X-array":dbl[], "Y-array":dbl[]}[], "error out"=w1870:errorcluster)  [unwired: 6 in, 3 out]
            n741 = for {
              tunnel: w1881 -> [w1905] mode=indexing
              tunnel: [w1903] -> w1882 mode=indexing
              n742 = Unbundle(w1905) -> ("X-array"=w1904:dbl[])  [unwired: 1 out]
              n743 = Array Size(array=w1904) -> (size(s)=w1903:i32)
            }
            n744 = Array Max & Min(array=w1882) -> (min value=w1880:i32)  [unwired: 3 out]
            n745 = for {
              tunnel: w1881 -> [w1902] mode=indexing
              tunnel: w1880 -> [w1900]
              tunnel: [w1898] -> w1878 mode=indexing
              n746 = Unbundle(w1902) -> ("Y-array"=w1901:dbl[])  [unwired: 1 out]
              n747 = Array Subset(array=w1901, index=0, length=w1900) -> (w1898:dbl[])
            }
            n748 = Transpose 2D Array(2D array=w1878) -> (transposed array=w1873:dbl[][])
            "ProfilePlot" <- w1873
            n749 = Array Max & Min(array=w1873) -> (max value=w1872:dbl, min value=w1871:dbl)  [unwired: 2 out]
            n750 = property on="ProfilePlot" class="IntGraph (strict)"(error in=w1870, "ZScale.Maximum"=w1872, "ZScale.Minimum"=w1871) -> (error out=w1867:errorcluster)  [unwired: 1 in, 1 out]
          }
          frame True {
          }
        }
        n751 = call "ShiftAlongX.vi"("Data"=w1858, "X shift"=w1857) -> ("Data"=w1856:cluster{cluster{dbl, dbl}[]}[])  [unwired: 17 in]
        n752 = local write "ZPositionPlot"(w1856) -> ()
        n753 = case shown="False" "BtnSaveZToFile" {
          tunnel: w1856 -> [_ w1920]
          frame False {
          }
          frame True {
            w1928 = dbl[][] []
            # "Save data to file"
            n754 = Get Date/Time In Seconds() -> (seconds since 1Jan1904=w1939:timestamp)
            n755 = Format Date/Time String(time format string (%c)="%Y%m%d%H%M%S", seconds (now)=w1939) -> (date/time string=w1937:string)  [unwired: 1 in]
            n756 = local read "StripLineRb"() -> (w1921:u32)
            n757 = for {
              tunnel: w1920 -> [w1948] mode=indexing
              shift-right: [w1947] -> w1919
              shift-left: w1928 -> [w1946]
              shift-right: [w1942] -> w1923
              shift-left: w1928 -> [w1943]
              n758 = Unbundle(w1948) -> (w1945:cluster{dbl, dbl}[])
              n759 = for {
                tunnel: w1945 -> [w1953] mode=indexing
                tunnel: [w1952] -> w1950 mode=indexing
                tunnel: [w1951] -> w1949 mode=indexing
                n760 = Unbundle(w1953) -> (w1952:dbl, w1951:dbl)
              }
              n761 = Index Array(array=w1945, index=1) -> (element=w1941:cluster{dbl, dbl})
              n762 = Cluster To Array(cluster=w1941) -> (array=w1940:dbl[])
              n763 = Build Array (concatenate)(w1946, w1950, w1949) -> (w1947:dbl[][])
              n764 = Build Array (concatenate)(w1943, w1940) -> (w1942:dbl[][])
            }
            n765 = Format Into String(initial string=w1937, "Line" ("input 1"), w1921) -> (resulting string=w1931:string)  [unwired: 2 in, 1 out]
            n766 = Concatenate Strings(w1931, "Short.csv") -> (w1929:string)
            n767 = Concatenate Strings(w1931, ".csv") -> (w1933:string)
            n768 = String To Path(string="c:\\temp\\ZData\\") -> (path=w1932:path)
            n769 = Build Path(base path=w1932, name or relative path=w1933) -> (appended path=w1917:path)
            n770 = Build Path(base path=w1932, name or relative path=w1929) -> (appended path=w1924:path)
            n771 = call-poly <vilib>:"Write Delimited Spreadsheet.vi"("file path (dialog if empty)"=w1924, "format (%.3f)"="%.12f", "2D data"=w1923, "append to file? (new file:F)"=FALSE, "transpose? (no:F)"=TRUE, "delimiter (\\t)"="," ("delimiter (\\t)")) -> ()  [unwired: 8 in, 2 out]
            n772 = call-poly <vilib>:"Write Delimited Spreadsheet.vi"("file path (dialog if empty)"=w1917, "format (%.3f)"="%.12f", "2D data"=w1919, "append to file? (new file:F)"=FALSE, "transpose? (no:F)"=TRUE, "delimiter (\\t)"="," ("delimiter (\\t)")) -> ()  [unwired: 8 in, 2 out]
          }
        }
      }
      frame "Save Scan Config" {
        n773 = local read "BtnSaveScanConfig"() -> (w1959:bool)
        n774 = local read "BtnSaveSegLineRecords"() -> (w1957:bool)
        n775 = case shown="True" w1959 {
          tunnel: w1958 -> [w1986 w1988]
          tunnel: [w1986 w1987] -> w1956
          frame False {
          }
          frame True {
            n776 = flat-sequence {
              tunnel: w1988 -> [w2021]
              tunnel: [w2020] -> w1989
              tunnel: [w2053] -> w1987
              tunnel: w1989 -> [w2053]
              frame #0 {
                w1995 = "\n"
                w2023 = "\t"
                # "Other original inputs\n1. x stage motion type\n2. x stage start position\n3. x stage end position\n4. y stage motion type\n5. y stage start position\n6. y stage end position"
                # "4 to DLADS\n1. Number of lines\n2. Main motion range (mm)\n3. Strip motion range (mm)\n4. Scan rate (mm/s)"
                # "save it into .txt"
                # "info, tab-delimited format, hardcode all entries"
                # "Path, predifined"
                n777 = local read "XStartPosition"() -> (w1993:dbl)
                n778 = local read "XEndPosition"() -> (w1992:dbl)
                n779 = local read "YStartPosition"() -> (w1991:dbl)
                n780 = local read "YEndPosition"() -> (w1990:dbl)
                n781 = Subtract(x=w1992, y=w1993) -> (x-y=w2015:dbl)
                n782 = Subtract(x=w1990, y=w1991) -> (x-y=w2012:dbl)
                n783 = local read "XStageType"() -> (w2017:enum16{"Main motion", "Strip motion"})
                n784 = Format Into String(format string="%.4f", w2015) -> (resulting string=w2010:string)  [unwired: 2 in, 1 out]
                n785 = Format Into String(format string="%.4f", w2012) -> (resulting string=w2011:string)  [unwired: 2 in, 1 out]
                n786 = Format Into String(format string="%.4f", w1990) -> (resulting string=w1996:string)  [unwired: 2 in, 1 out]
                n787 = local read "Velocity"() -> (w2006:dbl)
                n788 = Format Into String(format string="%.4f", w1991) -> (resulting string=w1997:string)  [unwired: 2 in, 1 out]
                n789 = Get Date/Time In Seconds() -> (seconds since 1Jan1904=w2047:timestamp)
                n790 = case shown="\"Strip motion\"" w2017 {
                  tunnel: w2011 -> [w2048 w2050]
                  tunnel: w2010 -> [w2049 w2051]
                  tunnel: [w2049 w2050] -> w2009
                  tunnel: [w2048 w2051] -> w2008
                  frame "Main motion", Default {
                  }
                  frame "Strip motion" {
                  }
                }
                n791 = Format Into String(format string="%.4f", w2006) -> (resulting string=w1994:string)  [unwired: 2 in, 1 out]
                n792 = Format Into String(format string="%.4f", w1992) -> (resulting string=w2002:string)  [unwired: 2 in, 1 out]
                n793 = Format Date/Time String(time format string (%c)="%Y%m%d%H%M%S", seconds (now)=w2047) -> (date/time string=w2041:string)  [unwired: 1 in]
                n794 = Format Into String(w2017) -> (resulting string=w2016:string)  [unwired: 3 in, 1 out]
                n795 = Format Into String(format string="%.4f", w1993) -> (resulting string=w2004:string)  [unwired: 2 in, 1 out]
                n796 = local read "StripLines"() -> (w2019:u32)
                n797 = local read "YStageType"() -> (w2001:enum16{"Main motion", "Strip motion"})
                n798 = Concatenate Strings(w2041, ".txt") -> (w2043:string)
                n799 = String To Path(string="c:\\temp\\scan_config\\") -> (path=w2042:path)
                n800 = Format Into String(w2019) -> (resulting string=w2018:string)  [unwired: 3 in, 1 out]
                n801 = Format Into String(w2001) -> (resulting string=w2000:string)  [unwired: 3 in, 1 out]
                n802 = Build Path(base path=w2042, name or relative path=w2043) -> (appended path=w2040:path)
                n803 = Open/Create/Replace File(file path (use dialog)=w2040, error in=w2021, operation (0:open)=T21."create", access (0:read/write)=enum16{"read/write", "read-only", "write-only"}."write-only") -> (refnum out=w2037:refnum<file>, error out=w2036:errorcluster)  [unwired: 3 out]
                n804 = Concatenate Strings("Number of lines:", w2023, w2018, w1995, "Main motion range (mm):", w2023, w2009, w1995, "Strip motion range (mm):", w2023, w2008, w1995, "Scan rate (mm/s):", w2023, w1994, w1995, "x stage motion type:", w2023, w2016, w1995, "x stage start position (mm):", w2023, w2004, w1995, "x stage end position (mm):", w2023, w2002, w1995, "y stage motion type:", w2023, w2000, w1995, "y stage start position (mm):", w2023, w1997, w1995, "y stage end position (mm):", w2023, w1996) -> (w2022:string)
                n805 = Write to Text File(file (use dialog)=w2037, text=w2022, error in=w2036) -> (refnum out=w2035:refnum<file>, error out=w2034:errorcluster)  [unwired: 1 in, 1 out]
                n806 = Close File(refnum=w2035, error in=w2034) -> (error out=w2020:errorcluster)  [unwired: 1 out]
              }
              frame #1 {
                n807 = local write "BtnSaveScanConfig"(FALSE ("BtnSaveScanConfig")) -> ()
              }
            }
          }
        }
        n808 = case shown="True" w1957 {
          tunnel: w1958 -> [w1969 w1972]
          tunnel: [w1969 w1970] -> w1954
          frame False {
          }
          frame True {
            n809 = flat-sequence {
              tunnel: w1972 -> [w1974]
              tunnel: [w1973] -> w1971
              tunnel: w1971 -> [w1984]
              tunnel: [w1984] -> w1970
              frame #0 {
                # "Path, predifined"
                n810 = Get Date/Time In Seconds() -> (seconds since 1Jan1904=w1983:timestamp)
                n811 = Format Date/Time String(time format string (%c)="%Y%m%d%H%M%S", seconds (now)=w1983) -> (date/time string=w1977:string)  [unwired: 1 in]
                n812 = Concatenate Strings(w1977, ".txt") -> (w1979:string)
                n813 = String To Path(string="c:\\temp\\segLine_record\\") -> (path=w1978:path)
                n814 = Build Path(base path=w1978, name or relative path=w1979) -> (appended path=w1976:path)
                n815 = local read "segLines"() -> (w1975:dbl[][])
                n816 = call-poly <vilib>:"Write Delimited Spreadsheet.vi"("file path (dialog if empty)"=w1976, "2D data"=w1975, "error in (no error)"=w1974) -> ("error out"=w1973:errorcluster)  [unwired: 11 in, 1 out]
              }
              frame #1 {
                n817 = local write "BtnSaveSegLineRecords"(FALSE ("BtnSaveSegLineRecords")) -> ()
              }
            }
          }
        }
        n818 = Merge Errors(w1956, w1954) -> (w1955:errorcluster)
      }
      frame "Save Profile Text File" {
        n819 = Open/Create/Replace File(error in=w2055, prompt="Save", operation (0:open)=T21."replace or create", access (0:read/write)=enum16{"read/write", "read-only", "write-only"}."write-only") -> (refnum out=w2058:refnum<file>, cancelled=w2059:bool, error out=w2057:errorcluster)  [unwired: 2 in]
        n820 = case shown="True" w2059 {
          tunnel: w2058 -> [w2074 _]
          tunnel: w2057 -> [w2073 w2134]
          tunnel: [w2071 w2134] -> w2054
          frame False {
            w2093 = u16 2 items=["coerce", "linear", "spline", "FIR filter"] ("interpolation mode")
            # "Write Profile array to text file"
            n821 = local read "Profile array"() -> (w2072:cluster{dbl[], dbl[]}[])
            n822 = for {
              tunnel: w2072 -> [w2133] mode=indexing
              tunnel: [w2131] -> w2082 mode=indexing
              n823 = Unbundle(w2133) -> (w2130:dbl[])  [unwired: 1 out]
              n824 = Index Array(array=w2130, index=0) -> (element=w2131:dbl)
            }
            n825 = Index Array(array=w2072, index=0) -> (element=w2099:cluster{dbl[], dbl[]})
            n826 = Unbundle(w2099) -> (w2097:dbl[])  [unwired: 1 out]
            n827 = Array Max & Min(array=w2082) -> (max index (indices)=w2081:i32)  [unwired: 3 out]
            n828 = Index Array(array=w2097, index #1=1 ("index"), index #2=0 ("index")) -> (element #1=w2094:dbl, element #2=w2076:dbl)
            n829 = Index Array(array=w2082, index=w2081) -> (element=w2080:dbl)
            n830 = Subtract(x=w2094, y=w2076) -> (x-y=w2087:dbl)
            n831 = call-poly <vilib>:"Resample Waveforms (single shot).vi"("Multiple XY-data in"=w2072, "dt"=w2087, "t0"=w2080, "interpolation mode"=w2093, "error in (no error)"=w2073) -> ("Multiple XY-data out"=w2091:cluster{"X-array":dbl[], "Y-array":dbl[]}[], "error out"=w2090:errorcluster)  [unwired: 6 in, 3 out]
            n832 = Divide(x=w2087, y=1000.0) -> (x/y=w2086:dbl)
            n833 = for {
              tunnel: w2091 -> [w2129] mode=indexing
              tunnel: [w2127] -> w2092 mode=indexing
              n834 = Unbundle(w2129) -> ("X-array"=w2128:dbl[])  [unwired: 1 out]
              n835 = Array Size(array=w2128) -> (size(s)=w2127:i32)
            }
            n836 = Array Max & Min(array=w2092) -> (min value=w2089:i32)  [unwired: 3 out]
            n837 = for {
              N: w2089 -> [_]
              shift-right: [w2107] -> w2078
              shift-left: "" -> [w2106]
              tunnel: w2086 -> [w2104]
              i -> [w2105]
              n838 = Multiply(x=w2104, y=w2105) -> (x*y=w2102:dbl)
              n839 = Number To Fractional String(number=w2102, precision (6)=i16 3) -> (F-format string=w2100:string)  [unwired: 2 in]
              n840 = Concatenate Strings(w2106, "," ("string"), w2100) -> (w2107:string)
            }
            n841 = Concatenate Strings(w2078, "\r\n") -> (w2077:string)
            n842 = Write to Text File(file (use dialog)=w2074, text=w2077, error in=w2090) -> (refnum out=w2075:refnum<file>, error out=w2084:errorcluster)  [unwired: 1 in, 1 out]
            n843 = for {
              tunnel: w2091 -> [w2120] mode=indexing
              tunnel: w2089 -> [w2118]
              shift-right: [w2115] -> w2083
              shift-left: w2084 -> [w2116]
              tunnel: w2075 -> [w2111]
              i -> [w2113]
              n844 = Unbundle(w2120) -> ("Y-array"=w2119:dbl[])  [unwired: 1 out]
              n845 = Array Subset(array=w2119, index=0, length=w2118) -> (w2114:dbl[])
              n846 = Number To Decimal String(number=w2113) -> (decimal integer string=w2112:string)  [unwired: 1 in]
              n847 = for {
                shift-right: [w2126] -> w2108
                shift-left: w2112 -> [w2125]
                tunnel: w2114 -> [w2121] mode=indexing
                n848 = Number To Fractional String(number=w2121, precision (6)=i16 2) -> (F-format string=w2122:string)  [unwired: 2 in]
                n849 = Concatenate Strings(w2125, "," ("string"), w2122) -> (w2126:string)
              }
              n850 = Concatenate Strings(w2108, "\r\n") -> (w2109:string)
              n851 = Write to Text File(file (use dialog)=w2111, text=w2109, error in=w2116) -> (error out=w2115:errorcluster)  [unwired: 1 in, 2 out]
            }
            n852 = Close File(refnum=w2075, error in=w2083) -> (error out=w2071:errorcluster)  [unwired: 1 out]
          }
          frame True {
          }
        }
      }
      frame "Get Time" {
        n853 = Get Date/Time In Seconds() -> (seconds since 1Jan1904=→"Current Time":timestamp)
      }
      frame "HW Close - Zaber" {
        w2150 = T1 {"Serial port handle"="", "Axis"="", "Controller #"=0, "Min position"=0.0, "Max position"=0.0, "Min velocity"=0.0, "Max velocity"=0.0, "Firmware"="", "Device ID"=0, "Variable event"=refnum, "Variable ref"=refnum, "Resolution, usteps/step"=0, "Serial port semaphore"=refnum, "Joystick buttons"={"MinDir"=1, "MaxDir"=2, "MedSpeed"=5, "HighSpeed"=6}} ("Zaber out")
        n854 = call "UnJoin.vi"("Zaber"=w2155, "error in"=w2147) -> ("error out"=w2153:errorcluster)  [unwired: 17 in]
        n855 = call "Disconnect.vi"("Zaber"=w2156, "error in"=w2147) -> ("error out"=w2152:errorcluster)  [unwired: 17 in]
        n856 = call "Disconnect.vi"("Zaber"=w2154, "error in"=w2147) -> ("error out"=w2151:errorcluster)  [unwired: 17 in]
        n857 = Merge Errors(w2153, w2152, w2151) -> (w2146:errorcluster)
      }
      frame "HW Close - DO" {
        w2164 = refnum<k21> refnum ("task out")
        n858 = call <vilib>:"DAQmx Clear Task.vi"("task in"=w2166, "error in"=w2162) -> ("error out"=w2167:errorcluster)  [unwired: 13 in]
        n859 = call <vilib>:"DAQmx Clear Task.vi"("task in"=w2165, "error in"=w2167) -> ("error out"=w2161:errorcluster)  [unwired: 13 in]
      }
      frame "Shutdown Ctrl" {
        # "0: Exit\n1: HW Close - Zaber\n2: HW Close - DO"
        # "Generate \"quit\" event"
        # "Close Run.vi"
        # "Close Dialog3Stages.vi"
        n860 = local read "Method"() -> (w2182:T9)
        n861 = case shown="\"Shear force sensor\"" w2182 {
          tunnel: [T13 {"Action"=enum."Method close - Keyence", "1"=FALSE, "2"=FALSE, "3"=FALSE} ("element") T13 {"Action"=enum."Method close - SICM", "1"=FALSE, "2"=FALSE, "3"=FALSE} ("element") T13 {"Action"=enum."Method close - Shear force", "1"=FALSE, "2"=FALSE, "3"=FALSE} ("element") T13 {"Action"=enum."Wait (ms)", "1"=FALSE, "2"=FALSE, "3"=FALSE} ("element")] -> w2180
          frame "Keyence sensor" {
          }
          frame "SICM sensor" {
          }
          frame "Shear force sensor" {
          }
          frame Default {
          }
        }
        n862 = Build Array (concatenate)(T13[] [{"Action"=enum."Exit", "1"=FALSE, "2"=FALSE, "3"=FALSE}, {"Action"=enum."HW Close - Zaber", "1"=FALSE, "2"=FALSE, "3"=FALSE}, {"Action"=enum."HW Close - DO", "1"=FALSE, "2"=FALSE, "3"=FALSE}], w2180) -> (w2179:T13[])
        n863 = call "Enqueue At Front.vi"("elements"=w2179, "error in"=w2177, "queue in"=w2178) -> ("error out"=w2175:errorcluster, "queue out"=w2176:refnum<queue>)  [unwired: 7 in]
        n864 = Generate User Event(user event=w2184, event data cluster=TRUE ("event data"), error in=w2175) -> (user event out=w2183:refnum<user-event>, error out=w2185:errorcluster)  [unwired: 1 in]
        n865 = local read "Call type"() -> (w2203:enum16{"Dynamic", "Static"})
        n866 = case shown="\"Static\", Default" w2203 {
          tunnel: w2185 -> [w2215 w2217]
          tunnel: [w2215 w2216] -> w2189
          frame "Static", Default {
          }
          frame "Dynamic" {
            # "Close reference to\nTip tune ZaberAndSR865.vi"
            n867 = local read "Tune ShFrc"() -> (w2219:refnum<vi>)
            n868 = local read "Stop tune ShFrc"() -> (w2220:refnum<user-event>)
            n869 = Close Reference(reference=w2219, error in (no error)=w2217) -> (error out=w2218:errorcluster)
            n870 = Destroy User Event(user event=w2220, error in=w2218) -> (error out=w2216:errorcluster)
          }
        }
        n871 = local read "RunRef"() -> (w2188:refnum<vi>)
        n872 = call-by-ref "Wait On Asynchronous Call"(reference=w2188, error in=w2189) -> (reference out=w2198:refnum<vi>, error out=w2200:errorcluster, 19:"error out"=w2199:errorcluster)  [unwired: 18 in, 1 out]
        n873 = Merge Errors(w2200, w2199) -> (w2202:errorcluster)
        n874 = invoke class="VI Interface Type 0" method="FP.Close"(reference=w2198, error in=w2202) -> (reference out=w2197:refnum<vi>, error out=w2201:errorcluster)  [unwired: 1 in, 1 out]
        n875 = local read "Dialog3StagesRef"() -> (w2187:refnum<vi>)
        n876 = Close Reference(reference=w2197, error in (no error)=w2201) -> (error out=w2190:errorcluster)
        n877 = call-by-ref "Wait On Asynchronous Call"(reference=w2187, error in=w2190) -> (reference out=w2194:refnum<vi>, error out=w2195:errorcluster, 19:"error out"=w2196:errorcluster)  [unwired: 19 in]
        n878 = Merge Errors(w2195, w2196) -> (w2193:errorcluster)
        n879 = invoke class="VI Interface Type 1" method="FP.Close"(reference=w2194, error in=w2193) -> (reference out=w2192:refnum<vi>, error out=w2191:errorcluster)  [unwired: 1 in, 1 out]
        n880 = Close Reference(reference=w2192, error in (no error)=w2191) -> (error out=w2174:errorcluster)
      }
      frame "Exit" {
        w2231 = TRUE
        # "Stop instrument loop"
        # "Generates a \"Done Event\" user event \nthat stops the user interface loop"
        n881 = Generate User Event(user event=w2233, event data cluster=w2231, error in=w2222) -> (user event out=w2223:refnum<user-event>, error out=w2221:errorcluster)  [unwired: 1 in]
      }
      frame "Error" {
        # "Clear errors"
        # "Once an error has been detected, the error must be processed.  Often the error code can be used to select execution of a case to resolve the issue and continue normal operation."
        n882 = Unbundle By Name(w2235) -> ("code"=w2248:i32)
        n883 = case shown="1055" w2248 {
          selector: w2248 -> [w2249 _ _ _ _ _]
          tunnel: [T13 {"Action"=enum."Exit", "1"=FALSE, "2"=FALSE, "3"=FALSE} ("Exec State") T13 {"Action"=enum."Get Time", "1"=FALSE, "2"=FALSE, "3"=FALSE} ("Exec State") T13 {"Action"=enum."Wait (ms)", "1"=FALSE, "2"=FALSE, "3"=FALSE} ("Exec State") T13 {"Action"=enum."Wait (ms)", "1"=FALSE, "2"=FALSE, "3"=FALSE} ("Exec State") T13 {"Action"=enum."Wait (ms)", "1"=FALSE, "2"=FALSE, "3"=FALSE} ("Exec State") T13 {"Action"=enum."Wait (ms)", "1"=FALSE, "2"=FALSE, "3"=FALSE} ("Exec State")] -> w2247
          frame Default {
            # "Unknown Error\nExit Program"
            n884 = call <vilib>:"General Error Handler.vi"("[error code] (0)"=w2249) -> ()  [unwired: 10 in, 5 out]
          }
          frame 43 {
            # "Known Error\nJust wait for\nit to clear"
          }
          frame -2000000006 {
            n885 = One Button Dialog(message="Error -2000000006:\nJoystick not connected.") -> ()  [unwired: 1 in, 1 out]
          }
          frame -1073807343 {
            n886 = property on="Com error" class="Bool (strict)"("Value"=TRUE ("Com error")) -> (error out=w2254:errorcluster)  [unwired: 2 in, 1 out]
            n887 = One Button Dialog(message="Error -1073807343:\nLock-in amplifier not connected.") -> ()  [unwired: 1 in, 1 out]
            n888 = property on="Method" class="Enum (strict)"(error in=w2254, "Val(Sgnl)"=T9."Simple plane" ("Value (Signaling)")) -> ()  [unwired: 1 in, 2 out]
          }
          frame 1055 {
            n889 = property on="Com error" class="Bool (strict)"("Value"=TRUE ("Com error")) -> (error out=w2260:errorcluster)  [unwired: 2 in, 1 out]
            n890 = One Button Dialog(message="Error 1055:\nKeyence not connected.") -> ()  [unwired: 1 in, 1 out]
            n891 = property on="Method" class="Enum (strict)"(error in=w2260, "Val(Sgnl)"=T9."Simple plane" ("Value (Signaling)")) -> ()  [unwired: 1 in, 2 out]
          }
          frame -1073807346 {
            n892 = property on="Com error" class="Bool (strict)"("Value"=TRUE ("Com error")) -> (error out=w2265:errorcluster)  [unwired: 2 in, 1 out]
            n893 = One Button Dialog(message="Error -1073807346:\nSICM sensor not connected.") -> ()  [unwired: 1 in, 1 out]
            n894 = property on="Method" class="Enum (strict)"(error in=w2265, "Val(Sgnl)"=T9."Simple plane" ("Value (Signaling)")) -> ()  [unwired: 1 in, 2 out]
          }
        }
        n895 = Enqueue Element At Opposite End(queue=w2238, element=w2247, error in (no error)=errorcluster {"status"=FALSE, "code"=0, "source"=""}) -> (queue out=w2244:refnum<queue>, error out=w2236:errorcluster)  [unwired: 1 in, 1 out]
      }
      frame "Wait (ms)" {
        n896 = Wait (ms)(milliseconds to wait=u32 100) -> ()  [unwired: 1 out]
      }
    }
  }
  n897 = while {
    tunnel: w21 -> [w2287]
    tunnel: [w2286] -> w19
    tunnel: w18 -> [w2285]
    shift-right: [w2280] -> w1
    shift-left: w4 -> [w2281]
    stop <- w2283 stop-if-true
    n898 = event shown="[9] \"BtnPlaneSetPoint1\": Value Change" {
      selector: w2287 -> [_ _ _ _ _ _ _ _ _ _ _ _ _ _ _ _ _]
      dyn-events: [_ _ _ _ _ _ _ _ _ _ _ _ _ _ _ _ _] -> w2286
      timeout: _ -> [_ _ _ _ _ _ _ _ _ _ _ _ _ _ _ _ _]
      tunnel: [TRUE _ _ _ _ _ _ _ _ _ _ _ _ _ _ _ _] -> w2283
      tunnel: [_ w2301 w2313 T13[] [{"Action"=enum."Set Motion Params", "1"=FALSE, "2"=FALSE, "3"=FALSE}] w2324 w2330 w2336 w2343 _ w2365 w2372 w2377 T13[] [] T13[] [] w2399 T13[] [{"Action"=enum."Save Profile Text File", "1"=FALSE, "2"=FALSE, "3"=FALSE}] T13[] [{"Action"=enum."Save Scan Config", "1"=FALSE, "2"=FALSE, "3"=FALSE}]] -> w2284
      tunnel: [_ TRUE TRUE _ _ _ _ _ _ _ _ _ _ _ w2398 _ _] -> w2282
      tunnel: w2281 -> [w2296 w2298 w2310 w2321 w2323 w2329 w2335 w2342 w2357 w2364 w2370 w2376 w2382 w2390 w2400 w2418 w2422]
      tunnel: [w2296 w2298 w2310 w2321 w2323 w2329 w2335 w2342 w2356 w2364 w2370 w2376 w2382 w2390 w2400 w2418 w2422] -> w2280
      event User Event {
        # "Stop user interface loop"
        n899 = event-data() -> ()  [unwired: 1 in, 5 out]
      }
      event "BtnExit": Value Change {
        # "0: Shutdown Ctrl"
        # "0: Wait"
        # "Prompt user before quitting"
        n900 = event-data() -> ()  [unwired: 1 in, 6 out]
        n901 = local read "Status"() -> (w2299:T11)
        n902 = Two Button Dialog(message="Are you sure you want to quit?", 1:"Quit" ("T button name (\"OK\")"), 2:"Return" ("F button name (\"Cancel\")")) -> (T button?=w2304:bool)
        n903 = case shown="\"Idle\", Default" w2299 {
          frame "Idle", Default {
          }
          frame "Working" {
            n904 = local write "Status"(Status."Stopping" ("Status")) -> ()
          }
        }
        n905 = Select(t=T13[] [{"Action"=enum."Wait (ms)", "1"=FALSE, "2"=FALSE, "3"=FALSE}], s=w2304, f=T13[] [{"Action"=enum."Shutdown Ctrl", "1"=FALSE, "2"=FALSE, "3"=FALSE}]) -> (s? t:f=w2301:T13[])
      }
      event Panel Close? {
        # "0: Shutdown Ctrl"
        # "0: Wait"
        # "Prompt user before quitting"
        n906 = event-data() -> ()  [unwired: 1 in, 4 out]
        n907 = Two Button Dialog(message="Are you sure you want to quit?", 1:"Quit" ("T button name (\"OK\")"), 2:"Return" ("F button name (\"Cancel\")")) -> (T button?=w2317:bool)
        n908 = local read "Status"() -> (w2311:T11)
        n909 = case shown="\"Working\"" w2311 {
          frame "Idle", Default {
          }
          frame "Working" {
            n910 = local write "Status"(Status."Stopping" ("Status")) -> ()
          }
        }
        n911 = Select(t=T13[] [{"Action"=enum."Wait (ms)", "1"=FALSE, "2"=FALSE, "3"=FALSE}], s=w2317, f=T13[] [{"Action"=enum."Shutdown Ctrl", "1"=FALSE, "2"=FALSE, "3"=FALSE}]) -> (s? t:f=w2313:T13[])
        n912 = event-data("Discard?"=TRUE) -> ()  [unwired: 1 in, 1 out]
      }
      event "ZStartPosition", "SPZEndPosition", "ZStep", "XStageType", "XStartPosition", "XEndPosition", "Velocity", "StripLines", "YStartPosition", "YEndPosition": Value Change {
        # "0: Set Motion Params"
        n913 = event-data() -> ()  [unwired: 1 in, 6 out]
      }
      event "BtnSetZOutPosition": Value Change {
        n914 = event-data() -> ("NewVal"=w2325:bool)  [unwired: 1 in, 5 out]
        n915 = case shown="True" w2325 {
          tunnel: [T13[] [] T13[] [{"Action"=enum."Set Zout Pos", "1"=FALSE, "2"=FALSE, "3"=FALSE}]] -> w2324
          frame False {
          }
          frame True {
            # "0: Set Zout Pos"
            n916 = local write "BtnSetZOutPosition"(FALSE ("BtnSetZOutPosition")) -> ()
          }
        }
      }
      event "BtnSetZStartPosition": Value Change {
        n917 = event-data() -> ("NewVal"=w2331:bool)  [unwired: 1 in, 5 out]
        n918 = case shown="True" w2331 {
          tunnel: [T13[] [] T13[] [{"Action"=enum."Set Zstart Pos", "1"=FALSE, "2"=FALSE, "3"=FALSE}, {"Action"=enum."Set Motion Params", "1"=FALSE, "2"=FALSE, "3"=FALSE}]] -> w2330
          frame False {
          }
          frame True {
            # "0: Set Zstart Pos\n1: Set Motion Params"
            n919 = local write "BtnSetZStartPosition"(FALSE ("BtnSetZOutPosition")) -> ()
          }
        }
      }
      event "BtnZ-", "BtnZ+": Value Change {
        n920 = event-data() -> ("NewVal"=w2337:bool)  [unwired: 1 in, 5 out]
        n921 = case shown="True" w2337 {
          tunnel: [T13[] [] T13[] [{"Action"=enum."Step Z", "1"=FALSE, "2"=FALSE, "3"=FALSE}]] -> w2336
          frame False {
          }
          frame True {
            # "0: Step Z"
            n922 = local write "BtnZ-"(FALSE ("BtnZ-")) -> ()
          }
        }
      }
      event "Method": Value Change {
        n923 = event-data() -> ("OldVal"=w2346:T9)  [unwired: 1 in, 5 out]
        n924 = case shown="True" "Com error" {
          tunnel: w2346 -> [w2348 _]
          tunnel: [w2347 T13 {"Action"=enum."Wait (ms)", "1"=FALSE, "2"=FALSE, "3"=FALSE} ("Exec State")] -> w2345
          frame False {
            n925 = case shown="Default" w2348 {
              tunnel: [T13 {"Action"=enum."Method close - SICM", "1"=FALSE, "2"=FALSE, "3"=FALSE} ("Exec State") T13 {"Action"=enum."Wait (ms)", "1"=FALSE, "2"=FALSE, "3"=FALSE} ("Exec State") T13 {"Action"=enum."Method close - Keyence", "1"=FALSE, "2"=FALSE, "3"=FALSE} ("Exec State") T13 {"Action"=enum."Method close - Shear force", "1"=FALSE, "2"=FALSE, "3"=FALSE} ("Exec State")] -> w2347
              frame "SICM sensor" {
              }
              frame Default {
              }
              frame "Keyence sensor" {
              }
              frame "Shear force sensor" {
              }
            }
          }
          frame True {
            # "Do not close hardware if there was an \nerror establishing communication"
            n926 = local write "Com error"(FALSE ("Com error")) -> ()
          }
        }
        n927 = Build Array(w2345, T13 {"Action"=enum."Method UI and HW init", "1"=FALSE, "2"=FALSE, "3"=FALSE} ("element")) -> (w2343:T13[])
      }
      event "BtnShearForceTune": Value Change {
        n928 = event-data() -> ()  [unwired: 1 in, 6 out]
        n929 = local read "Call type"() -> (w2358:enum16{"Dynamic", "Static"})
        n930 = local read "Z Zaber"() -> (w2355:T1)
        n931 = case shown="\"Static\"" w2358 {
          tunnel: w2355 -> [w2361 _]
          tunnel: w2357 -> [w2360 w2363]
          tunnel: [w2359 w2363] -> w2356
          frame "Static" {
            n932 = local read "SR865"() -> (w2362:T6)
            n933 = call "Tip tune ZaberAndSR865 Static.vi"("Z axis"=w2361, "SR865"=w2362, "error in"=w2360) -> ("error out"=w2359:errorcluster)  [unwired: 16 in]
          }
          frame "Dynamic", Default {
          }
        }
      }
      event "BtnPlaneSetPoint1": Value Change {
        n934 = event-data() -> ("NewVal"=w2366:bool)  [unwired: 1 in, 5 out]
        n935 = case shown="True" w2366 {
          tunnel: [T13[] [] T13[] [{"Action"=enum."Plane Set Point 1", "1"=FALSE, "2"=FALSE, "3"=FALSE}, {"Action"=enum."Calculate Plane", "1"=FALSE, "2"=FALSE, "3"=FALSE}, {"Action"=enum."Set Motion Params", "1"=FALSE, "2"=FALSE, "3"=FALSE}]] -> w2365
          frame False {
          }
          frame True {
            # "0: Plate Set Point 1\n1: Calculate Plane\n2: Set Motion Params"
            n936 = local write "BtnPlaneSetPoint1"(FALSE ("BtnPlaneSetPoint1")) -> ()
          }
        }
      }
      event "BtnPlaneSetPoint2": Value Change {
        n937 = event-data() -> ("NewVal"=w2371:bool)  [unwired: 1 in, 5 out]
        n938 = case shown="True" w2371 {
          tunnel: [T13[] [] T13[] [{"Action"=enum."Plane Set Point 2", "1"=FALSE, "2"=FALSE, "3"=FALSE}, {"Action"=enum."Calculate Plane", "1"=FALSE, "2"=FALSE, "3"=FALSE}, {"Action"=enum."Set Motion Params", "1"=FALSE, "2"=FALSE, "3"=FALSE}]] -> w2372
          frame False {
          }
          frame True {
            # "0: Plate Set Point 2\n1: Calculate Plane\n2: Set Motion Params"
            n939 = local write "BtnPlaneSetPoint2"(FALSE ("BtnPlaneSetPoint1")) -> ()
          }
        }
      }
      event "BtnPlaneSetPoint3": Value Change {
        n940 = event-data() -> ("NewVal"=w2378:bool)  [unwired: 1 in, 5 out]
        n941 = case shown="True" w2378 {
          tunnel: [T13[] [] T13[] [{"Action"=enum."Plane Set Point 3", "1"=FALSE, "2"=FALSE, "3"=FALSE}, {"Action"=enum."Calculate Plane", "1"=FALSE, "2"=FALSE, "3"=FALSE}, {"Action"=enum."Set Motion Params", "1"=FALSE, "2"=FALSE, "3"=FALSE}]] -> w2377
          frame False {
          }
          frame True {
            # "0: Plate Set Point 3\n1: Calculate Plane\n2: Set Motion Params"
            n942 = local write "BtnPlaneSetPoint3"(FALSE ("BtnPlaneSetPoint1")) -> ()
          }
        }
      }
      event "BtnMeasurement": Value Change {
        n943 = event-data() -> ("NewVal"=w2385:bool)  [unwired: 1 in, 5 out]
        n944 = local read "Status"() -> (w2384:T11)
        n945 = case shown="True" w2385 {
          tunnel: w2384 -> [w2386 w2388]
          frame False {
            n946 = case shown="\"Working\"" w2386 {
              frame Default {
              }
              frame "Working" {
                n947 = property on="Command" class="Enum (strict)"("Val(Sgnl)"=Command."Stop" ("Value (Signaling)")) -> ()  [unwired: 2 in, 2 out]
              }
            }
          }
          frame True {
            n948 = case shown="\"Idle\"" w2388 {
              frame "Idle" {
                n949 = property on="Command" class="Enum (strict)"("Val(Sgnl)"=Command."Start" ("Value (Signaling)")) -> ()  [unwired: 2 in, 2 out]
              }
              frame Default {
              }
            }
          }
        }
      }
      event "BtnMeasurementPause": Value Change {
        n950 = event-data() -> ("NewVal"=w2393:bool)  [unwired: 1 in, 5 out]
        n951 = local read "Status"() -> (w2392:T11)
        n952 = case shown="True" w2393 {
          tunnel: w2392 -> [w2394 w2396]
          frame False {
            n953 = case shown="\"Pause\"" w2394 {
              frame Default {
              }
              frame "Pause" {
                n954 = property on="Command" class="Enum (strict)"("Val(Sgnl)"=Command."Resume" ("Value (Signaling)")) -> ()  [unwired: 2 in, 2 out]
              }
            }
          }
          frame True {
            n955 = case shown="\"Working\"" w2396 {
              frame Default {
              }
              frame "Working" {
                n956 = property on="Command" class="Enum (strict)"("Val(Sgnl)"=Command."Suspend" ("Value (Signaling)")) -> ()  [unwired: 2 in, 2 out]
              }
            }
          }
        }
      }
      event Value Change {
        # "0: Scan Ctrl\n1: Scan UI"
        n957 = event-data() -> ("NewVal"=w2402:T10)  [unwired: 1 in, 5 out]
        n958 = case shown="\"Stop\"" w2402 {
          tunnel: [Status."Working" ("Status") Status."Working" ("y") Status."Stopping" ("Status") Status."Idle" ("Status") Status."Pause" ("y")] -> w2401
          tunnel: [T13[] [{"Action"=enum."Scan UI", "1"=FALSE, "2"=FALSE, "3"=FALSE}, {"Action"=enum."Scan Ctrl", "1"=FALSE, "2"=FALSE, "3"=FALSE}] T13[] [{"Action"=enum."Scan UI", "1"=FALSE, "2"=FALSE, "3"=FALSE}, {"Action"=enum."Pause Check Ctrl", "1"=FALSE, "2"=FALSE, "3"=FALSE}] T13[] [{"Action"=enum."Scan UI", "1"=FALSE, "2"=FALSE, "3"=FALSE}] T13[] [{"Action"=enum."Scan UI", "1"=FALSE, "2"=FALSE, "3"=FALSE}] T13[] [{"Action"=enum."Scan UI", "1"=FALSE, "2"=FALSE, "3"=FALSE}]] -> w2399
          tunnel: [FALSE FALSE TRUE FALSE TRUE] -> w2398
          frame "Start" {
            # "0: Scan UI\n1: Scan Ctrl"
          }
          frame "Resume" {
            # "0: Scan UI\n1: Pause Check Ctrl"
          }
          frame "Stop" {
            # "0: Scan UI"
          }
          frame "Finish", Default {
            # "0: Scan UI"
          }
          frame "Suspend" {
            # "0: Scan UI"
          }
        }
        n959 = local write "Status"(w2401) -> ()
      }
      event "BtnSave": Value Change {
        # "0: Save Text File"
        n960 = event-data() -> ()  [unwired: 1 in, 6 out]
        n961 = local write "BtnSave"(FALSE ("BtnSave")) -> ()
      }
      event "BtnSaveScanConfig", "BtnSaveSegLineRecords": Value Change {
        # "multiple saves use the same state"
        n962 = event-data() -> ()  [unwired: 1 in, 6 out]
      }
    }
    n963 = case shown="False" w2282 {
      tunnel: w2285 -> [w2288 w2293]
      tunnel: w2284 -> [w2289 w2292]
      frame False {
        # "Enqueue at back"
        n964 = for {
          tunnel: w2289 -> [w2291] mode=indexing
          tunnel: w2288 -> [w2290]
          n965 = Enqueue Element(queue=w2290, element=w2291) -> ()  [unwired: 2 in, 3 out]
        }
      }
      frame True {
        # "Enqueue at front"
        n966 = for {
          tunnel: w2292 -> [w2295] mode=indexing
          tunnel: w2293 -> [w2294]
          n967 = Enqueue Element At Opposite End(queue=w2294, element=w2295) -> ()  [unwired: 2 in, 3 out]
        }
      }
    }
  }
  n968 = Unregister For Events(event registration refnum=w19) -> ()  [unwired: 1 in, 1 out]
  n969 = Merge Errors(w1, w3) -> (w2:errorcluster)
  n970 = Flush Queue(queue=w14, error in (no error)=w2) -> (queue out=w16:refnum<queue>, error out=w15:errorcluster)  [unwired: 1 out]
  n971 = Release Queue(queue=w16, error in (no error)=w15) -> (error out=w8:errorcluster)  [unwired: 1 in, 2 out]
  n972 = Destroy User Event(user event=w10, error in=w8) -> (error out=w11:errorcluster)
  n973 = Destroy User Event(user event=w20, error in=w11) -> ()  [unwired: 1 out]
